vi "squash2016_3.vi"() -> ()   [LabVIEW 2014]
uses:
  <vilib>/vision/Image Controls.llb/IMAQ Image.ctl
  <vilib>/Utility/file.llb/Read From Spreadsheet File (string).vi
  <vilib>/Utility/file.llb/Read From Spreadsheet File (I64).vi
panel:
  in  "Forehand disp 2":bool
  in  "Backhand disp 2":bool
  in  "Cross disp 2":bool
  in  "Bounce disp 2":bool
  in  "Straight disp 2":bool
  in  "volley disp 2":bool
  in  "halfvolley disp 2":bool
  in  "halfvolley disp 1":bool
  in  "volley disp 1":bool
  in  "Straight disp 1":bool
  in  "Bounce disp 1":bool
  in  "Cross disp 1":bool
  in  "Backhand disp 1":bool
  in  "Forehand disp 1":bool
  in  "Let disp 2":bool
  in  "Nolet2 disp":bool
  in  "Stroke2 disp":bool
  in  "Unforced Error2 disp":bool
  in  "Forced Error2 disp":bool
  in  "Unexpected Winner2 disp":bool
  in  "Expected Winner2 disp":bool
  in  "Let disp":bool
  in  "Nolet1 disp":bool
  in  "Stroke1 disp":bool
  in  "Unforced Error1 disp":bool
  in  "Forced Error1 disp":bool
  in  "Unexpected Winner1 disp":bool
  in  "Expected Winner1 disp":bool
  in  "Adrive disp 2":bool
  in  "Smash disp 2":bool
  in  "DSWdrive disp 2":bool
  in  "Lob disp 2":bool
  in  "ASWdrive disp 2":bool
  in  "Ddrive disp 2":bool
  in  "Chop disp 2":bool
  in  "Drop disp 2":bool
  in  "Boast2 disp 2":bool
  in  "Boast3 disp 2":bool
  in  "Stringdisp 2":string
  in  "Adrive disp":bool
  in  "Smash disp":bool
  in  "DSWdrive disp":bool
  in  "Lob disp":bool
  in  "ASWdrive disp":bool
  in  "Ddrive disp":bool
  in  "Chop disp":bool
  in  "Drop disp":bool
  in  "Boast2 disp":bool
  in  "Boast3 disp":bool
  in  "Stringdisp":string
  out "last saved data":i64[](array[numeric])
  out "Btn 10":string
  out "Btn 9":string
  out "Btn 8":string
  out "Btn 7":string
  out "Btn 6":string
  out "subarray":i64[](array[numeric])
  out "output array":i64[][](array[numeric])
  out "appended array":i64[](array[numeric])
  out "0, 1":i16[](array[numeric])
  in  "REPORT":bool
  out "Player 2 data":i64[](array[numeric])
  out "player 1 data":i64[](array[numeric])
  out "both player data":i64[](array[numeric])
  out "Edited data":i64[][](array[numeric])
  out "Event After":i64[][](array[numeric])
  out "Event before":i64[][](array[numeric])
  out "result":i32[](array[numeric])
  out "EVENTS\nTO PLAY":i32[](array[numeric])
  out "Combined data":i64[][](array[numeric])
  out "Extra":i16
  out "Score change":bool[](array[boolean])
  out "last row":i32[](array[numeric])
  out "Player 1/2":i16
  out "Service":i16
  out "Cross":i16
  out "Straight":i16
  out "position":i16
  out "Main tab 2":T1(ring)
  in  "fast rewind":bool
  out "refnum of data save file":refnum<file>
  in  "START":bool
  out "frames to write":i64[][](array[numeric])
  in  "Data file":path=path "C:/Users/KoKuM/Desktop/Current work/ISN/SQUASH/testdata/test2.xls" caption="Data"
  in  "playback speed":dbl(slide)=1.0 min=0.25 max=1.5 step=0.25 scale=0.25..1.5
  in  "Main tab":enum32{"Coding", "Display"}(tab)
  in  "Boast 10":bool
  in  "Boast 12":bool
  in  "Boast 9":bool
  in  "Boast 11":bool
  in  "Smash 12":bool
  in  "Smash 11":bool
  in  "Smash 10":bool
  in  "Smash 9":bool
  in  "lob 12":bool
  in  "Drop 12":bool
  in  "lob 11":bool
  in  "Drop 11":bool
  in  "lob 10":bool
  in  "Drop 10":bool
  in  "lob 9":bool
  in  "Drop 9":bool
  in  "Chop 12":bool
  in  "Chop 11":bool
  in  "Chop 10":bool
  in  "Chop 9":bool
  in  "Smash 8":bool
  in  "Smash 7":bool
  in  "Smash 6":bool
  in  "Smash 5":bool
  in  "Smash":bool
  in  "Smash 2":bool
  in  "Smash 3":bool
  in  "Smash 4":bool
  in  "Chop 8":bool
  in  "Chop 7":bool
  in  "Chop 6":bool
  in  "Chop 5":bool
  in  "Chop":bool
  in  "Chop 2":bool
  in  "Chop 3":bool
  in  "Chop 4":bool
  in  "Boast 7":bool
  in  "Boast 5":bool
  in  "Boast 3":bool
  in  "Boast":bool
  in  "lob 8":bool
  in  "Drop 8":bool
  in  "Boast 6":bool
  in  "lob 7":bool
  in  "Drop 7":bool
  in  "lob 6":bool
  in  "Drop 6":bool
  in  "Boast 8":bool
  in  "lob 5":bool
  in  "Drop 5":bool
  in  "lob 13":bool
  in  "Drop":bool
  in  "Boast 2":bool
  in  "lob 2":bool
  in  "Drop 2":bool
  in  "lob 3":bool
  in  "Drop 3":bool
  in  "Boast 4":bool
  in  "lob 4":bool
  in  "Drop 4":bool
  in  "Let":bool
  in  "Nolet1":bool
  in  "Nolet2":bool
  in  "Stroke1":bool
  in  "Stroke2":bool
  in  "Expected Winner1":bool
  in  "Expected Winner2":bool
  in  "Unexpected Winner1":bool
  in  "Unexpected Winner2":bool
  in  "Forced Error1":bool
  in  "Unforced Error1":bool
  in  "Forced Error2":bool
  in  "Unforced Error2":bool
  in  "Pause lag(s)":dbl=1.0 min=0.0 max=2.0 step=0.5 format="%#.1g"
  in  "Code lag(s)":dbl=1.0 min=0.0 max=5.0 step=0.5 format="%#.1g"
  in  "Link Errors":bool
  in  "Btn 1":string
  in  "Btn 2":string
  in  "Btn 3":string
  in  "Btn 4":string
  in  "Btn 5":string
  in  "Button 1":bool
  in  "Button 2":bool
  in  "Button 3":bool
  in  "Button 4":bool
  in  "Button 5":bool
  out "P2":i32
  out "P1":i32
  out "Player1/Player2":bool[](array[boolean])
  in  "S6":bool
  in  "S5":bool
  in  "S4":bool
  in  "S3":bool
  in  "S2":bool
  in  "Service1":bool
  in  "Service2":bool
  in  "S1":bool
  in  "Player2":bool
  in  "Player1":bool
  in  "Auto switch":bool
  in  "5 4":bool
  in  "5 3":bool
  in  "5 2":bool
  in  "5 1":bool
  in  "6 4":bool
  in  "6 3":bool
  in  "6 2":bool
  in  "6 1":bool
  in  "4 4":bool
  in  "4 3":bool
  in  "4 2":bool
  in  "4 1":bool
  in  "3 4":bool
  in  "3 3":bool
  in  "3 2":bool
  in  "3 1":bool
  in  "2 4":bool
  in  "2 3":bool
  in  "2 2":bool
  in  "2 1":bool
  in  "1 4":bool
  in  "1 3":bool
  in  "1 2":bool
  in  "1 1":bool
  in  "after 2":u8(slide)=2 scale=0.0..5.0
  in  "before 2":u8(slide)=2
  in  "Pause lag on":bool
  in  "SWDrive hide":bool
  in  "SWADrive 12":bool
  in  "SWADrive 11":bool
  in  "SWADrive 10":bool
  in  "SWADrive 9":bool
  in  "SWDDrive 12":bool
  in  "SWDDrive 11":bool
  in  "SWDDrive 10":bool
  in  "SWDDrive 9":bool
  in  "ADrive 12":bool
  in  "ADrive 11":bool
  in  "ADrive 10":bool
  in  "ADrive 9":bool
  in  "DDrive 12":bool
  in  "DDrive 11":bool
  in  "DDrive 10":bool
  in  "DDrive 9":bool
  in  "DDrive 8":bool
  in  "DDrive 7":bool
  in  "DDrive 6":bool
  in  "DDrive 5":bool
  in  "DDrive":bool
  in  "DDrive 2":bool
  in  "DDrive 3":bool
  in  "DDrive 4":bool
  in  "ADrive 8":bool
  in  "ADrive 7":bool
  in  "ADrive 6":bool
  in  "ADrive 5":bool
  in  "ADrive":bool
  in  "ADrive 2":bool
  in  "ADrive 3":bool
  in  "ADrive 4":bool
  in  "SWDDrive 8":bool
  in  "SWDDrive 7":bool
  in  "SWDDrive 6":bool
  in  "SWDDrive 5":bool
  in  "SWDDrive":bool
  in  "SWDDrive 2":bool
  in  "SWDDrive 3":bool
  in  "SWDDrive 4":bool
  in  "SWADrive 8":bool
  in  "SWADrive 7":bool
  in  "SWADrive 6":bool
  in  "SWADrive 5":bool
  in  "SWADrive":bool
  in  "SWADrive 2":bool
  in  "SWADrive 3":bool
  in  "SWADrive 4":bool
  in  "Drive hide":bool
  in  "Undo":bool
  in  "Display tab":enum32{"Edit ", "Data Display"}(tab)
  in  "Extract data":bool
  in  "Upload edited video":bool
  in  "1 10":bool
  in  "1 7":bool
  in  "1 6":bool
  in  "1 5":bool
  in  "2 10":bool
  in  "2 7":bool
  in  "2 6":bool
  in  "2 5":bool
  in  "3 9":bool
  in  "3 7":bool
  in  "3 6":bool
  in  "3 5":bool
  in  "4 9":bool
  in  "4 7":bool
  in  "4 6":bool
  in  "4 5":bool
  in  "Boast3":bool
  in  "Boast2":bool
  in  "Drop 14":bool
  in  "Chop 13":bool
  in  "Ddrive":bool
  in  "Adrive":bool
  in  "ASWdrive":bool
  in  "Lob":bool
  in  "DSWdrive":bool
  in  "Smash 13":bool
  in  "FH":bool
  in  "BH":bool
  in  "ST":bool
  in  "CR":bool
  in  "Bounce":bool
  in  "Half Volley":bool
  in  "Volley":bool
  in  "before":u8(slide)=2
  in  "after":u8(slide)=2 scale=0.0..5.0
  in  "Combine":bool
  in  "Player2 2":bool
  in  "Player1 2":bool
  in  "S6 2":bool
  in  "S5 2":bool
  in  "S4 2":bool
  in  "S1 2":bool
  in  "Service2 2":bool
  in  "Service1 2":bool
  in  "S2 2":bool
  in  "S3 2":bool
  in  "Let 2":bool
  in  "Nolet2 2":bool
  in  "Nolet1 2":bool
  in  "Stroke2 2":bool
  in  "Stroke1 2":bool
  in  "Unforced Error2 2":bool
  in  "Forced Error2 2":bool
  in  "Unforced Error1 2":bool
  in  "Forced Error1 2":bool
  in  "Unexpected Winner2 2":bool
  in  "Unexpected Winner1 2":bool
  in  "Expected Winner2 2":bool
  in  "Expected Winner1 2":bool
  out "Video files to write":string[](array[string])
  in  "Video compress":bool=TRUE
  in  "Abort":bool
  in  "Write file":bool
  in  "Delete":bool[](array[boolean])
  out "Writing":u32(slide) scale=0.0..404.0
  in  "File name":string
  in  "Add to lib":bool
  in  "Video to write":path caption="Folder"
  in  "Examine code":bool
  in  "Update":bool
  in  "Reset":bool
  in  "Code number display":i32 min=1 max=1
  in  "Next":bool
  in  "Previous":bool
  in  "6 5":bool
  in  "6 6":bool
  in  "6 7":bool
  in  "6 8":bool
  in  "5 5":bool
  in  "5 6":bool
  in  "5 7":bool
  in  "5 8":bool
  in  "Button 7":bool
  in  "Button 8":bool
  in  "Button 9":bool
  in  "Button 10":bool
  in  "Button 6":bool
  in  "playback interval on":bool
  in  "Player 2 shots":string[](array[string])=["Att drive", "Def drive", "Att SW drive", "Def SW drive", "", "Drop", "Chop", "Lob", "Boast 2", "Boast 3", "Smash", "", "F-hand", "B-hand", "", "Straight", "Cross", "", "Bounce", "Volley", "H-volley"]
  out "FH 2":u8(slide) scale=0.0..2.0
  out "BH 2":u8(slide) scale=0.0..2.0
  out "Straight 2":u8(slide) scale=0.0..2.0
  out "Cross 2":u8(slide) scale=0.0..2.0
  out "Bounce 2":u8(slide) scale=0.0..2.0
  out "Volley 2":u8(slide) scale=0.0..2.0
  out "Drive 2":u8(slide) scale=0.0..2.0
  out "Lob 2":u8(slide) scale=0.0..2.0
  out "Drop 13":u8(slide) scale=0.0..2.0
  out "Boast 13":u8(slide) scale=0.0..2.0
  out "Player 2 shots numbers":string[](array[string])=["0", "0", "0", "0", "", " ", "0", "0", "", "0", "0", "", "0", "0"]
  in  "Fh 2":string="Forehand"
  in  "BH 4":string="Backhand"
  in  "Cross 6":string="Cross"
  in  "bounce 2":string="Bounce"
  in  "Straight 6":string="Straight"
  in  "volley 2":string="Volley"
  in  "H-volley 2":string="Half volley"
  out "F-hand 2":string="0"
  out "B-hand 2":string="0"
  out "Cross 3":string="0"
  out "Bounce 3":string="0"
  out "Straight 3":string="0"
  out "Volley 3":string="0"
  out "H-volley 3":string="0"
  in  "No let 2":string="No let"
  in  "Let  5":string="Let"
  in  "Stroke 2":string="Stroke"
  out "No Let 2":string="0"
  out "Let 4":string="0"
  out "Stroke 4":string="0"
  in  "ex win2":string="Expected \nwinner"
  in  "UNex win2":string="UNexpected \nwinner"
  in  "F err2":string="Forced \nerror"
  in  "UF err2":string="UNforced \nerror"
  out "ex win2 num":string="0"
  out "UNex win2 num":string="0"
  out "F err2 num":string="0"
  out "UF err2 num":string="0"
  out "4 42":dbl
  out "4 32":dbl
  out "4 22":dbl
  out "4 12":dbl
  out "3 42":dbl
  out "3 32":dbl
  out "3 22":dbl
  out "3 12":dbl
  out "2 42":dbl
  out "2 32":dbl
  out "2 22":dbl
  out "2 12":dbl
  out "1 42":dbl
  out "1 32":dbl
  out "1 22":dbl
  out "1 12":dbl
  in  "H-volley":string="Half volley"
  in  "volley":string="Volley"
  in  "Straight 5":string="Straight"
  in  "bounce":string="Bounce"
  in  "Cross 5":string="Cross"
  in  "BH 3":string="Backhand"
  in  "Fh":string="Forehand"
  in  "No let 1":string="No let"
  in  "Let 1":string="Let "
  in  "Stroke 1":string="Stroke"
  out "No Let 1":string="0"
  out "Let 3":string="0"
  out "Stroke 3":string="0"
  in  "ex win1":string="Expected \nwinner"
  in  "UNex win1":string="Unexpected \nwinner"
  in  "F err1":string="Forced \nerror"
  in  "UF err1":string="UNforced \nerror"
  out "ex win1 num":string="0"
  out "UNex win1 num":string="0"
  out "F err1 num":string="0"
  out "UF err1 num":string="0"
  out "1 14":dbl
  out "1 13":dbl
  out "1 11":dbl
  out "1 9":dbl
  out "2 14":dbl
  out "2 13":dbl
  out "2 11":dbl
  out "2 9":dbl
  out "3 13":dbl
  out "3 11":dbl
  out "3 10":dbl
  out "3 8":dbl
  out "4 13":dbl
  out "4 11":dbl
  out "4 10":dbl
  out "4 8":dbl
  out "H-volley 1":string="0"
  out "F-hand 1":string="0"
  out "B-hand 1":string="0"
  out "Cross 1":string="0"
  out "Bounce 1":string="0"
  out "Straight 1":string="0"
  out "Volley 1":string="0"
  in  "Player 1 shots":string[](array[string])=["Att drive", "Def drive", "Att SW drive", "Def SW drive", "", "Drop", "Chop", "Lob", "Boast 2", "Boast 3", "Smash", "", "F-hand", "B-hand", "", "Straight", "Cross", "", "Bounce", "Volley", "H-volley"]
  out "FH 1":u8(slide) scale=0.0..2.0
  out "BH 1":u8(slide) scale=0.0..2.0
  out "Straight 4":u8(slide) scale=0.0..2.0
  out "Cross 4":u8(slide) scale=0.0..2.0
  out "Bounce 4":u8(slide) scale=0.0..2.0
  out "Volley 4":u8(slide) scale=0.0..2.0
  out "Drive 1":u8(slide) scale=0.0..2.0
  out "Lob 1":u8(slide) scale=0.0..2.0
  out "Drop 1":u8(slide) scale=0.0..2.0
  out "Boast 1":u8(slide) scale=0.0..2.0
  out "Player 1 shots numbers":string[](array[string])=["0", "0", "0", "0", "", " ", "0", "0", "", "0", "0", "", "0", "0"]
  in  "display\nselection":string(combo)="1"
  out "5 14":dbl
  out "5 23":dbl
  out "5 33":dbl
  out "5 43":dbl
  out "6 15":dbl
  out "6 24":dbl
  out "6 34":dbl
  out "6 44":dbl
  out "5 18":dbl
  out "5 15":dbl
  out "5 16":dbl
  out "5 17":dbl
  out "6 18":dbl
  out "6 19":dbl
  out "6 20":dbl
  out "6 21":dbl
  in  "Load video":bool
  in  "Play":bool
  out "ful video frames":i64[](array[numeric])
  out "playback speed":dbl
  out "Number of Frames":u32
  out "framesPerSecond":u32
  out "Last Edit":bool[](array[boolean])
  out "frames 2 play":i64[](array[numeric])
  in  "stop":bool
  out "Video Frame":u32
  out "edited\nevents":i64[][](array[numeric])
  out "edited to play":i64[](array[numeric])
  out "frames edited":i64[](array[numeric])
  in  "fast forward":bool
  in  "Pause":bool
  out "coding":i64[][](array[numeric])
  in  "Progress...":u32(slide) min=400 max=47374 scale=-1.1..130372.0
  in  "Video file":path=path "C:/Users/KoKuM/Desktop/Current work/ISN/SQUASH/testdata/WWC16_FIN_w1.avi" caption="Video"
  out "task":i32(slide) scale=0.0..300.0
  out "Video":T2(plugin-control)
  # "Playback interval (s)"
  # "© 2016 National Sports Institute of Malaysia All Rights Reserved"
  # "Position"
  # "Drop"
  # "Chop"
  # "Lob"
  # "Boast"
  # "Smash"
  # "Att"
  # "Def"
  # "Att"
  # "Def"
  # "Half volley"
  # "Forehand"
  # "Backhand"
  # "St"
  # "Cr"
  # "St"
  # "Cr"
  # "Volley"
  # "Forehand"
  # "Backhand"
  # "St"
  # "Cr"
  # "St"
  # "Cr"
  # "Bounce"
  # "Forehand"
  # "Backhand"
  # "St"
  # "Cr"
  # "St"
  # "Cr"
  # "Lead and lag settings"
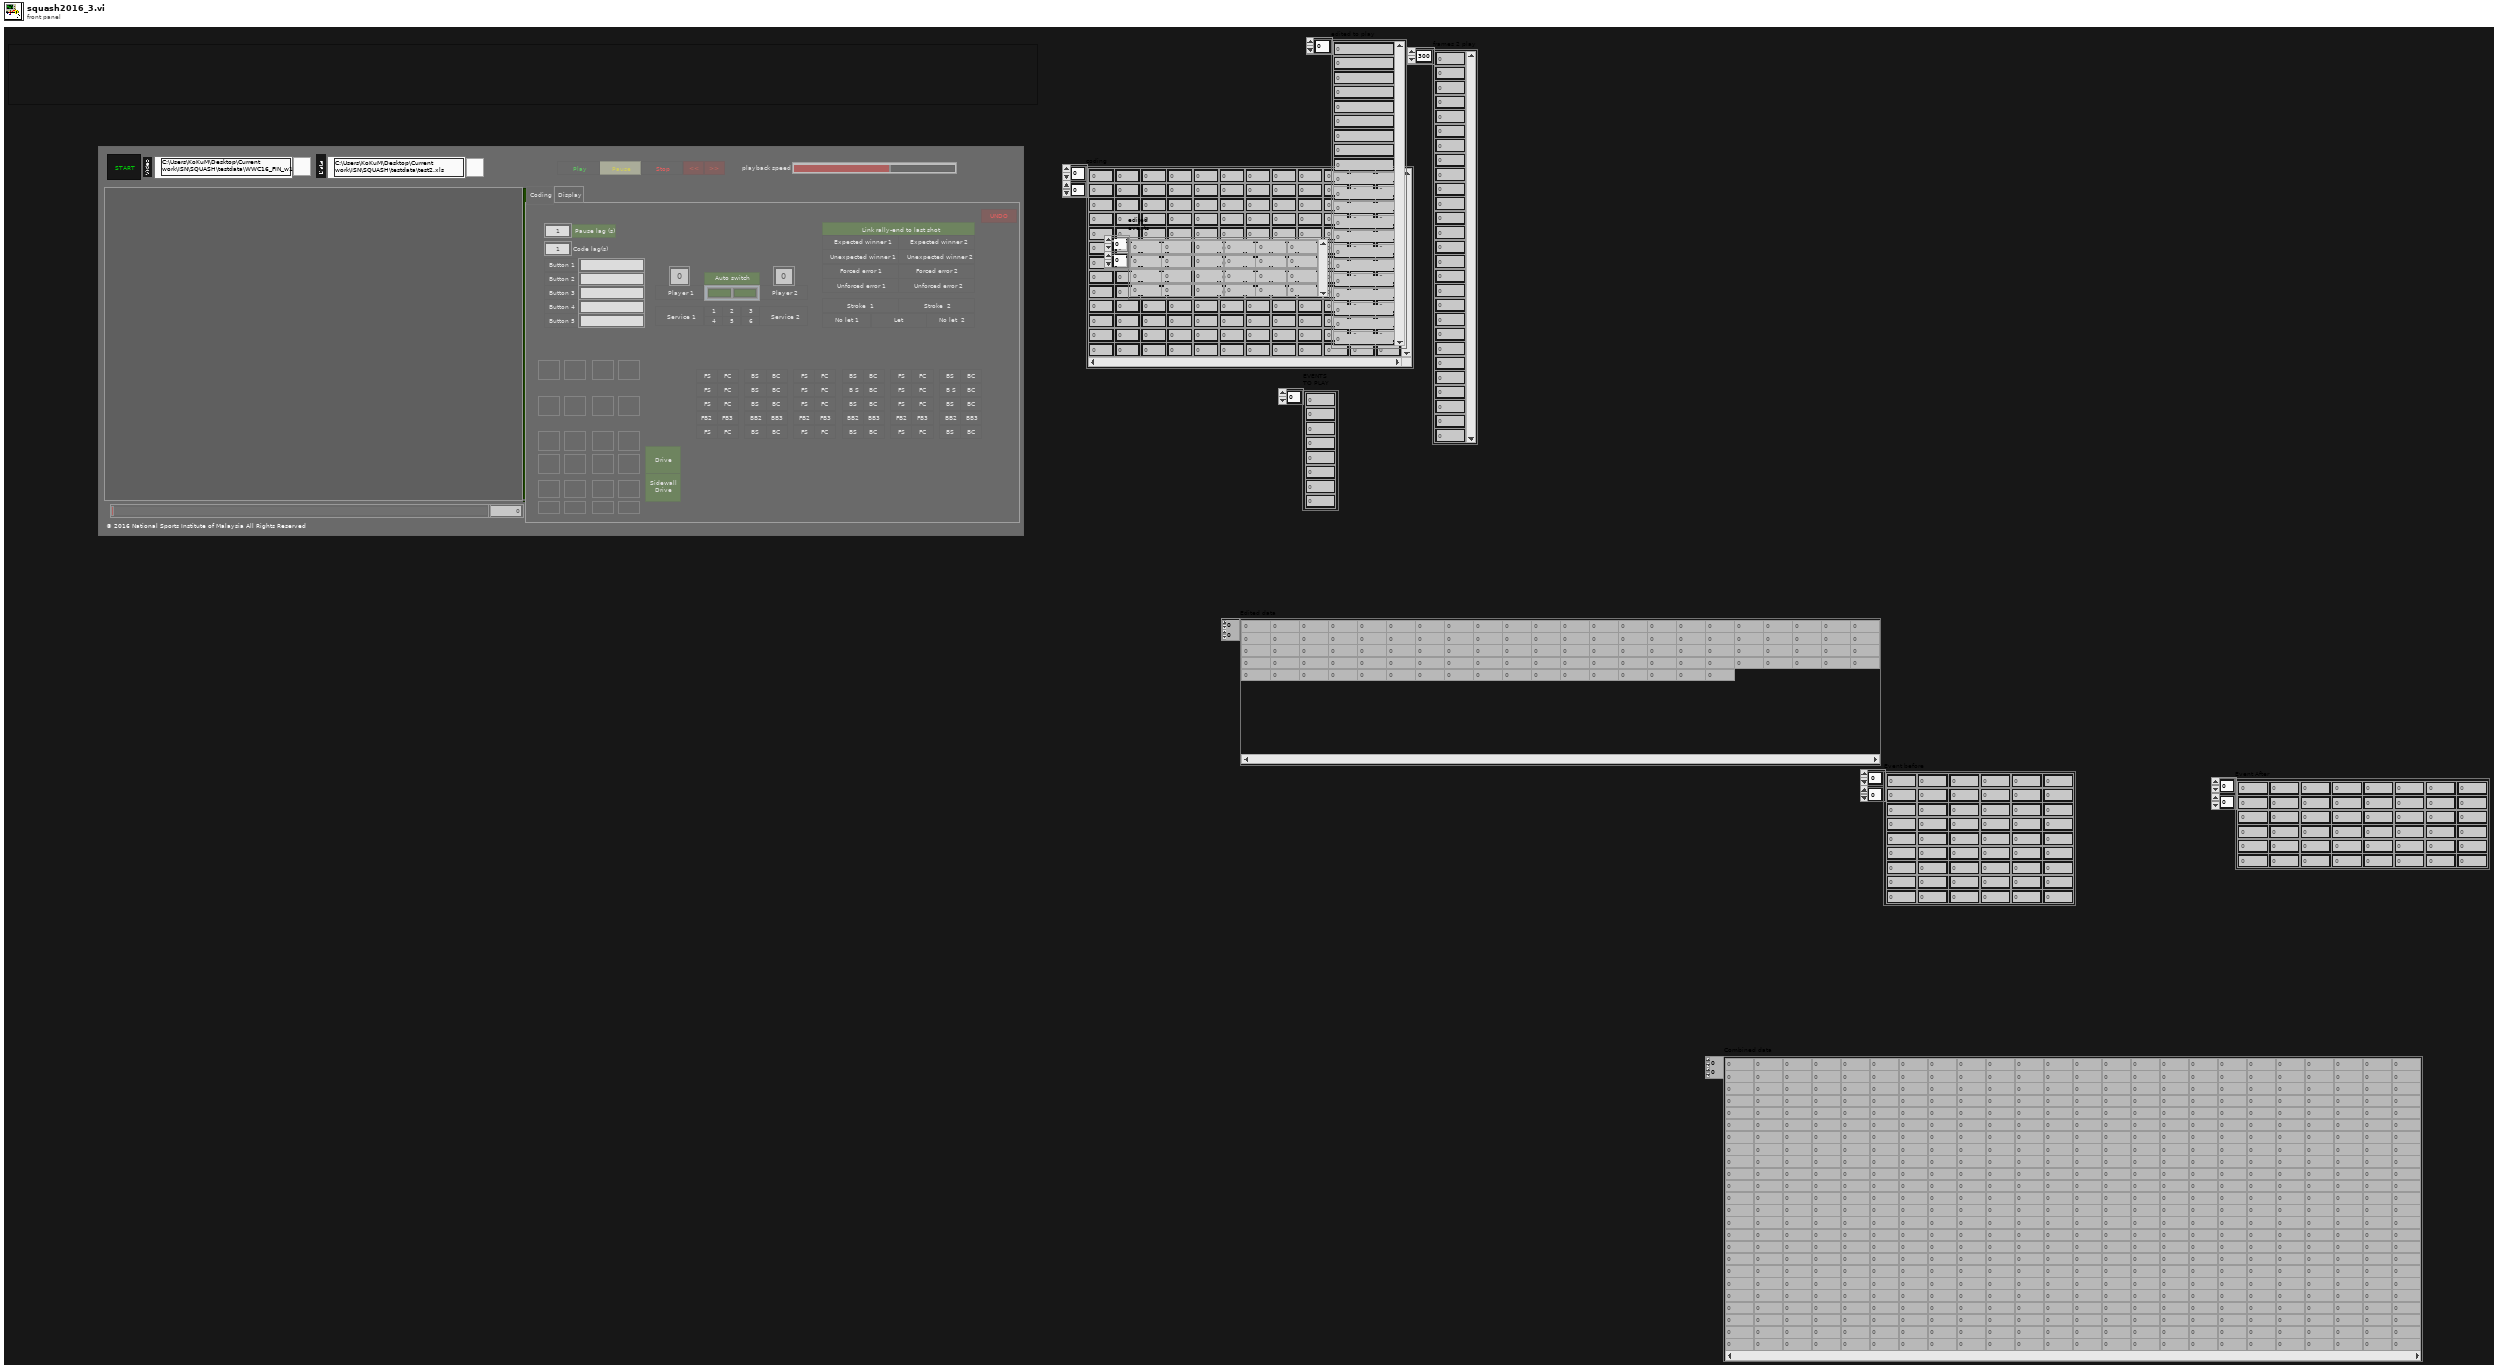
[diagram p1: front panel]
types:
  T1 = enum32{"Coding", "Edit video", "Examine coding", "Display", "Update coding", "Edit coding"}
  T2 = typedef "IMAQ Image.ctl" = refnum<image>
  T3 = enum16{"open", "replace", "create", "open or create", "replace or create", "replace or create with confirmation"}
  T4 = enum8{"Enabled", "Disabled", "Disabled and Grayed Out"}
  T5 = typedef "Image Type" = u32
  T6 = typedef "AviRefnum.ctl" = refnum<k1>
  T7 = cluster{"width":u32, "height":u32, "framesPerSecond":u32, "compressionFilter":string, "hasData":bool}
  T8 = typedef "eventvkey.ctl" = enum16{"ASCII", "Enter", "Return", "Shift", "Ctrl", "Alt", "Cmd", "Opt", "Caps", "NumLock", "Clear", "Break", "Up", "Down", "Left", "Right", "Insert", "Delete", "Home", "End", "PageUp", "PageDown", "Escape", "Help", "Pause", "ScrollLock", "F1", "F2", "F3", "F4", "F5", "F6", "F7", "F8", "F9", "F10", "F11", "F12", "F13", "F14", "F15", "F16", "F17", "F18", "F19", "F20", "F21", "F22", "F23", "F24", "Play", "VolumeUp", "VolumeDown", "Mute", "Two Byte Char"}
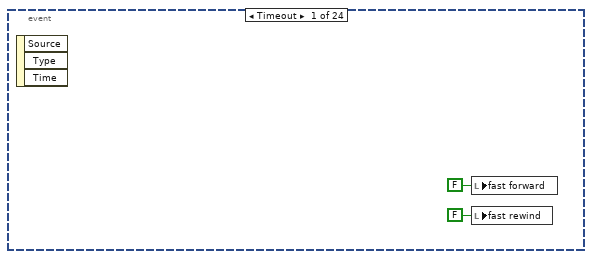
[diagram p3: hidden frame]
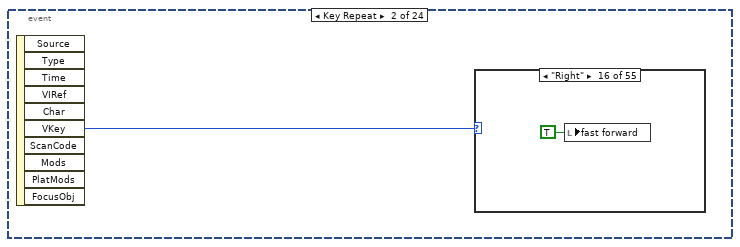
[diagram p4: hidden frame]
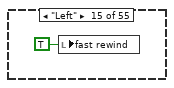
[diagram p19: hidden frame]
diagram:
  n1 = while {
    stop <- FALSE stop-if-true
    n2 = flat-sequence {
      tunnel: [w42] -> w15
      tunnel: [w43] -> w16
      tunnel: w16 -> [w136]
      tunnel: w15 -> [w135]
      tunnel: [w135] -> w14
      tunnel: [w136] -> w13
      tunnel: w14 -> [w176]
      tunnel: w13 -> [w159]
      tunnel: [w175] -> w11
      tunnel: [w158] -> w10
      tunnel: [w157] -> w9
      tunnel: [w156] -> w1
      tunnel: [w155] -> w8
      frame #0 {
        w37 = T4."Enabled" ("Disabled")
        w39 = u32 0 ("Progress...")
        w36 = FALSE ("START")
        w35 = T4."Disabled and Grayed Out" ("Disabled")
        n3 = property on="Play" class="Bool (strict)"("DisabledEnum"=w35, "Value"=w36) -> ()  [unwired: 2 in, 2 out]
        n4 = property on="stop" class="Bool (strict)"("DisabledEnum"=w35, "Value"=w36) -> ()  [unwired: 2 in, 2 out]
        n5 = property on="Pause" class="Bool (strict)"("DisabledEnum"=w35, "Value"=w36) -> ()  [unwired: 2 in, 2 out]
        n6 = property on="fast forward" class="Bool (strict)"("DisabledEnum"=w35, "Value"=w36) -> ()  [unwired: 2 in, 2 out]
        n7 = property on="playback speed" class="Slide (strict)"("DisabledEnum"=w35, "Value"=1.0 ("playback speed")) -> ()  [unwired: 2 in, 2 out]
        n8 = property on="Main tab" class="TabCtl (strict)"("DisabledEnum"=w35, "Value"=enum32{"Coding", "Display"}."Coding" ("Main tab")) -> ()  [unwired: 2 in, 2 out]
        n9 = property on="Progress..." class="Slide (strict)"("DisabledEnum"=w35, "Value"=w39) -> ()  [unwired: 2 in, 2 out]
        n10 = property on="Video Frame" class="DigNum (strict)"("DisabledEnum"=w35, "Value"=w39) -> ()  [unwired: 2 in, 2 out]
        n11 = property on="Video" class="ImageControl"("DisabledEnum"=w35, "Value"=T2 refnum ("Video")) -> ()  [unwired: 2 in, 2 out]
        n12 = property on="START" class="Bool (strict)"("DisabledEnum"=w37, "Value"=w36) -> ()  [unwired: 2 in, 2 out]
        n13 = property on="Video file" class="Path"("DisabledEnum"=w37) -> ()  [unwired: 2 in, 2 out]
        n14 = property on="Data file" class="Path"("DisabledEnum"=w37) -> ()  [unwired: 2 in, 2 out]
        n15 = property on="fast rewind" class="Bool (strict)"("DisabledEnum"=w35, "Value"=w36) -> ()  [unwired: 2 in, 2 out]
      }
      frame #1 {
        n16 = while {
          tunnel: [w45] -> w43
          tunnel: [w44] -> w42
          stop <- w46 stop-if-true
          n17 = case shown="True" "START" {
            tunnel: [FALSE w51] -> w46
            tunnel: [w48 w54] -> w45
            tunnel: [w48 w53] -> w44
            frame False {
              w48 = path "" ("dup path")
              n18 = Wait (ms)(milliseconds to wait=u32 200) -> ()  [unwired: 1 out]
            }
            frame True {
              n19 = Path To String(path="Data file") -> (string=w63:string)
              n20 = Wait (ms)(milliseconds to wait=u32 200) -> ()  [unwired: 1 out]
              n21 = Empty String/Path?(string/path=w63) -> (empty?=w62:bool)
              n22 = case shown="False" w62 {
                tunnel: "Data file" -> [w84 w109]
                tunnel: [w83 FALSE] -> w60
                tunnel: [w82 w109] -> w53
                frame False {
                  n23 = Strip Path(path=w84) -> (stripped path=w89:path)  [unwired: 1 out]
                  n24 = Path To String(path=w89) -> (string=w88:string)
                  n25 = call <vilib>:"Get File Extension.vi"("file"=w84) -> ("filename without extension"=w91:string)  [unwired: 7 in, 3 out]
                  n26 = Concatenate Strings(w88, "\\" ("string"), w91, ".xls" ("string")) -> (w90:string)
                  n27 = String To Path(string=w90) -> (path=w85:path)
                  n28 = call <vilib>:"Check if File or Folder Exists.vi"("path"=w85) -> ("file or folder exists?"=w86:bool)  [unwired: 8 in, 2 out]
                  n29 = case shown="True" w86 {
                    selector: w86 -> [_ w108]
                    tunnel: w85 -> [w95 w107]
                    tunnel: [w94 w108] -> w83
                    tunnel: [w93 w107] -> w82
                    frame False {
                      n30 = Two Button Dialog(message="This data file does not exist.\nDo you wish to start a new project?", 1:"No" ("F button name (\"Cancel\")"), 2:"Yes" ("T button name (\"OK\")")) -> (T button?=w96:bool)
                      n31 = case shown="False" w96 {
                        selector: w96 -> [w101 w103]
                        tunnel: w95 -> [_ w102]
                        tunnel: [w101 w103] -> w94
                        tunnel: [path "" ("dup path") w102] -> w93
                        frame False {
                        }
                        frame True {
                          n32 = Open/Create/Replace File(file path (use dialog)=w102, operation (0:open)=T3."create") -> (refnum out=w104:refnum<file>, error out=w106:errorcluster)  [unwired: 4 in, 1 out]
                          n33 = Close File(refnum=w104, error in=w106) -> ()  [unwired: 2 out]
                        }
                      }
                    }
                    frame True {
                    }
                  }
                }
                frame True {
                  n34 = One Button Dialog(message="Please enter data file") -> ()  [unwired: 1 in, 1 out]
                }
              }
              n35 = Path To String(path="Video file") -> (string=w58:string)
              n36 = Empty String/Path?(string/path=w58) -> (empty?=w57:bool)
              n37 = case shown="True" w57 {
                selector: w57 -> [_ w81]
                tunnel: "Video file" -> [w68 w79]
                tunnel: [w65 w79] -> w54
                tunnel: [w64 w81] -> w55
                frame False {
                  n38 = call <vilib>:"Check if File or Folder Exists.vi"("path"=w68) -> ("file or folder exists?"=w72:bool, "dup path"=w66:path)  [unwired: 8 in, 1 out]
                  n39 = call <vilib>:"Get File Extension.vi"("file"=w68) -> ("lowercase file extension"=w69:string)  [unwired: 7 in, 3 out]
                  n40 = Not(x=w72) -> (.not. x?=w73:bool)
                  n41 = Not Equal?(x=w69, y="avi" ("lowercase file extension")) -> (x != y?=w71:bool)
                  n42 = Or(x=w73, y=w71) -> (x .or. y?=w67:bool)
                  n43 = case shown="True" w67 {
                    selector: w67 -> [w74 w76]
                    tunnel: w66 -> [w75 _]
                    tunnel: [w75 path "" ("dup path")] -> w65
                    tunnel: [w74 w76] -> w64
                    frame False {
                    }
                    frame True {
                      n44 = One Button Dialog(message="You have chosen an invalid video file for coding\n\nPossible reasons\n1)\tChosen video file format was not AVI\n2)\tChosen video file does not exist") -> ()  [unwired: 1 in, 1 out]
                    }
                  }
                }
                frame True {
                  n45 = One Button Dialog(message="Please enter video file") -> ()  [unwired: 1 in, 1 out]
                }
              }
              n46 = Not(x=w55) -> (.not. x?=w59:bool)
              n47 = local write "Video file"(w54) -> ()
              n48 = And(x=w59, y=w60) -> (x .and. y?=w51:bool)
              n49 = local write "Data file"(w53) -> ()
              n50 = local write "START"(w51) -> ()
            }
          }
        }
      }
      frame #2 {
        w114 = FALSE ("Combine")
        w113 = i64[] [] ("to write")
        w131 = 0 ("P1")
        w116 = FALSE ("4 6")
        w115 = TRUE ("4 6")
        w151 = FALSE ("4 6")
        w149 = TRUE ("Extract data")
        w117 = u8 2 ("before")
        w134 = T4."Disabled and Grayed Out" ("Disabled")
        w154 = u32 0 ("Progress...")
        w137 = FALSE ("START")
        w138 = T4."Enabled" ("Disabled")
        n51 = property on="Play" class="Bool (strict)"("DisabledEnum"=w138, "Value"=w137) -> ()  [unwired: 2 in, 2 out]
        n52 = property on="stop" class="Bool (strict)"("DisabledEnum"=w138, "Value"=w137) -> ()  [unwired: 2 in, 2 out]
        n53 = property on="Pause" class="Bool (strict)"("DisabledEnum"=w138, "Value"=w137) -> ()  [unwired: 2 in, 2 out]
        n54 = property on="fast forward" class="Bool (strict)"("DisabledEnum"=w138, "Value"=w137) -> ()  [unwired: 2 in, 2 out]
        n55 = property on="fast rewind" class="Bool (strict)"("DisabledEnum"=w138, "Value"=w137) -> ()  [unwired: 2 in, 2 out]
        n56 = property on="playback speed" class="Slide (strict)"("DisabledEnum"=w138, "Value"=1.0 ("playback speed")) -> ()  [unwired: 2 in, 2 out]
        n57 = property on="Main tab" class="TabCtl (strict)"("DisabledEnum"=w138, "Value"=enum32{"Coding", "Display"}."Coding" ("Main tab")) -> ()  [unwired: 2 in, 2 out]
        n58 = property on="Progress..." class="Slide (strict)"("DisabledEnum"=w138, "Value"=w154) -> ()  [unwired: 2 in, 2 out]
        n59 = property on="Video Frame" class="DigNum (strict)"("DisabledEnum"=w138, "Value"=w154) -> ()  [unwired: 2 in, 2 out]
        n60 = property on="Video" class="ImageControl"("DisabledEnum"=w138) -> ()  [unwired: 2 in, 2 out]
        n61 = property on="Video file" class="Path"("DisabledEnum"=w134) -> ()  [unwired: 2 in, 2 out]
        n62 = property on="Data file" class="Path"("DisabledEnum"=w134) -> ()  [unwired: 2 in, 2 out]
        n63 = property on="Code number display" class="DigNum (strict)"("DisabledEnum"=w134) -> ()  [unwired: 2 in, 2 out]
        n64 = property on="Next" class="Bool (strict)"("DisabledEnum"=w134) -> ()  [unwired: 2 in, 2 out]
        n65 = property on="Reset" class="Bool (strict)"("DisabledEnum"=w134) -> ()  [unwired: 2 in, 2 out]
        n66 = property on="Update" class="Bool (strict)"("DisabledEnum"=w134) -> ()  [unwired: 2 in, 2 out]
        n67 = property on="Previous" class="Bool (strict)"("DisabledEnum"=w134) -> ()  [unwired: 2 in, 2 out]
        n68 = local write "Pause lag(s)"(1.0 ("Pause lag(s)")) -> ()
        n69 = local write "Code lag(s)"(0.5 ("Code lag(s)")) -> ()
        n70 = local write "Link Errors"(TRUE ("Link Errors")) -> ()
        n71 = local write "SWDrive hide"(w115) -> ()
        n72 = local write "Drive hide"(w115) -> ()
        n73 = local write "Pause lag on"(w115) -> ()
        n74 = local write "playback interval on"(w115) -> ()
        n75 = local write "Auto switch"(w115) -> ()
        n76 = local write "Combine"(w114) -> ()
        n77 = local write "Button 10"(w114) -> ()
        n78 = local write "Undo"(w114) -> ()
        n79 = local write "Button 8"(w114) -> ()
        n80 = local write "Button 9"(w114) -> ()
        n81 = local write "Button 6"(w114) -> ()
        n82 = local write "Button 7"(w114) -> ()
        n83 = local write "Last Edit"(bool[] [FALSE, FALSE, FALSE, FALSE, FALSE, FALSE, FALSE, FALSE, FALSE, FALSE, FALSE, FALSE, FALSE, FALSE, FALSE, FALSE, FALSE, FALSE, FALSE, FALSE, FALSE, FALSE, FALSE, FALSE, FALSE, FALSE, FALSE, FALSE, FALSE, FALSE, FALSE, FALSE, FALSE, FALSE, FALSE, FALSE] ("Last Edit")) -> ()
        n84 = local write "File name"("" ("File name")) -> ()
        n85 = local write "Code number display"(1 ("Code number display")) -> ()
        n86 = local write "Delete"(bool[] [TRUE, TRUE, TRUE, TRUE, TRUE] ("Array 2")) -> ()
        n87 = local write "Video compress"(w149) -> ()
        n88 = local write "Extract data"(w149) -> ()
        n89 = local write "Upload edited video"(w151) -> ()
        n90 = local write "Add to lib"(w151) -> ()
        n91 = local write "Abort"(w151) -> ()
        n92 = local write "Write file"(w151) -> ()
        n93 = local write "REPORT"(w151) -> ()
        n94 = local write "Examine code"(w151) -> ()
        n95 = local write "Update"(w151) -> ()
        n96 = local write "Reset"(w151) -> ()
        n97 = local write "Previous"(w151) -> ()
        n98 = local write "Next"(w151) -> ()
        n99 = local write "before"(w117) -> ()
        n100 = local write "after"(w117) -> ()
        n101 = local write "before 2"(w117) -> ()
        n102 = local write "after 2"(w117) -> ()
        n103 = call-poly <vilib>:"Read From Spreadsheet File.vi"("file path (dialog if empty)"=w135) -> ("all rows"=w123:string[][])  [unwired: 6 in, 4 out]
        n104 = Index Array(array=w123, index (row)=3) -> (element=w125:string[])  [unwired: 1 in]
        n105 = Index Array(array=w125, index #1=71 ("index"), index #2=72 ("index"), index #3=73 ("index"), index #4=74 ("index"), index #5=75 ("index")) -> (element #1=w120:string, element #2=w121:string, element #3=w122:string, element #4=w119:string, element #5=w118:string)
        n106 = local write "display\nselection"("1" ("display\nselection")) -> ()
        n107 = local write "task"(300 ("task")) -> ()
        n108 = local write "Load video"(FALSE ("Pause")) -> ()
        n109 = local write "Video files to write"(string[] [] ("Video files to write")) -> ()
        n110 = local write "frames to write"(i64[][] [] ("to write")) -> ()
        n111 = local write "player 1 data"(w113) -> ()
        n112 = local write "both player data"(w113) -> ()
        n113 = local write "Player 2 data"(w113) -> ()
        n114 = local write "last saved data"(w113) -> ()
        n115 = local write "Btn 1"(w120) -> ()
        n116 = local write "Btn 2"(w121) -> ()
        n117 = local write "Btn 3"(w122) -> ()
        n118 = local write "Btn 4"(w119) -> ()
        n119 = local write "Btn 5"(w118) -> ()
        n120 = local write "P1"(w131) -> ()
        n121 = local write "P2"(w131) -> ()
        n122 = local write "Drop"(w116) -> ()
        n123 = local write "Drop 2"(w116) -> ()
        n124 = local write "Drop 3"(w116) -> ()
        n125 = local write "Drop 4"(w116) -> ()
        n126 = local write "Drop 5"(w116) -> ()
        n127 = local write "Drop 6"(w116) -> ()
        n128 = local write "Drop 7"(w116) -> ()
        n129 = local write "Drop 8"(w116) -> ()
        n130 = local write "Drop 9"(w116) -> ()
        n131 = local write "Drop 10"(w116) -> ()
        n132 = local write "Drop 11"(w116) -> ()
        n133 = local write "Drop 12"(w116) -> ()
        n134 = local write "Chop"(w116) -> ()
        n135 = local write "Chop 2"(w116) -> ()
        n136 = local write "Chop 3"(w116) -> ()
        n137 = local write "Chop 4"(w116) -> ()
        n138 = local write "Chop 5"(w116) -> ()
        n139 = local write "Chop 6"(w116) -> ()
        n140 = local write "Chop 7"(w116) -> ()
        n141 = local write "Chop 8"(w116) -> ()
        n142 = local write "Chop 9"(w116) -> ()
        n143 = local write "Chop 10"(w116) -> ()
        n144 = local write "Chop 11"(w116) -> ()
        n145 = local write "Chop 12"(w116) -> ()
        n146 = local write "Player2 2"(w116) -> ()
        n147 = local write "Player1 2"(w116) -> ()
        n148 = local write "Button 7"(w116) -> ()
        n149 = local write "Button 8"(w116) -> ()
        n150 = local write "Button 9"(w116) -> ()
        n151 = local write "Button 10"(w116) -> ()
        n152 = local write "Button 6"(w116) -> ()
        n153 = local write "S6 2"(w116) -> ()
        n154 = local write "S5 2"(w116) -> ()
        n155 = local write "S4 2"(w116) -> ()
        n156 = local write "S1 2"(w116) -> ()
        n157 = local write "Service2 2"(w116) -> ()
        n158 = local write "Service1 2"(w116) -> ()
        n159 = local write "S2 2"(w116) -> ()
        n160 = local write "S3 2"(w116) -> ()
        n161 = local write "lob 13"(w116) -> ()
        n162 = local write "lob 2"(w116) -> ()
        n163 = local write "lob 3"(w116) -> ()
        n164 = local write "lob 4"(w116) -> ()
        n165 = local write "lob 5"(w116) -> ()
        n166 = local write "lob 6"(w116) -> ()
        n167 = local write "lob 7"(w116) -> ()
        n168 = local write "lob 8"(w116) -> ()
        n169 = local write "lob 9"(w116) -> ()
        n170 = local write "lob 10"(w116) -> ()
        n171 = local write "lob 11"(w116) -> ()
        n172 = local write "lob 12"(w116) -> ()
        n173 = local write "Smash"(w116) -> ()
        n174 = local write "Smash 2"(w116) -> ()
        n175 = local write "Smash 3"(w116) -> ()
        n176 = local write "Smash 4"(w116) -> ()
        n177 = local write "Smash 5"(w116) -> ()
        n178 = local write "Smash 6"(w116) -> ()
        n179 = local write "Smash 7"(w116) -> ()
        n180 = local write "Smash 8"(w116) -> ()
        n181 = local write "Smash 9"(w116) -> ()
        n182 = local write "Smash 10"(w116) -> ()
        n183 = local write "Smash 11"(w116) -> ()
        n184 = local write "Smash 12"(w116) -> ()
        n185 = local write "4 5"(w116) -> ()
        n186 = local write "4 6"(w116) -> ()
        n187 = local write "4 7"(w116) -> ()
        n188 = local write "4 9"(w116) -> ()
        n189 = local write "3 5"(w116) -> ()
        n190 = local write "3 6"(w116) -> ()
        n191 = local write "3 7"(w116) -> ()
        n192 = local write "3 9"(w116) -> ()
        n193 = local write "2 5"(w116) -> ()
        n194 = local write "2 6"(w116) -> ()
        n195 = local write "2 7"(w116) -> ()
        n196 = local write "2 10"(w116) -> ()
        n197 = local write "1 5"(w116) -> ()
        n198 = local write "1 6"(w116) -> ()
        n199 = local write "1 7"(w116) -> ()
        n200 = local write "1 10"(w116) -> ()
        n201 = local write "6 5"(w116) -> ()
        n202 = local write "6 6"(w116) -> ()
        n203 = local write "6 7"(w116) -> ()
        n204 = local write "6 8"(w116) -> ()
        n205 = local write "5 5"(w116) -> ()
        n206 = local write "5 6"(w116) -> ()
        n207 = local write "5 7"(w116) -> ()
        n208 = local write "5 8"(w116) -> ()
        n209 = local write "Half Volley"(w116) -> ()
        n210 = local write "ADrive"(w116) -> ()
        n211 = local write "ADrive 2"(w116) -> ()
        n212 = local write "ADrive 3"(w116) -> ()
        n213 = local write "ADrive 4"(w116) -> ()
        n214 = local write "ADrive 5"(w116) -> ()
        n215 = local write "ADrive 6"(w116) -> ()
        n216 = local write "ADrive 7"(w116) -> ()
        n217 = local write "ADrive 8"(w116) -> ()
        n218 = local write "ADrive 9"(w116) -> ()
        n219 = local write "ADrive 10"(w116) -> ()
        n220 = local write "ADrive 11"(w116) -> ()
        n221 = local write "ADrive 12"(w116) -> ()
        n222 = local write "DDrive"(w116) -> ()
        n223 = local write "DDrive 2"(w116) -> ()
        n224 = local write "DDrive 3"(w116) -> ()
        n225 = local write "DDrive 4"(w116) -> ()
        n226 = local write "DDrive 5"(w116) -> ()
        n227 = local write "DDrive 6"(w116) -> ()
        n228 = local write "DDrive 7"(w116) -> ()
        n229 = local write "DDrive 8"(w116) -> ()
        n230 = local write "DDrive 9"(w116) -> ()
        n231 = local write "DDrive 10"(w116) -> ()
        n232 = local write "DDrive 11"(w116) -> ()
        n233 = local write "DDrive 12"(w116) -> ()
        n234 = local write "Smash 13"(w116) -> ()
        n235 = local write "Boast3"(w116) -> ()
        n236 = local write "DSWdrive"(w116) -> ()
        n237 = local write "Lob"(w116) -> ()
        n238 = local write "ASWdrive"(w116) -> ()
        n239 = local write "Adrive"(w116) -> ()
        n240 = local write "Ddrive"(w116) -> ()
        n241 = local write "Chop 13"(w116) -> ()
        n242 = local write "Drop 14"(w116) -> ()
        n243 = local write "Boast2"(w116) -> ()
        n244 = local write "FH"(w116) -> ()
        n245 = local write "BH"(w116) -> ()
        n246 = local write "ST"(w116) -> ()
        n247 = local write "CR"(w116) -> ()
        n248 = local write "Bounce"(w116) -> ()
        n249 = local write "Volley"(w116) -> ()
        n250 = local write "SWADrive"(w116) -> ()
        n251 = local write "SWADrive 2"(w116) -> ()
        n252 = local write "SWADrive 3"(w116) -> ()
        n253 = local write "SWADrive 4"(w116) -> ()
        n254 = local write "SWADrive 5"(w116) -> ()
        n255 = local write "SWADrive 6"(w116) -> ()
        n256 = local write "SWADrive 7"(w116) -> ()
        n257 = local write "SWADrive 8"(w116) -> ()
        n258 = local write "SWADrive 9"(w116) -> ()
        n259 = local write "SWADrive 10"(w116) -> ()
        n260 = local write "SWADrive 11"(w116) -> ()
        n261 = local write "SWADrive 12"(w116) -> ()
        n262 = local write "SWDDrive"(w116) -> ()
        n263 = local write "SWDDrive 2"(w116) -> ()
        n264 = local write "SWDDrive 3"(w116) -> ()
        n265 = local write "SWDDrive 4"(w116) -> ()
        n266 = local write "SWDDrive 5"(w116) -> ()
        n267 = local write "SWDDrive 6"(w116) -> ()
        n268 = local write "SWDDrive 7"(w116) -> ()
        n269 = local write "SWDDrive 8"(w116) -> ()
        n270 = local write "SWDDrive 9"(w116) -> ()
        n271 = local write "SWDDrive 10"(w116) -> ()
        n272 = local write "SWDDrive 11"(w116) -> ()
        n273 = local write "SWDDrive 12"(w116) -> ()
        n274 = local write "Let 2"(w116) -> ()
        n275 = local write "Nolet2 2"(w116) -> ()
        n276 = local write "Nolet1 2"(w116) -> ()
        n277 = local write "Stroke2 2"(w116) -> ()
        n278 = local write "Stroke1 2"(w116) -> ()
        n279 = local write "Unforced Error2 2"(w116) -> ()
        n280 = local write "Forced Error2 2"(w116) -> ()
        n281 = local write "Unforced Error1 2"(w116) -> ()
        n282 = local write "Forced Error1 2"(w116) -> ()
        n283 = local write "Unexpected Winner2 2"(w116) -> ()
        n284 = local write "Unexpected Winner1 2"(w116) -> ()
        n285 = local write "Expected Winner2 2"(w116) -> ()
        n286 = local write "Expected Winner1 2"(w116) -> ()
        n287 = local write "Boast"(w116) -> ()
        n288 = local write "Boast 2"(w116) -> ()
        n289 = local write "Boast 3"(w116) -> ()
        n290 = local write "Boast 4"(w116) -> ()
        n291 = local write "Boast 5"(w116) -> ()
        n292 = local write "Boast 6"(w116) -> ()
        n293 = local write "Boast 7"(w116) -> ()
        n294 = local write "Boast 8"(w116) -> ()
        n295 = local write "Boast 9"(w116) -> ()
        n296 = local write "Boast 10"(w116) -> ()
        n297 = local write "Boast 11"(w116) -> ()
        n298 = local write "Boast 12"(w116) -> ()
        n299 = local write "4 4"(w116) -> ()
        n300 = local write "4 3"(w116) -> ()
        n301 = local write "4 2"(w116) -> ()
        n302 = local write "4 1"(w116) -> ()
        n303 = local write "3 4"(w116) -> ()
        n304 = local write "3 3"(w116) -> ()
        n305 = local write "3 2"(w116) -> ()
        n306 = local write "3 1"(w116) -> ()
        n307 = local write "2 4"(w116) -> ()
        n308 = local write "2 3"(w116) -> ()
        n309 = local write "2 2"(w116) -> ()
        n310 = local write "2 1"(w116) -> ()
        n311 = local write "1 4"(w116) -> ()
        n312 = local write "1 3"(w116) -> ()
        n313 = local write "1 2"(w116) -> ()
        n314 = local write "1 1"(w116) -> ()
        n315 = local write "5 4"(w116) -> ()
        n316 = local write "5 3"(w116) -> ()
        n317 = local write "5 2"(w116) -> ()
        n318 = local write "5 1"(w116) -> ()
        n319 = local write "6 4"(w116) -> ()
        n320 = local write "6 3"(w116) -> ()
        n321 = local write "6 2"(w116) -> ()
        n322 = local write "6 1"(w116) -> ()
        n323 = local write "S6"(w116) -> ()
        n324 = local write "S5"(w116) -> ()
        n325 = local write "S4"(w116) -> ()
        n326 = local write "S1"(w116) -> ()
        n327 = local write "S2"(w116) -> ()
        n328 = local write "S3"(w116) -> ()
        n329 = local write "Let"(w116) -> ()
        n330 = local write "Unexpected Winner2"(w116) -> ()
        n331 = local write "Unexpected Winner1"(w116) -> ()
        n332 = local write "Expected Winner2"(w116) -> ()
        n333 = local write "Expected Winner1"(w116) -> ()
        n334 = local write "Forced Error2"(w116) -> ()
        n335 = local write "Forced Error1"(w116) -> ()
        n336 = local write "Service2"(w116) -> ()
        n337 = local write "Service1"(w116) -> ()
        n338 = local write "Nolet2"(w116) -> ()
        n339 = local write "Nolet1"(w116) -> ()
        n340 = local write "Stroke2"(w116) -> ()
        n341 = local write "Stroke1"(w116) -> ()
        n342 = local write "Unforced Error2"(w116) -> ()
        n343 = local write "Unforced Error1"(w116) -> ()
        n344 = local write "Button 5"(w116) -> ()
        n345 = local write "Button 4"(w116) -> ()
        n346 = local write "Button 3"(w116) -> ()
        n347 = local write "Button 2"(w116) -> ()
        n348 = local write "Button 1"(w116) -> ()
        "Score change" <- bool[] [FALSE, FALSE] ("Score change")
        "Player1/Player2" <- bool[] [TRUE, FALSE] ("Score change")
      }
      frame #3 {
        w161 = T5 4 items=["Grayscale (U8)", "Grayscale (I16)", "Grayscale (SGL)", "Complex (CSG)", "RGB (U32)", "HSL (U32)", "RGB (U64)"] ("Image Type")
        n349 = Path to Array of Strings(0:w159) -> (2:w172:string[])  [unwired: 1 out]
        n350 = call "IMAQ AVI Open"("AVI Path"=w159) -> ("error out"=w163:errorcluster, "Avi Refnum"=w162:T6)  [unwired: 9 in]
        n351 = Delete From Array(array=w172) -> (array with subset deleted=w173:string[])  [unwired: 2 in, 1 out]
        n352 = call "IMAQ AVI Get Info"("error in (no error)"=w163, "Avi Refnum"=w162) -> ("error out"=w165:errorcluster, "Number of Frames"=w168:u32, "Avi Refnum (duplicate)"=w158:T6, "Frame Data"=w164:T7)  [unwired: 5 in, 1 out]
        "Number of Frames" <- w168
        n353 = Array of Strings to Path(0:w173) -> (2:w174:path)  [unwired: 1 in]
        n354 = call-poly <vilib>:"Read From Spreadsheet File.vi"("file path (dialog if empty)"=w176) -> ("all rows"=w179:i64[][])  [unwired: 6 in, 4 out]
        n355 = Decrement(x=w168) -> (x-1=w171:u32)
        n356 = local write "Video to write"(w174) -> ()
        n357 = Subtract(x=w171, y=200.0) -> (x-y=w169:dbl)
        n358 = Unbundle By Name(w164) -> ("framesPerSecond"=→"framesPerSecond":u32)
        n359 = property on="Progress..." class="Slide (strict)"(error in=w165, "Scale.Maximum"=w171) -> (error out=w166:errorcluster)  [unwired: 1 in, 1 out]
        n360 = Delete From Array(array=w179, length=4, index (row)=0) -> (array with subset deleted=w175:i64[][])  [unwired: 1 in, 1 out]
        n361 = for {
          N: w169 -> [_]
          tunnel: [w183] -> w155 mode=indexing
          i -> [w183]
        }
        "ful video frames" <- w155
        n362 = Index Array(array=w175, index (col)=0 ("disabled index (col)")) -> (element=w181:i64[])  [unwired: 1 in]
        n363 = Array Max & Min(array=w181) -> (max value=w180:i64)  [unwired: 3 out]
        n364 = call "IMAQ Create"("Image Name"="Video", "Image Type"=w161, "error in (no error)"=w166) -> ("New Image"=w157:T2, "error out"=w156:errorcluster)  [unwired: 2 in]
        n365 = local write "Progress..."(w180) -> ()
      }
    }
    n366 = while {
      tunnel: w10 -> [w355]
      tunnel: w9 -> [w354]
      tunnel: w1 -> [w353]
      shift-right: [w347] -> _
      shift-left: w8 -> [w346]
      tunnel: [w330] -> w4
      stop <- w331 continue-if-true
      # "This loop is the video play loop"
      # "1000/playback speed    / frames per sec"
      n367 = while {
        stop <- w371 continue-if-true
        n368 = local read "START"() -> (w370:bool)
        n369 = And(x=w370, y="Pause") -> (x .and. y?=w371:bool)
      }
      n370 = Index Array(array=w346, index="Progress...") -> (element=w333:i64)
      n371 = Array Max & Min(array=w346) -> (max value=w351:i64, max index (indices)=w352:i32)  [unwired: 2 out]
      n372 = while {
        stop <- w360 stop-if-true
        n373 = local read "START"() -> (w357:bool)
        n374 = Not(x=w357) -> (.not. x?=w356:bool)
        n375 = Compound Arithmetic op=OR(w356, "Play", "Load video", "stop") -> (w360:bool)
        n376 = case shown="True" "stop" {
          frame False {
          }
          frame True {
            w362 = FALSE ("Play")
            n377 = local write "stop"(w362) -> ()
            n378 = local write "Play"(w362) -> ()
          }
        }
      }
      n379 = property on="Progress..." class="Slide (strict)"("Scale.Maximum"=w352) -> ()  [unwired: 2 in, 2 out]
      n380 = Increment(x=w333) -> (x+1=w334:i64)
      n381 = Greater Or Equal?(x=w334, y=w351) -> (x >= y?=w337:bool)
      n382 = Select(t=w351, s=w337, f=w333) -> (s? t:f=w348:i64)
      "Video Frame" <- w348
      n383 = call "IMAQ AVI Read Frame"("error in (no error)"=w353, "Frame Number"=w348, "Image"=w354, "Avi Refnum"=w355) -> ("Image Out"=→"Video":T2, "Avi Refnum (duplicate)"=w330:T6)  [unwired: 4 in, 2 out]
      n384 = Search 1D Array(1D array=w346, element=w348) -> ()  [unwired: 1 in, 1 out]
      n385 = Or(x="fast forward", y="fast rewind") -> (x .or. y?=w328:bool)
      n386 = Increment(x="Progress...") -> (x+1=w329:u32)
      n387 = Select(t=1.0, s=w328, f="playback speed") -> (s? t:f=w340:dbl)
      n388 = Increment(x=w329) -> (x+1=w332:u32)
      n389 = local read "framesPerSecond"() -> (w345:u32)
      n390 = Select(t=w332, s="fast forward", f=w329) -> (s? t:f=w324:u32)
      n391 = Subtract(x="Progress...", y=2) -> (x-y=w325:u32)
      n392 = Divide(x=1000.0, y=w340) -> (x/y=w344:dbl)
      n393 = Divide(x=w344, y=w345) -> (x/y=w342:dbl)
      n394 = Select(t=w325, s="fast rewind", f=w324) -> (s? t:f=w323:u32)
      n395 = Round Toward -Infinity(1:w342) -> (0:w341:dbl)
      "playback speed" <- w341
      n396 = Wait (ms)(milliseconds to wait=w341) -> ()  [unwired: 1 out]
      n397 = local read "Load video"() -> (w335:bool)
      n398 = Select(t="Progress...", s=w337, f=w323) -> (s? t:f=w336:u32)
      n399 = case shown="True" w335 {
        tunnel: w346 -> [w363 _]
        tunnel: w336 -> [w364 _]
        tunnel: [w364 w365] -> w350
        tunnel: [w363 w368] -> w347
        frame False {
        }
        frame True {
          n400 = local read "frames 2 play"() -> (w368:i64[])
          n401 = Array Max & Min(array=w368) -> (max index (indices)=w367:i32)  [unwired: 3 out]
          n402 = property on="Progress..." class="Slide (strict)"("Scale.Maximum"=w367) -> ()  [unwired: 2 in, 2 out]
          n403 = local write "Load video"(FALSE ("Play")) -> ()
          n404 = local read "Progress..."() -> (w365:u32)
        }
      }
      n405 = local write "Progress..."(w350) -> ()
      n406 = local read "START"() -> (w331:bool)
    }
    n407 = while {
      shift-right: [w372] -> _
      shift-left: T1."Display" ("Main tab") -> [w373]
      tunnel: w10 -> [w386]
      shift-right: [w376] -> _
      shift-left: w11 -> [w389]
      tunnel: w8 -> [_]
      tunnel: w1 -> [_]
      tunnel: [w374] -> w7
      stop <- w375 continue-if-true
      w379 = T1."Coding" ("Main tab")
      # "Moving to display tab"
      n408 = case shown="\"Edit coding\"" w373 {
        tunnel: w389 -> [w576 w1482 w1740 w2105 w2142 w2277]
        tunnel: [w420 w1482 w1740 w2105 w2142 w2259] -> w376
        tunnel: [T1."Edit video" ("Main tab") w1494 T1."Display" ("Main tab") T1."Edit coding" ("Main tab") w2143 T1."Edit video" ("Main tab")] -> w381
        tunnel: w386 -> [w574 _ _ _ _ _]
        tunnel: [w416 w1487 w1754 w2103 w2140 w2265] -> w374
        frame "Coding", Default {
          n409 = local read "Drop"() -> (w572:bool)
          n410 = local read "Drop 2"() -> (w571:bool)
          n411 = local read "Drop 3"() -> (w570:bool)
          n412 = local read "Drop 4"() -> (w569:bool)
          n413 = local read "Drop 5"() -> (w568:bool)
          n414 = local read "Drop 6"() -> (w567:bool)
          n415 = local read "Drop 7"() -> (w566:bool)
          n416 = local read "Drop 8"() -> (w565:bool)
          n417 = local read "Drop 9"() -> (w564:bool)
          n418 = local read "Drop 10"() -> (w563:bool)
          n419 = local read "Drop 11"() -> (w562:bool)
          n420 = local read "Drop 12"() -> (w561:bool)
          n421 = local read "Chop"() -> (w560:bool)
          n422 = local read "Chop 2"() -> (w559:bool)
          n423 = local read "Chop 3"() -> (w558:bool)
          n424 = local read "Chop 4"() -> (w557:bool)
          n425 = local read "Chop 5"() -> (w556:bool)
          n426 = local read "Chop 6"() -> (w555:bool)
          n427 = local read "Chop 7"() -> (w554:bool)
          n428 = local read "Chop 8"() -> (w553:bool)
          n429 = local read "Chop 9"() -> (w552:bool)
          n430 = local read "Chop 10"() -> (w551:bool)
          n431 = local read "Chop 11"() -> (w550:bool)
          n432 = local read "Chop 12"() -> (w549:bool)
          n433 = local read "Let"() -> (w548:bool)
          n434 = local read "Unexpected Winner2"() -> (w539:bool)
          n435 = local read "Unexpected Winner1"() -> (w538:bool)
          n436 = local read "Expected Winner2"() -> (w537:bool)
          n437 = local read "Expected Winner1"() -> (w536:bool)
          n438 = local read "Forced Error2"() -> (w542:bool)
          n439 = local read "Forced Error1"() -> (w540:bool)
          n440 = local read "Nolet2"() -> (w547:bool)
          n441 = local read "Nolet1"() -> (w546:bool)
          n442 = local read "Stroke2"() -> (w545:bool)
          n443 = local read "Stroke1"() -> (w544:bool)
          n444 = local read "Unforced Error2"() -> (w543:bool)
          n445 = local read "Unforced Error1"() -> (w541:bool)
          n446 = Build Array(w572, w571, w570, w569, w568, w567, w566, w565, w564, w563, w562, w561, w560, w559, w558, w557, w556, w555, w554, w553, w552, w551, w550, w549, w548, w547, w546, w545, w544, w543, w542, w541, w540, w539, w538, w537, w536) -> (w426:bool[])
          n447 = local read "lob 13"() -> (w535:bool)
          n448 = local read "lob 2"() -> (w534:bool)
          n449 = local read "lob 3"() -> (w533:bool)
          n450 = local read "lob 4"() -> (w532:bool)
          n451 = local read "lob 5"() -> (w531:bool)
          n452 = local read "lob 6"() -> (w530:bool)
          n453 = local read "lob 7"() -> (w529:bool)
          n454 = local read "lob 8"() -> (w528:bool)
          n455 = local read "lob 9"() -> (w527:bool)
          n456 = local read "lob 10"() -> (w526:bool)
          n457 = local read "lob 11"() -> (w525:bool)
          n458 = local read "lob 12"() -> (w524:bool)
          n459 = local read "Smash"() -> (w523:bool)
          n460 = local read "Smash 2"() -> (w522:bool)
          n461 = local read "Smash 3"() -> (w521:bool)
          n462 = local read "Smash 4"() -> (w520:bool)
          n463 = local read "Smash 5"() -> (w519:bool)
          n464 = local read "Smash 6"() -> (w518:bool)
          n465 = local read "Smash 7"() -> (w517:bool)
          n466 = local read "Smash 8"() -> (w516:bool)
          n467 = local read "Smash 9"() -> (w515:bool)
          n468 = local read "Smash 10"() -> (w514:bool)
          n469 = local read "Smash 11"() -> (w513:bool)
          n470 = local read "Smash 12"() -> (w512:bool)
          n471 = local read "Boast"() -> (w511:bool)
          n472 = local read "Boast 2"() -> (w510:bool)
          n473 = local read "Boast 3"() -> (w509:bool)
          n474 = local read "Boast 4"() -> (w508:bool)
          n475 = local read "Boast 5"() -> (w507:bool)
          n476 = local read "Boast 6"() -> (w506:bool)
          n477 = local read "Boast 7"() -> (w505:bool)
          n478 = local read "Boast 8"() -> (w504:bool)
          n479 = local read "Boast 9"() -> (w503:bool)
          n480 = local read "Boast 10"() -> (w502:bool)
          n481 = local read "Boast 11"() -> (w501:bool)
          n482 = local read "Boast 12"() -> (w500:bool)
          n483 = Build Array(w535, w534, w533, w532, w531, w530, w529, w528, w527, w526, w525, w524, w523, w522, w521, w520, w519, w518, w517, w516, w515, w514, w513, w512, w511, w510, w509, w508, w507, w506, w505, w504, w503, w502, w501, w500) -> (w425:bool[])
          n484 = local read "Player2"() -> (w417:bool)
          n485 = local read "Player1"() -> (w418:bool)
          n486 = local read "Pause"() -> (w419:bool)
          n487 = local read "ADrive"() -> (w499:bool)
          n488 = local read "ADrive 2"() -> (w498:bool)
          n489 = local read "ADrive 3"() -> (w497:bool)
          n490 = local read "ADrive 4"() -> (w496:bool)
          n491 = local read "ADrive 5"() -> (w495:bool)
          n492 = local read "ADrive 6"() -> (w494:bool)
          n493 = local read "ADrive 7"() -> (w493:bool)
          n494 = local read "ADrive 8"() -> (w492:bool)
          n495 = local read "ADrive 9"() -> (w491:bool)
          n496 = local read "ADrive 10"() -> (w490:bool)
          n497 = local read "ADrive 11"() -> (w489:bool)
          n498 = local read "ADrive 12"() -> (w488:bool)
          n499 = local read "SWADrive"() -> (w487:bool)
          n500 = local read "SWADrive 2"() -> (w486:bool)
          n501 = local read "SWADrive 3"() -> (w485:bool)
          n502 = local read "SWADrive 4"() -> (w484:bool)
          n503 = local read "SWADrive 5"() -> (w483:bool)
          n504 = local read "SWADrive 6"() -> (w482:bool)
          n505 = local read "SWADrive 7"() -> (w481:bool)
          n506 = local read "SWADrive 8"() -> (w480:bool)
          n507 = local read "SWADrive 9"() -> (w479:bool)
          n508 = local read "SWADrive 10"() -> (w478:bool)
          n509 = local read "SWADrive 11"() -> (w477:bool)
          n510 = local read "SWADrive 12"() -> (w476:bool)
          n511 = local read "S6"() -> (w473:bool)
          n512 = local read "S5"() -> (w472:bool)
          n513 = local read "S4"() -> (w471:bool)
          n514 = local read "S1"() -> (w470:bool)
          n515 = local read "S2"() -> (w469:bool)
          n516 = local read "S3"() -> (w468:bool)
          n517 = local read "Service2"() -> (w475:bool)
          n518 = local read "Service1"() -> (w474:bool)
          n519 = Build Array(w499, w498, w497, w496, w495, w494, w493, w492, w491, w490, w489, w488, w487, w486, w485, w484, w483, w482, w481, w480, w479, w478, w477, w476, w475, w474, w473, w472, w471, w470, w469, w468, w419, w418, w417) -> (w424:bool[])
          n520 = local read "DDrive"() -> (w467:bool)
          n521 = local read "DDrive 2"() -> (w466:bool)
          n522 = local read "DDrive 3"() -> (w465:bool)
          n523 = local read "DDrive 4"() -> (w464:bool)
          n524 = local read "DDrive 5"() -> (w463:bool)
          n525 = local read "DDrive 6"() -> (w462:bool)
          n526 = local read "DDrive 7"() -> (w461:bool)
          n527 = local read "DDrive 8"() -> (w460:bool)
          n528 = local read "DDrive 9"() -> (w459:bool)
          n529 = local read "DDrive 10"() -> (w458:bool)
          n530 = local read "DDrive 11"() -> (w457:bool)
          n531 = local read "DDrive 12"() -> (w456:bool)
          n532 = local read "SWDDrive"() -> (w455:bool)
          n533 = local read "SWDDrive 2"() -> (w454:bool)
          n534 = local read "SWDDrive 3"() -> (w453:bool)
          n535 = local read "SWDDrive 4"() -> (w452:bool)
          n536 = local read "SWDDrive 5"() -> (w451:bool)
          n537 = local read "SWDDrive 6"() -> (w450:bool)
          n538 = local read "SWDDrive 7"() -> (w449:bool)
          n539 = local read "SWDDrive 8"() -> (w448:bool)
          n540 = local read "SWDDrive 9"() -> (w447:bool)
          n541 = local read "SWDDrive 10"() -> (w446:bool)
          n542 = local read "SWDDrive 11"() -> (w445:bool)
          n543 = local read "SWDDrive 12"() -> (w444:bool)
          n544 = local read "Button 5"() -> (w415:bool)
          n545 = local read "Button 4"() -> (w414:bool)
          n546 = local read "Button 3"() -> (w413:bool)
          n547 = local read "Button 2"() -> (w412:bool)
          n548 = local read "Button 1"() -> (w411:bool)
          n549 = Build Array(w467, w466, w465, w464, w463, w462, w461, w460, w459, w458, w457, w456, w455, w454, w453, w452, w451, w450, w449, w448, w447, w446, w445, w444) -> (w422:bool[])
          n550 = local read "4 4"() -> (w436:bool)
          n551 = local read "4 3"() -> (w437:bool)
          n552 = local read "4 2"() -> (w438:bool)
          n553 = local read "4 1"() -> (w439:bool)
          n554 = local read "3 4"() -> (w440:bool)
          n555 = local read "3 3"() -> (w441:bool)
          n556 = local read "3 2"() -> (w442:bool)
          n557 = local read "3 1"() -> (w443:bool)
          n558 = local read "2 4"() -> (w435:bool)
          n559 = local read "2 3"() -> (w434:bool)
          n560 = local read "2 2"() -> (w433:bool)
          n561 = local read "2 1"() -> (w432:bool)
          n562 = local read "1 4"() -> (w431:bool)
          n563 = local read "1 3"() -> (w430:bool)
          n564 = local read "1 2"() -> (w429:bool)
          n565 = local read "1 1"() -> (w428:bool)
          n566 = local read "5 4"() -> (w409:bool)
          n567 = local read "5 3"() -> (w408:bool)
          n568 = local read "5 2"() -> (w407:bool)
          n569 = local read "5 1"() -> (w406:bool)
          n570 = local read "6 4"() -> (w405:bool)
          n571 = local read "6 3"() -> (w404:bool)
          n572 = local read "6 2"() -> (w403:bool)
          n573 = local read "6 1"() -> (w402:bool)
          n574 = local read "Undo"() -> (w401:bool)
          n575 = Build Array(w415, w414, w413, w412, w411, w401) -> (w410:bool[])
          n576 = Build Array(w436, w437, w438, w439, w440, w441, w442, w443, w435, w434, w433, w432, w431, w430, w429, w428, w409, w408, w407, w406, w405, w404, w403, w402) -> (w423:bool[])
          n577 = local read "Video Frame"() -> (w573:u32)
          n578 = Build Array(w410, w422, w423, w424, w425, w426) -> (w427:bool[][])
          n579 = Or Array Elements(Boolean array=w427) -> (logical OR=w421:bool)
          n580 = case shown="True" w421 {
            tunnel: w573 -> [_ w739]
            tunnel: w576 -> [w580 w740]
            tunnel: [w580 w603] -> w420
            tunnel: w574 -> [_ w736]
            tunnel: [w577 w632] -> w416
            frame False {
              n581 = local read "Data file"() -> (w578:path)
              n582 = Open/Create/Replace File(file path (use dialog)=w578, operation (0:open)=T3."open") -> (refnum out=w577:refnum<file>)  [unwired: 4 in, 2 out]
            }
            frame True {
              w597 = 0 ("index")
              w607 = "\t"
              w643 = "\r"
              # "extra code buttons\n\nundo button / error button\n\nlink all (extra buttons) to linkshots logic"
              n583 = stacked-sequence {
                tunnel: w740 -> [w764 _ _ _ _ _ _ _ _ _ _ _ _ _ w1430 _]
                tunnel: [w764 _ _ _ _ _ _ _ _ _ _ _ _ _ _ _] -> w601
                tunnel: w739 -> [w770 _ _ _ _ _ _ _ _ _ _ _ _ _ _ _]
                tunnel: [w770 _ _ _ _ _ _ _ _ _ _ _ _ _ _ _] -> w605
                tunnel: w736 -> [w769 _ _ _ _ _ _ _ _ _ _ _ _ _ _ _]
                tunnel: [w766 _ _ _ _ _ _ _ _ _ _ _ _ _ _ _] -> w735
                tunnel: [_ _ "before 2" _ _ _ _ _ _ _ _ _ _ _ _ _] -> w734
                tunnel: [_ _ "after 2" _ _ _ _ _ _ _ _ _ _ _ _ _] -> w733
                tunnel: [_ _ w851 _ _ _ _ _ _ _ _ _ _ _ _ _] -> w732
                tunnel: [_ _ w850 _ _ _ _ _ _ _ _ _ _ _ _ _] -> w731
                tunnel: [_ _ w849 _ _ _ _ _ _ _ _ _ _ _ _ _] -> w730
                tunnel: [_ _ w848 _ _ _ _ _ _ _ _ _ _ _ _ _] -> w729
                tunnel: [_ _ w847 _ _ _ _ _ _ _ _ _ _ _ _ _] -> w728
                tunnel: [_ _ w846 _ _ _ _ _ _ _ _ _ _ _ _ _] -> w727
                tunnel: [_ _ w845 _ _ _ _ _ _ _ _ _ _ _ _ _] -> w726
                tunnel: [_ _ w844 _ _ _ _ _ _ _ _ _ _ _ _ _] -> w725
                tunnel: [_ _ w843 _ _ _ _ _ _ _ _ _ _ _ _ _] -> w724
                tunnel: [_ _ w842 _ _ _ _ _ _ _ _ _ _ _ _ _] -> w723
                tunnel: [_ _ w841 _ _ _ _ _ _ _ _ _ _ _ _ _] -> w722
                tunnel: [_ _ w840 _ _ _ _ _ _ _ _ _ _ _ _ _] -> w721
                tunnel: [_ _ w839 _ _ _ _ _ _ _ _ _ _ _ _ _] -> w720
                tunnel: [_ _ w838 _ _ _ _ _ _ _ _ _ _ _ _ _] -> w719
                tunnel: [_ _ w837 _ _ _ _ _ _ _ _ _ _ _ _ _] -> w718
                tunnel: [_ _ w836 _ _ _ _ _ _ _ _ _ _ _ _ _] -> w717
                tunnel: [_ _ w835 _ _ _ _ _ _ _ _ _ _ _ _ _] -> w716
                tunnel: [_ _ w834 _ _ _ _ _ _ _ _ _ _ _ _ _] -> w715
                tunnel: [_ _ w833 _ _ _ _ _ _ _ _ _ _ _ _ _] -> w714
                tunnel: [_ _ w832 _ _ _ _ _ _ _ _ _ _ _ _ _] -> w713
                tunnel: [_ _ w831 _ _ _ _ _ _ _ _ _ _ _ _ _] -> w712
                tunnel: [_ _ w830 _ _ _ _ _ _ _ _ _ _ _ _ _] -> w711
                tunnel: [_ _ w829 _ _ _ _ _ _ _ _ _ _ _ _ _] -> w710
                tunnel: [_ _ w828 _ _ _ _ _ _ _ _ _ _ _ _ _] -> w709
                tunnel: [_ _ _ w893 _ _ _ _ _ _ _ _ _ _ _ _] -> w708
                tunnel: [_ _ _ w892 _ _ _ _ _ _ _ _ _ _ _ _] -> w707
                tunnel: [_ _ _ w891 _ _ _ _ _ _ _ _ _ _ _ _] -> w706
                tunnel: [_ _ _ w890 _ _ _ _ _ _ _ _ _ _ _ _] -> w705
                tunnel: [_ _ _ _ w948 _ _ _ _ _ _ _ _ _ _ _] -> w704
                tunnel: [_ _ _ _ w947 _ _ _ _ _ _ _ _ _ _ _] -> w703
                tunnel: [_ _ _ _ w946 _ _ _ _ _ _ _ _ _ _ _] -> w702
                tunnel: [_ _ _ _ _ w990 _ _ _ _ _ _ _ _ _ _] -> w701
                tunnel: [_ _ _ _ _ w989 _ _ _ _ _ _ _ _ _ _] -> w700
                tunnel: [_ _ _ _ _ w988 _ _ _ _ _ _ _ _ _ _] -> w699
                tunnel: [_ _ _ _ _ _ w1018 _ _ _ _ _ _ _ _ _] -> w698
                tunnel: [_ _ _ _ _ _ _ w1076 _ _ _ _ _ _ _ _] -> w697
                tunnel: [_ _ _ _ _ _ _ _ w1134 _ _ _ _ _ _ _] -> w696
                tunnel: [_ _ _ _ _ _ _ _ _ w1186 _ _ _ _ _ _] -> w695
                tunnel: [_ _ _ _ _ _ _ _ _ _ w1250 _ _ _ _ _] -> w694
                tunnel: [_ _ _ _ _ _ _ _ _ _ _ w1290 _ _ _ _] -> w693
                tunnel: [_ _ _ _ _ _ _ _ _ _ _ _ w1330 _ _ _] -> w692
                tunnel: [_ _ _ _ _ _ _ _ _ _ _ _ _ _ w1393 _] -> w691
                tunnel: [_ _ _ _ _ _ _ _ _ _ _ _ _ _ w1394 _] -> w690
                tunnel: [_ _ _ _ _ _ _ _ _ _ _ _ _ _ w1395 _] -> w689
                tunnel: [_ _ _ _ _ _ _ _ _ _ _ _ _ _ w1400 _] -> w688
                tunnel: [_ _ _ _ _ _ _ _ _ _ _ _ _ _ w1401 _] -> w687
                tunnel: [_ _ _ _ _ _ _ _ _ _ _ _ _ _ w1402 _] -> w686
                tunnel: [_ _ _ _ _ _ _ _ _ _ _ _ _ _ w1403 _] -> w685
                tunnel: [_ _ _ _ _ _ _ _ _ _ _ _ _ _ w1404 _] -> w684
                tunnel: [_ _ _ _ _ _ _ _ _ _ _ _ _ _ w1405 _] -> w683
                tunnel: [_ _ _ _ _ _ _ _ _ _ _ _ _ _ w1406 _] -> w682
                tunnel: [_ _ _ _ _ _ _ _ _ _ _ _ _ _ w1407 _] -> w681
                tunnel: [_ _ _ _ _ _ _ _ _ _ _ _ _ _ w1408 _] -> w680
                tunnel: [_ _ _ _ _ _ _ _ _ _ _ _ _ _ w1408 _] -> w679
                tunnel: [_ _ _ _ _ _ _ _ _ _ _ _ _ _ w1396 _] -> w678
                tunnel: [_ _ _ _ _ _ _ _ _ _ _ _ _ _ w1397 _] -> w677
                tunnel: [_ _ _ _ _ _ _ _ _ _ _ _ _ _ w1398 _] -> w676
                tunnel: [_ _ _ _ _ _ _ _ _ _ _ _ _ _ w1399 _] -> w675
                tunnel: [_ _ _ _ _ _ _ _ _ _ _ _ _ _ _ w1449] -> w646
                tunnel: [_ _ _ _ _ _ _ _ _ _ _ _ _ w1379 _ _] -> w631
                tunnel: [_ _ _ _ _ _ _ _ _ _ _ _ _ w1378 _ _] -> w630
                tunnel: [_ _ _ _ _ _ _ _ _ _ _ _ _ w1377 _ _] -> w629
                tunnel: [_ _ _ _ _ _ _ _ _ _ _ _ _ w1376 _ _] -> w628
                tunnel: [_ _ _ _ _ _ _ _ _ _ _ _ _ w1375 _ _] -> w627
                tunnel: [_ _ w815 _ _ _ _ _ _ _ _ _ _ _ _ _] -> w619
                tunnel: [_ _ _ _ _ _ _ _ _ _ _ _ _ w1374 _ _] -> w618
                tunnel: [_ _ _ _ _ _ _ _ _ _ _ _ _ w1373 _ _] -> w617
                tunnel: [_ _ _ _ _ _ _ _ _ _ _ _ _ w1372 _ _] -> w616
                tunnel: [_ _ _ _ _ _ _ _ _ _ _ _ _ w1371 _ _] -> w615
                tunnel: [_ _ _ _ _ _ _ _ _ _ _ _ _ w1370 _ _] -> w614
                tunnel: [_ _ w819 _ _ _ _ _ _ _ _ _ _ _ _ _] -> w613
                tunnel: [_ _ w818 _ _ _ _ _ _ _ _ _ _ _ _ _] -> w612
                tunnel: [_ _ w817 _ _ _ _ _ _ _ _ _ _ _ _ _] -> w611
                tunnel: [_ _ w816 _ _ _ _ _ _ _ _ _ _ _ _ _] -> w610
                frame #0 {
                  n584 = local read "Pause"() -> (w765:bool)
                  n585 = And(x=w765, y="Pause lag on") -> (x .and. y?=w768:bool)
                  n586 = case shown="False" w765 {
                    frame False {
                      n587 = Tick Count (ms)() -> (millisecond timer value=w771:u32)
                      n588 = while {
                        tunnel: w771 -> [w783]
                        i -> [w774]
                        stop <- w781 stop-if-true
                        w777 = u32 25 ("milliseconds to wait")
                        n589 = Tick Count (ms)() -> (millisecond timer value=w784:u32)
                        n590 = Subtract(x=w784, y=w783) -> (x-y=w782:u32)
                        n591 = Multiply(x="Code lag(s)", y=1000) -> (x*y=w778:dbl)
                        n592 = Greater Or Equal?(x=w782, y=w778) -> (x >= y?=w781:bool)
                        n593 = Divide(x=w778, y=w777) -> (x/y=w776:dbl)
                        n594 = Divide(x=300.0, y=w776) -> (x/y=w773:dbl)
                        n595 = Multiply(x=w774, y=w773) -> (x*y=→"task":dbl)
                        n596 = Wait (ms)(milliseconds to wait=w777) -> ()  [unwired: 1 out]
                      }
                    }
                    frame True {
                    }
                  }
                  n597 = case shown="True" w768 {
                    tunnel: w770 -> [_ w788]
                    tunnel: w769 -> [_ w790]
                    tunnel: ["pauselag" ("Image Name") w786] -> w766
                    frame False {
                    }
                    frame True {
                      w791 = T5 4 items=["Grayscale (U8)", "Grayscale (I16)", "Grayscale (SGL)", "Complex (CSG)", "RGB (U32)", "HSL (U32)", "RGB (U64)"] ("Image Type")
                      n598 = local read "framesPerSecond"() -> (w797:u32)
                      n599 = local read "Number of Frames"() -> (w787:u32)
                      n600 = Increment(x=w788) -> (x+1=w789:u32)
                      n601 = Multiply(x="Pause lag(s)", y=w797) -> (x*y=w795:dbl)
                      n602 = call "IMAQ Create"("Image Name"="pauselag", "Image Type"=w791) -> ("New Image"=w786:T2, "error out"=w792:errorcluster)  [unwired: 3 in]
                      n603 = Round Toward +Infinity(x=w795) -> (ceil(x): smallest int >= x=w794:dbl)
                      n604 = for {
                        N: w794 -> [_]
                        tunnel: w789 -> [w804]
                        tunnel: w792 -> [w807]
                        tunnel: w786 -> [w806]
                        tunnel: w790 -> [w803]
                        tunnel: w787 -> [w801]
                        i -> [w805]
                        n605 = Add(x=w805, y=w804) -> (x+y=w800:u32)
                        n606 = local read "playback speed"() -> (w798:dbl)
                        n607 = Less Or Equal?(x=w801, y=w800) -> (x <= y?=w802:bool)
                        n608 = Select(t=w801, s=w802, f=w800) -> (s? t:f=w799:u32)
                        n609 = call "IMAQ AVI Read Frame"("error in (no error)"=w807, "Frame Number"=w799, "Image"=w806, "Avi Refnum"=w803) -> ("Image Out"=w808:T2)  [unwired: 4 in, 3 out]
                        n610 = local write "Video"(w808) -> ()
                        n611 = Wait (ms)(milliseconds to wait=w798) -> ()  [unwired: 1 out]
                      }
                    }
                  }
                }
                frame #1 {
                  w809 = i16 0 ("Service")
                  n612 = while {
                    stop <- w810 continue-if-true
                    n613 = local read "START"() -> (w811:bool)
                    n614 = local read "Pause"() -> (w812:bool)
                    n615 = And(x=w811, y=w812) -> (x .and. y?=w810:bool)
                  }
                  n616 = local write "Service"(w809) -> ()
                  n617 = local write "Cross"(w809) -> ()
                  n618 = local write "Straight"(w809) -> ()
                  n619 = local write "position"(w809) -> ()
                  n620 = local write "Player 1/2"(w809) -> ()
                  n621 = local write "Extra"(w809) -> ()
                }
                frame #2 {
                  n622 = local read "Service1"() -> (w859:bool)
                  n623 = local read "Service2"() -> (w861:bool)
                  n624 = Compound Arithmetic op=OR(w859, "Player1", w861, "Player2") -> (w858:bool)
                  n625 = Or(x="Player1", y="Player2") -> (x .or. y?=w864:bool)
                  n626 = case shown="True" w858 {
                    tunnel: w859 -> [_ w887]
                    tunnel: w861 -> [_ w886]
                    tunnel: "Player1" -> [_ w885]
                    tunnel: "Player2" -> [_ w884]
                    frame False {
                    }
                    frame True {
                      n627 = Or(x=w887, y=w885) -> (x .or. y?=w889:bool)
                      n628 = Or(x=w886, y=w884) -> (x .or. y?=w888:bool)
                      n629 = Build Array(w889, w888) -> (w883:bool[])
                      n630 = local write "Player1/Player2"(w883) -> ()
                    }
                  }
                  n631 = Boolean To (0,1)(Boolean=w864) -> (0, 1=→"Player 1/2":i16)
                  n632 = Boolean To (0,1)(Boolean="1 1") -> (0, 1=w851:i16)
                  n633 = Boolean To (0,1)(Boolean="1 2") -> (0, 1=w850:i16)
                  n634 = Boolean To (0,1)(Boolean="1 3") -> (0, 1=w849:i16)
                  n635 = Boolean To (0,1)(Boolean="1 4") -> (0, 1=w848:i16)
                  n636 = Boolean To (0,1)(Boolean="2 1") -> (0, 1=w847:i16)
                  n637 = Boolean To (0,1)(Boolean="2 2") -> (0, 1=w846:i16)
                  n638 = Boolean To (0,1)(Boolean="2 3") -> (0, 1=w845:i16)
                  n639 = Boolean To (0,1)(Boolean="2 4") -> (0, 1=w844:i16)
                  n640 = Boolean To (0,1)(Boolean="3 1") -> (0, 1=w843:i16)
                  n641 = Boolean To (0,1)(Boolean="3 2") -> (0, 1=w842:i16)
                  n642 = Boolean To (0,1)(Boolean="3 3") -> (0, 1=w841:i16)
                  n643 = Boolean To (0,1)(Boolean="3 4") -> (0, 1=w840:i16)
                  n644 = Boolean To (0,1)(Boolean="4 1") -> (0, 1=w839:i16)
                  n645 = Boolean To (0,1)(Boolean="4 2") -> (0, 1=w838:i16)
                  n646 = Boolean To (0,1)(Boolean="4 3") -> (0, 1=w837:i16)
                  n647 = Boolean To (0,1)(Boolean="4 4") -> (0, 1=w836:i16)
                  n648 = Boolean To (0,1)(Boolean="5 1") -> (0, 1=w835:i16)
                  n649 = Boolean To (0,1)(Boolean="5 2") -> (0, 1=w834:i16)
                  n650 = Boolean To (0,1)(Boolean="5 3") -> (0, 1=w833:i16)
                  n651 = Boolean To (0,1)(Boolean="5 4") -> (0, 1=w832:i16)
                  n652 = Boolean To (0,1)(Boolean="6 1") -> (0, 1=w831:i16)
                  n653 = Boolean To (0,1)(Boolean="6 2") -> (0, 1=w830:i16)
                  n654 = Boolean To (0,1)(Boolean="6 3") -> (0, 1=w829:i16)
                  n655 = Boolean To (0,1)(Boolean="6 4") -> (0, 1=w828:i16)
                  n656 = Compound Arithmetic op=OR("1 1", "1 2", "1 3", "1 4", "2 1", "2 2", "2 3", "2 4", "3 1", "3 2", "3 3", "3 4", "4 1", "4 2", "4 3", "4 4", "5 1", "5 2", "5 3", "5 4", "6 1", "6 2", "6 3", "6 4") -> (w882:bool)
                  n657 = Boolean To (0,1)(Boolean=w882) -> (0, 1=→"position":i16)
                  n658 = Boolean To (0,1)(Boolean="Button 1") -> (0, 1=w819:i16)
                  n659 = Boolean To (0,1)(Boolean="Button 2") -> (0, 1=w818:i16)
                  n660 = Boolean To (0,1)(Boolean="Button 3") -> (0, 1=w817:i16)
                  n661 = Boolean To (0,1)(Boolean="Button 4") -> (0, 1=w816:i16)
                  n662 = Boolean To (0,1)(Boolean="Button 5") -> (0, 1=w815:i16)
                  n663 = Compound Arithmetic op=OR(w819, w818, w817, w816, w815) -> (→"Extra":i16)
                }
                frame #3 {
                  n664 = Compound Arithmetic op=OR("ADrive", "ADrive 2", "ADrive 3", "ADrive 4", "ADrive 5", "ADrive 6", "ADrive 7", "ADrive 8", "ADrive 9", "ADrive 10", "ADrive 11", "ADrive 12") -> (w945:bool)
                  n665 = Compound Arithmetic op=OR("SWADrive", "SWADrive 2", "SWADrive 3", "SWADrive 4", "SWADrive 5", "SWADrive 6", "SWADrive 7", "SWADrive 8", "SWADrive 9", "SWADrive 10", "SWADrive 11", "SWADrive 12") -> (w906:bool)
                  n666 = Boolean To (0,1)(Boolean=w945) -> (0, 1=w893:i16)
                  n667 = Boolean To (0,1)(Boolean=w906) -> (0, 1=w891:i16)
                  n668 = Compound Arithmetic op=OR("DDrive", "DDrive 2", "DDrive 3", "DDrive 4", "DDrive 5", "DDrive 6", "DDrive 7", "DDrive 8", "DDrive 9", "DDrive 10", "DDrive 11", "DDrive 12") -> (w932:bool)
                  n669 = Compound Arithmetic op=OR("SWDDrive", "SWDDrive 2", "SWDDrive 3", "SWDDrive 4", "SWDDrive 5", "SWDDrive 6", "SWDDrive 7", "SWDDrive 8", "SWDDrive 9", "SWDDrive 10", "SWDDrive 11", "SWDDrive 12") -> (w919:bool)
                  n670 = Boolean To (0,1)(Boolean=w932) -> (0, 1=w892:i16)
                  n671 = Boolean To (0,1)(Boolean=w919) -> (0, 1=w890:i16)
                }
                frame #4 {
                  n672 = Compound Arithmetic op=OR("Chop", "Chop 2", "Chop 3", "Chop 4", "Chop 5", "Chop 6", "Chop 7", "Chop 8", "Chop 9", "Chop 10", "Chop 11", "Chop 12") -> (w985:bool)
                  n673 = Boolean To (0,1)(Boolean=w985) -> (0, 1=w947:i16)
                  n674 = Compound Arithmetic op=OR("lob 13", "lob 2", "lob 3", "lob 4", "lob 5", "lob 6", "lob 7", "lob 8", "lob 9", "lob 10", "lob 11", "lob 12") -> (w986:bool)
                  n675 = Compound Arithmetic op=OR("Drop", "Drop 2", "Drop 3", "Drop 4", "Drop 5", "Drop 6", "Drop 7", "Drop 8", "Drop 9", "Drop 10", "Drop 11", "Drop 12") -> (w987:bool)
                  n676 = Boolean To (0,1)(Boolean=w987) -> (0, 1=w948:i16)
                  n677 = Boolean To (0,1)(Boolean=w986) -> (0, 1=w946:i16)
                }
                frame #5 {
                  n678 = Compound Arithmetic op=OR("Boast 2", "Boast 4", "Boast 6", "Boast 8", "Boast 10", "Boast 12") -> (w1009:bool)
                  n679 = Boolean To (0,1)(Boolean=w1009) -> (0, 1=w989:i16)
                  n680 = Compound Arithmetic op=OR("Smash", "Smash 2", "Smash 3", "Smash 4", "Smash 5", "Smash 6", "Smash 7", "Smash 8", "Smash 9", "Smash 10", "Smash 11", "Smash 12") -> (w1016:bool)
                  n681 = Compound Arithmetic op=OR("Boast", "Boast 3", "Boast 5", "Boast 7", "Boast 9", "Boast 11") -> (w1017:bool)
                  n682 = Boolean To (0,1)(Boolean=w1017) -> (0, 1=w990:i16)
                  n683 = Boolean To (0,1)(Boolean=w1016) -> (0, 1=w988:i16)
                }
                frame #6 {
                  # "forehand"
                  n684 = local read "Smash 10"() -> (w1052:bool)
                  n685 = local read "Chop 10"() -> (w1064:bool)
                  n686 = local read "Smash 2"() -> (w1056:bool)
                  n687 = local read "Smash 5"() -> (w1055:bool)
                  n688 = local read "Smash 6"() -> (w1054:bool)
                  n689 = local read "Smash 9"() -> (w1053:bool)
                  n690 = local read "Boast 10"() -> (w1046:bool)
                  n691 = local read "Drop 10"() -> (w1070:bool)
                  n692 = local read "Chop 2"() -> (w1068:bool)
                  n693 = local read "Chop 5"() -> (w1067:bool)
                  n694 = local read "Chop 6"() -> (w1066:bool)
                  n695 = local read "Chop 9"() -> (w1065:bool)
                  n696 = local read "Boast 2"() -> (w1050:bool)
                  n697 = local read "Boast 5"() -> (w1049:bool)
                  n698 = local read "Boast 6"() -> (w1048:bool)
                  n699 = local read "Boast 9"() -> (w1047:bool)
                  n700 = local read "Drop 2"() -> (w1074:bool)
                  n701 = local read "Drop 5"() -> (w1073:bool)
                  n702 = local read "Drop 6"() -> (w1072:bool)
                  n703 = local read "Drop 9"() -> (w1071:bool)
                  n704 = local read "Smash"() -> (w1057:bool)
                  n705 = local read "lob 10"() -> (w1058:bool)
                  n706 = local read "Chop"() -> (w1069:bool)
                  n707 = local read "Boast"() -> (w1051:bool)
                  n708 = local read "Drop"() -> (w1075:bool)
                  n709 = local read "lob 2"() -> (w1062:bool)
                  n710 = local read "lob 5"() -> (w1061:bool)
                  n711 = local read "lob 6"() -> (w1060:bool)
                  n712 = local read "lob 9"() -> (w1059:bool)
                  n713 = local read "lob 13"() -> (w1063:bool)
                  n714 = Compound Arithmetic op=OR(w1075, w1074, w1073, w1072, w1071, w1070, w1069, w1068, w1067, w1066, w1065, w1064, w1063, w1062, w1061, w1060, w1059, w1058, w1057, w1056, w1055, w1054, w1053, w1052, w1051, w1050, w1049, w1048, w1047, w1046) -> (w1019:bool)
                  n715 = local read "SWADrive 10"() -> (w1039:bool)
                  n716 = local read "SWDDrive 10"() -> (w1045:bool)
                  n717 = local read "SWADrive 2"() -> (w1035:bool)
                  n718 = local read "SWADrive 5"() -> (w1036:bool)
                  n719 = local read "SWADrive 6"() -> (w1037:bool)
                  n720 = local read "SWADrive 9"() -> (w1038:bool)
                  n721 = local read "SWDDrive 2"() -> (w1041:bool)
                  n722 = local read "SWDDrive 5"() -> (w1042:bool)
                  n723 = local read "SWDDrive 6"() -> (w1043:bool)
                  n724 = local read "SWDDrive 9"() -> (w1044:bool)
                  n725 = local read "SWADrive"() -> (w1034:bool)
                  n726 = local read "SWDDrive"() -> (w1040:bool)
                  n727 = local read "ADrive 10"() -> (w1027:bool)
                  n728 = local read "DDrive 10"() -> (w1033:bool)
                  n729 = local read "ADrive 2"() -> (w1023:bool)
                  n730 = local read "ADrive 5"() -> (w1024:bool)
                  n731 = local read "ADrive 6"() -> (w1025:bool)
                  n732 = local read "ADrive 9"() -> (w1026:bool)
                  n733 = local read "DDrive 2"() -> (w1029:bool)
                  n734 = local read "DDrive 5"() -> (w1030:bool)
                  n735 = local read "DDrive 6"() -> (w1031:bool)
                  n736 = local read "DDrive 9"() -> (w1032:bool)
                  n737 = local read "ADrive"() -> (w1022:bool)
                  n738 = local read "DDrive"() -> (w1028:bool)
                  n739 = Compound Arithmetic op=OR(w1022, w1023, w1024, w1025, w1026, w1027, w1028, w1029, w1030, w1031, w1032, w1033, w1034, w1035, w1036, w1037, w1038, w1039, w1040, w1041, w1042, w1043, w1044, w1045) -> (w1020:bool)
                  n740 = Or(x=w1019, y=w1020) -> (x .or. y?=w1021:bool)
                  n741 = Boolean To (0,1)(Boolean=w1021) -> (0, 1=w1018:i16)
                }
                frame #7 {
                  # "backhand"
                  n742 = local read "Smash 11"() -> (w1108:bool)
                  n743 = local read "Smash 12"() -> (w1107:bool)
                  n744 = local read "Chop 11"() -> (w1120:bool)
                  n745 = local read "Chop 12"() -> (w1119:bool)
                  n746 = local read "Smash 3"() -> (w1112:bool)
                  n747 = local read "Smash 4"() -> (w1111:bool)
                  n748 = local read "Smash 7"() -> (w1110:bool)
                  n749 = local read "Smash 8"() -> (w1109:bool)
                  n750 = local read "Boast 11"() -> (w1102:bool)
                  n751 = local read "Boast 12"() -> (w1101:bool)
                  n752 = local read "Drop 11"() -> (w1126:bool)
                  n753 = local read "Drop 12"() -> (w1125:bool)
                  n754 = local read "Chop 3"() -> (w1124:bool)
                  n755 = local read "Chop 4"() -> (w1123:bool)
                  n756 = local read "Chop 7"() -> (w1122:bool)
                  n757 = local read "Chop 8"() -> (w1121:bool)
                  n758 = local read "Boast 3"() -> (w1106:bool)
                  n759 = local read "Boast 4"() -> (w1105:bool)
                  n760 = local read "Boast 7"() -> (w1104:bool)
                  n761 = local read "Boast 8"() -> (w1103:bool)
                  n762 = local read "Drop 3"() -> (w1130:bool)
                  n763 = local read "Drop 4"() -> (w1129:bool)
                  n764 = local read "Drop 7"() -> (w1128:bool)
                  n765 = local read "Drop 8"() -> (w1127:bool)
                  n766 = local read "lob 11"() -> (w1114:bool)
                  n767 = local read "lob 12"() -> (w1113:bool)
                  n768 = local read "lob 3"() -> (w1118:bool)
                  n769 = local read "lob 4"() -> (w1117:bool)
                  n770 = local read "lob 7"() -> (w1116:bool)
                  n771 = local read "lob 8"() -> (w1115:bool)
                  n772 = Compound Arithmetic op=OR(w1130, w1129, w1128, w1127, w1126, w1125, w1124, w1123, w1122, w1121, w1120, w1119, w1118, w1117, w1116, w1115, w1114, w1113, w1112, w1111, w1110, w1109, w1108, w1107, w1106, w1105, w1104, w1103, w1102, w1101) -> (w1131:bool)
                  n773 = local read "SWADrive 11"() -> (w1084:bool)
                  n774 = local read "SWADrive 12"() -> (w1083:bool)
                  n775 = local read "SWDDrive 11"() -> (w1078:bool)
                  n776 = local read "SWDDrive 12"() -> (w1077:bool)
                  n777 = local read "SWADrive 3"() -> (w1088:bool)
                  n778 = local read "SWADrive 4"() -> (w1087:bool)
                  n779 = local read "SWADrive 7"() -> (w1086:bool)
                  n780 = local read "SWADrive 8"() -> (w1085:bool)
                  n781 = local read "SWDDrive 3"() -> (w1082:bool)
                  n782 = local read "SWDDrive 4"() -> (w1081:bool)
                  n783 = local read "SWDDrive 7"() -> (w1080:bool)
                  n784 = local read "SWDDrive 8"() -> (w1079:bool)
                  n785 = local read "ADrive 11"() -> (w1096:bool)
                  n786 = local read "ADrive 12"() -> (w1095:bool)
                  n787 = local read "DDrive 11"() -> (w1090:bool)
                  n788 = local read "DDrive 12"() -> (w1089:bool)
                  n789 = local read "ADrive 3"() -> (w1100:bool)
                  n790 = local read "ADrive 4"() -> (w1099:bool)
                  n791 = local read "ADrive 7"() -> (w1098:bool)
                  n792 = local read "ADrive 8"() -> (w1097:bool)
                  n793 = local read "DDrive 3"() -> (w1094:bool)
                  n794 = local read "DDrive 4"() -> (w1093:bool)
                  n795 = local read "DDrive 7"() -> (w1092:bool)
                  n796 = local read "DDrive 8"() -> (w1091:bool)
                  n797 = Compound Arithmetic op=OR(w1100, w1099, w1098, w1097, w1096, w1095, w1094, w1093, w1092, w1091, w1090, w1089, w1088, w1087, w1086, w1085, w1084, w1083, w1082, w1081, w1080, w1079, w1078, w1077) -> (w1132:bool)
                  n798 = Or(x=w1131, y=w1132) -> (x .or. y?=w1133:bool)
                  n799 = Boolean To (0,1)(Boolean=w1133) -> (0, 1=w1076:i16)
                }
                frame #8 {
                  # "straight"
                  n800 = local read "Smash 11"() -> (w1159:bool)
                  n801 = local read "Chop 11"() -> (w1171:bool)
                  n802 = local read "Smash 3"() -> (w1163:bool)
                  n803 = local read "Smash 5"() -> (w1162:bool)
                  n804 = local read "Smash 7"() -> (w1161:bool)
                  n805 = local read "Smash 9"() -> (w1160:bool)
                  n806 = local read "Drop 11"() -> (w1177:bool)
                  n807 = local read "Chop 3"() -> (w1175:bool)
                  n808 = local read "Chop 5"() -> (w1174:bool)
                  n809 = local read "Chop 7"() -> (w1173:bool)
                  n810 = local read "Chop 9"() -> (w1172:bool)
                  n811 = local read "Drop 3"() -> (w1181:bool)
                  n812 = local read "Drop 5"() -> (w1180:bool)
                  n813 = local read "Drop 7"() -> (w1179:bool)
                  n814 = local read "Drop 9"() -> (w1178:bool)
                  n815 = local read "Smash"() -> (w1164:bool)
                  n816 = local read "lob 11"() -> (w1165:bool)
                  n817 = local read "Chop"() -> (w1176:bool)
                  n818 = local read "Drop"() -> (w1182:bool)
                  n819 = local read "lob 3"() -> (w1169:bool)
                  n820 = local read "lob 5"() -> (w1168:bool)
                  n821 = local read "lob 7"() -> (w1167:bool)
                  n822 = local read "lob 9"() -> (w1166:bool)
                  n823 = local read "lob 13"() -> (w1170:bool)
                  n824 = Compound Arithmetic op=OR(w1182, w1181, w1180, w1179, w1178, w1177, w1176, w1175, w1174, w1173, w1172, w1171, w1170, w1169, w1168, w1167, w1166, w1165, w1164, w1163, w1162, w1161, w1160, w1159) -> (w1183:bool)
                  n825 = local read "SWADrive 11"() -> (w1141:bool)
                  n826 = local read "SWDDrive 11"() -> (w1135:bool)
                  n827 = local read "SWADrive 3"() -> (w1145:bool)
                  n828 = local read "SWADrive 5"() -> (w1144:bool)
                  n829 = local read "SWADrive 7"() -> (w1143:bool)
                  n830 = local read "SWADrive 9"() -> (w1142:bool)
                  n831 = local read "SWDDrive 3"() -> (w1139:bool)
                  n832 = local read "SWDDrive 5"() -> (w1138:bool)
                  n833 = local read "SWDDrive 7"() -> (w1137:bool)
                  n834 = local read "SWDDrive 9"() -> (w1136:bool)
                  n835 = local read "SWADrive"() -> (w1146:bool)
                  n836 = local read "SWDDrive"() -> (w1140:bool)
                  n837 = local read "ADrive 11"() -> (w1153:bool)
                  n838 = local read "DDrive 11"() -> (w1147:bool)
                  n839 = local read "ADrive 3"() -> (w1157:bool)
                  n840 = local read "ADrive 5"() -> (w1156:bool)
                  n841 = local read "ADrive 7"() -> (w1155:bool)
                  n842 = local read "ADrive 9"() -> (w1154:bool)
                  n843 = local read "DDrive 3"() -> (w1151:bool)
                  n844 = local read "DDrive 5"() -> (w1150:bool)
                  n845 = local read "DDrive 7"() -> (w1149:bool)
                  n846 = local read "DDrive 9"() -> (w1148:bool)
                  n847 = local read "ADrive"() -> (w1158:bool)
                  n848 = local read "DDrive"() -> (w1152:bool)
                  n849 = Compound Arithmetic op=OR(w1158, w1157, w1156, w1155, w1154, w1153, w1152, w1151, w1150, w1149, w1148, w1147, w1146, w1145, w1144, w1143, w1142, w1141, w1140, w1139, w1138, w1137, w1136, w1135) -> (w1184:bool)
                  n850 = Or(x=w1183, y=w1184) -> (x .or. y?=w1185:bool)
                  n851 = Boolean To (0,1)(Boolean=w1185) -> (0, 1=w1134:i16)
                  "Straight" <- w1134
                }
                frame #9 {
                  # "cross"
                  n852 = local read "Smash 10"() -> (w1225:bool)
                  n853 = local read "Smash 12"() -> (w1224:bool)
                  n854 = local read "Chop 10"() -> (w1237:bool)
                  n855 = local read "Chop 12"() -> (w1236:bool)
                  n856 = local read "Smash 2"() -> (w1229:bool)
                  n857 = local read "Smash 4"() -> (w1228:bool)
                  n858 = local read "Smash 6"() -> (w1227:bool)
                  n859 = local read "Smash 8"() -> (w1226:bool)
                  n860 = local read "Boast 10"() -> (w1214:bool)
                  n861 = local read "Boast 11"() -> (w1213:bool)
                  n862 = local read "Boast 12"() -> (w1212:bool)
                  n863 = local read "Drop 10"() -> (w1243:bool)
                  n864 = local read "Drop 12"() -> (w1242:bool)
                  n865 = local read "Chop 2"() -> (w1241:bool)
                  n866 = local read "Chop 4"() -> (w1240:bool)
                  n867 = local read "Chop 6"() -> (w1239:bool)
                  n868 = local read "Chop 8"() -> (w1238:bool)
                  n869 = local read "Boast 2"() -> (w1222:bool)
                  n870 = local read "Boast 3"() -> (w1221:bool)
                  n871 = local read "Boast 4"() -> (w1220:bool)
                  n872 = local read "Boast 5"() -> (w1219:bool)
                  n873 = local read "Boast 6"() -> (w1218:bool)
                  n874 = local read "Boast 7"() -> (w1217:bool)
                  n875 = local read "Boast 8"() -> (w1216:bool)
                  n876 = local read "Boast 9"() -> (w1215:bool)
                  n877 = local read "Drop 2"() -> (w1247:bool)
                  n878 = local read "Drop 4"() -> (w1246:bool)
                  n879 = local read "Drop 6"() -> (w1245:bool)
                  n880 = local read "Drop 8"() -> (w1244:bool)
                  n881 = local read "lob 10"() -> (w1231:bool)
                  n882 = local read "lob 12"() -> (w1230:bool)
                  n883 = local read "Boast"() -> (w1223:bool)
                  n884 = local read "lob 2"() -> (w1235:bool)
                  n885 = local read "lob 4"() -> (w1234:bool)
                  n886 = local read "lob 6"() -> (w1233:bool)
                  n887 = local read "lob 8"() -> (w1232:bool)
                  n888 = Compound Arithmetic op=OR(w1247, w1246, w1245, w1244, w1243, w1242, w1241, w1240, w1239, w1238, w1237, w1236, w1235, w1234, w1233, w1232, w1231, w1230, w1229, w1228, w1227, w1226, w1225, w1224, w1223, w1222, w1221, w1220, w1219, w1218, w1217, w1216, w1215, w1214, w1213, w1212) -> (w1187:bool)
                  n889 = local read "SWADrive 10"() -> (w1195:bool)
                  n890 = local read "SWADrive 12"() -> (w1194:bool)
                  n891 = local read "SWDDrive 10"() -> (w1189:bool)
                  n892 = local read "SWDDrive 12"() -> (w1188:bool)
                  n893 = local read "SWADrive 2"() -> (w1199:bool)
                  n894 = local read "SWADrive 4"() -> (w1198:bool)
                  n895 = local read "SWADrive 6"() -> (w1197:bool)
                  n896 = local read "SWADrive 8"() -> (w1196:bool)
                  n897 = local read "SWDDrive 2"() -> (w1193:bool)
                  n898 = local read "SWDDrive 4"() -> (w1192:bool)
                  n899 = local read "SWDDrive 6"() -> (w1191:bool)
                  n900 = local read "SWDDrive 8"() -> (w1190:bool)
                  n901 = local read "ADrive 10"() -> (w1207:bool)
                  n902 = local read "ADrive 12"() -> (w1206:bool)
                  n903 = local read "DDrive 10"() -> (w1201:bool)
                  n904 = local read "DDrive 12"() -> (w1200:bool)
                  n905 = local read "ADrive 2"() -> (w1211:bool)
                  n906 = local read "ADrive 4"() -> (w1210:bool)
                  n907 = local read "ADrive 6"() -> (w1209:bool)
                  n908 = local read "ADrive 8"() -> (w1208:bool)
                  n909 = local read "DDrive 2"() -> (w1205:bool)
                  n910 = local read "DDrive 4"() -> (w1204:bool)
                  n911 = local read "DDrive 6"() -> (w1203:bool)
                  n912 = local read "DDrive 8"() -> (w1202:bool)
                  n913 = Compound Arithmetic op=OR(w1211, w1210, w1209, w1208, w1207, w1206, w1205, w1204, w1203, w1202, w1201, w1200, w1199, w1198, w1197, w1196, w1195, w1194, w1193, w1192, w1191, w1190, w1189, w1188) -> (w1248:bool)
                  n914 = Or(x=w1187, y=w1248) -> (x .or. y?=w1249:bool)
                  n915 = Boolean To (0,1)(Boolean=w1249) -> (0, 1=w1186:i16)
                  "Cross" <- w1186
                }
                frame #10 {
                  # "bounce"
                  n916 = local read "Smash 2"() -> (w1257:bool)
                  n917 = local read "Smash 3"() -> (w1256:bool)
                  n918 = local read "Smash 4"() -> (w1255:bool)
                  n919 = local read "Chop 2"() -> (w1281:bool)
                  n920 = local read "Chop 3"() -> (w1280:bool)
                  n921 = local read "Chop 4"() -> (w1279:bool)
                  n922 = local read "Boast 2"() -> (w1253:bool)
                  n923 = local read "Boast 3"() -> (w1252:bool)
                  n924 = local read "Boast 4"() -> (w1251:bool)
                  n925 = local read "Drop 2"() -> (w1285:bool)
                  n926 = local read "Drop 3"() -> (w1284:bool)
                  n927 = local read "Drop 4"() -> (w1283:bool)
                  n928 = local read "Smash"() -> (w1258:bool)
                  n929 = local read "Chop"() -> (w1282:bool)
                  n930 = local read "Boast"() -> (w1254:bool)
                  n931 = local read "Drop"() -> (w1286:bool)
                  n932 = local read "lob 2"() -> (w1260:bool)
                  n933 = local read "lob 3"() -> (w1261:bool)
                  n934 = local read "lob 4"() -> (w1259:bool)
                  n935 = local read "lob 13"() -> (w1262:bool)
                  n936 = Compound Arithmetic op=OR(w1286, w1285, w1284, w1283, w1282, w1281, w1280, w1279, w1262, w1260, w1261, w1259, w1258, w1257, w1256, w1255, w1254, w1253, w1252, w1251) -> (w1287:bool)
                  n937 = local read "SWADrive 2"() -> (w1269:bool)
                  n938 = local read "SWADrive 3"() -> (w1268:bool)
                  n939 = local read "SWADrive 4"() -> (w1267:bool)
                  n940 = local read "SWDDrive 2"() -> (w1265:bool)
                  n941 = local read "SWDDrive 3"() -> (w1264:bool)
                  n942 = local read "SWDDrive 4"() -> (w1263:bool)
                  n943 = local read "SWADrive"() -> (w1270:bool)
                  n944 = local read "SWDDrive"() -> (w1266:bool)
                  n945 = local read "ADrive 2"() -> (w1277:bool)
                  n946 = local read "ADrive 3"() -> (w1276:bool)
                  n947 = local read "ADrive 4"() -> (w1275:bool)
                  n948 = local read "DDrive 2"() -> (w1273:bool)
                  n949 = local read "DDrive 3"() -> (w1272:bool)
                  n950 = local read "DDrive 4"() -> (w1271:bool)
                  n951 = local read "ADrive"() -> (w1278:bool)
                  n952 = local read "DDrive"() -> (w1274:bool)
                  n953 = Compound Arithmetic op=OR(w1278, w1277, w1276, w1275, w1274, w1273, w1272, w1271, w1270, w1269, w1268, w1267, w1266, w1265, w1264, w1263) -> (w1288:bool)
                  n954 = Or(x=w1287, y=w1288) -> (x .or. y?=w1289:bool)
                  n955 = Boolean To (0,1)(Boolean=w1289) -> (0, 1=w1250:i16)
                }
                frame #11 {
                  # "volley"
                  n956 = local read "Smash 5"() -> (w1314:bool)
                  n957 = local read "Smash 6"() -> (w1313:bool)
                  n958 = local read "Smash 7"() -> (w1312:bool)
                  n959 = local read "Smash 8"() -> (w1311:bool)
                  n960 = local read "Chop 5"() -> (w1322:bool)
                  n961 = local read "Chop 6"() -> (w1321:bool)
                  n962 = local read "Chop 7"() -> (w1320:bool)
                  n963 = local read "Chop 8"() -> (w1319:bool)
                  n964 = local read "Boast 5"() -> (w1310:bool)
                  n965 = local read "Boast 6"() -> (w1309:bool)
                  n966 = local read "Boast 7"() -> (w1308:bool)
                  n967 = local read "Boast 8"() -> (w1307:bool)
                  n968 = local read "Drop 5"() -> (w1326:bool)
                  n969 = local read "Drop 6"() -> (w1325:bool)
                  n970 = local read "Drop 7"() -> (w1324:bool)
                  n971 = local read "Drop 8"() -> (w1323:bool)
                  n972 = local read "lob 5"() -> (w1318:bool)
                  n973 = local read "lob 6"() -> (w1317:bool)
                  n974 = local read "lob 7"() -> (w1316:bool)
                  n975 = local read "lob 8"() -> (w1315:bool)
                  n976 = Compound Arithmetic op=OR(w1326, w1325, w1324, w1323, w1322, w1321, w1320, w1319, w1318, w1317, w1316, w1315, w1314, w1313, w1312, w1311, w1310, w1309, w1308, w1307) -> (w1327:bool)
                  n977 = local read "SWADrive 5"() -> (w1298:bool)
                  n978 = local read "SWADrive 6"() -> (w1297:bool)
                  n979 = local read "SWADrive 7"() -> (w1296:bool)
                  n980 = local read "SWADrive 8"() -> (w1295:bool)
                  n981 = local read "SWDDrive 5"() -> (w1294:bool)
                  n982 = local read "SWDDrive 6"() -> (w1293:bool)
                  n983 = local read "SWDDrive 7"() -> (w1292:bool)
                  n984 = local read "SWDDrive 8"() -> (w1291:bool)
                  n985 = local read "ADrive 5"() -> (w1306:bool)
                  n986 = local read "ADrive 6"() -> (w1305:bool)
                  n987 = local read "ADrive 7"() -> (w1304:bool)
                  n988 = local read "ADrive 8"() -> (w1303:bool)
                  n989 = local read "DDrive 5"() -> (w1302:bool)
                  n990 = local read "DDrive 6"() -> (w1301:bool)
                  n991 = local read "DDrive 7"() -> (w1300:bool)
                  n992 = local read "DDrive 8"() -> (w1299:bool)
                  n993 = Compound Arithmetic op=OR(w1306, w1305, w1304, w1303, w1302, w1301, w1300, w1299, w1298, w1297, w1296, w1295, w1294, w1293, w1292, w1291) -> (w1328:bool)
                  n994 = Or(x=w1327, y=w1328) -> (x .or. y?=w1329:bool)
                  n995 = Boolean To (0,1)(Boolean=w1329) -> (0, 1=w1290:i16)
                }
                frame #12 {
                  # "half volley"
                  n996 = local read "Smash 10"() -> (w1353:bool)
                  n997 = local read "Smash 11"() -> (w1352:bool)
                  n998 = local read "Smash 12"() -> (w1351:bool)
                  n999 = local read "Chop 10"() -> (w1361:bool)
                  n1000 = local read "Chop 11"() -> (w1360:bool)
                  n1001 = local read "Chop 12"() -> (w1359:bool)
                  n1002 = local read "Smash 9"() -> (w1354:bool)
                  n1003 = local read "Boast 10"() -> (w1349:bool)
                  n1004 = local read "Boast 11"() -> (w1348:bool)
                  n1005 = local read "Boast 12"() -> (w1347:bool)
                  n1006 = local read "Drop 10"() -> (w1365:bool)
                  n1007 = local read "Drop 11"() -> (w1364:bool)
                  n1008 = local read "Drop 12"() -> (w1363:bool)
                  n1009 = local read "Chop 9"() -> (w1362:bool)
                  n1010 = local read "Boast 9"() -> (w1350:bool)
                  n1011 = local read "Drop 9"() -> (w1366:bool)
                  n1012 = local read "lob 10"() -> (w1357:bool)
                  n1013 = local read "lob 11"() -> (w1356:bool)
                  n1014 = local read "lob 12"() -> (w1355:bool)
                  n1015 = local read "lob 9"() -> (w1358:bool)
                  n1016 = Compound Arithmetic op=OR(w1366, w1365, w1364, w1363, w1362, w1361, w1360, w1359, w1358, w1357, w1356, w1355, w1354, w1353, w1352, w1351, w1350, w1349, w1348, w1347) -> (w1367:bool)
                  n1017 = local read "SWADrive 10"() -> (w1337:bool)
                  n1018 = local read "SWADrive 11"() -> (w1336:bool)
                  n1019 = local read "SWADrive 12"() -> (w1335:bool)
                  n1020 = local read "SWDDrive 10"() -> (w1333:bool)
                  n1021 = local read "SWDDrive 11"() -> (w1332:bool)
                  n1022 = local read "SWDDrive 12"() -> (w1331:bool)
                  n1023 = local read "SWADrive 9"() -> (w1338:bool)
                  n1024 = local read "SWDDrive 9"() -> (w1334:bool)
                  n1025 = local read "ADrive 10"() -> (w1345:bool)
                  n1026 = local read "ADrive 11"() -> (w1344:bool)
                  n1027 = local read "ADrive 12"() -> (w1343:bool)
                  n1028 = local read "DDrive 10"() -> (w1341:bool)
                  n1029 = local read "DDrive 11"() -> (w1340:bool)
                  n1030 = local read "DDrive 12"() -> (w1339:bool)
                  n1031 = local read "ADrive 9"() -> (w1346:bool)
                  n1032 = local read "DDrive 9"() -> (w1342:bool)
                  n1033 = Compound Arithmetic op=OR(w1346, w1345, w1344, w1343, w1342, w1341, w1340, w1339, w1338, w1337, w1336, w1335, w1334, w1333, w1332, w1331) -> (w1368:bool)
                  n1034 = Or(x=w1367, y=w1368) -> (x .or. y?=w1369:bool)
                  n1035 = Boolean To (0,1)(Boolean=w1369) -> (0, 1=w1330:i16)
                }
                frame #13 {
                  n1036 = local read "Player1/Player2"() -> (w1380:bool[])
                  n1037 = Index Array(array=w1380) -> (element #1=w1381:bool, element #2=w1382:bool)  [unwired: 2 in]
                  n1038 = Boolean To (0,1)(Boolean=w1382) -> (0, 1=w1370:i16)
                  n1039 = Boolean To (0,1)(Boolean=w1381) -> (0, 1=w1371:i16)
                  n1040 = Compound Arithmetic op=OR("Service1", "Service2", "S1", "S2", "S3", "S4", "S5", "S6") -> (w1392:bool)
                  n1041 = Boolean To (0,1)(Boolean=w1392) -> (0, 1=→"Service":i16)
                  n1042 = Boolean To (0,1)(Boolean="Service1") -> (0, 1=w1379:i16)
                  n1043 = Boolean To (0,1)(Boolean="Service2") -> (0, 1=w1378:i16)
                  n1044 = Boolean To (0,1)(Boolean="S1") -> (0, 1=w1377:i16)
                  n1045 = Boolean To (0,1)(Boolean="S2") -> (0, 1=w1376:i16)
                  n1046 = Boolean To (0,1)(Boolean="S3") -> (0, 1=w1375:i16)
                  n1047 = Boolean To (0,1)(Boolean="S4") -> (0, 1=w1374:i16)
                  n1048 = Boolean To (0,1)(Boolean="S5") -> (0, 1=w1373:i16)
                  n1049 = Boolean To (0,1)(Boolean="S6") -> (0, 1=w1372:i16)
                }
                frame #14 {
                  w1408 = 0 ("disabled index (col)")
                  n1050 = Index Array(array=w1430, index (col) #1=51 ("disabled index (col)"), index (col) #2=52 ("index (col)"), index (col) #3=0 ("index (col)")) -> (element #1=w1419:i64[], element #2=w1418:i64[], element #3=w1421:i64[])  [unwired: 3 in]
                  n1051 = Or(x=w1419, y=w1418) -> (x .or. y?=w1426:i64[])
                  n1052 = Reverse 1D Array(array=w1426) -> (reversed array=w1425:i64[])
                  n1053 = Reverse 1D Array(array=w1421) -> (reversed array=w1423:i64[])
                  n1054 = Compound Arithmetic op=OR("Expected Winner1", "Unexpected Winner1", "Stroke1", "Forced Error2", "Unforced Error2", "Nolet2") -> (w1440:bool)
                  n1055 = Search 1D Array(1D array=w1425, element=i64 1) -> (index of element=w1422:i32)  [unwired: 1 in]
                  n1056 = Boolean To (0,1)(Boolean=w1440) -> (0, 1=w1406:i16)
                  n1057 = Compound Arithmetic op=OR("Expected Winner2", "Unexpected Winner2", "Stroke2", "Forced Error1", "Unforced Error1", "Nolet1") -> (w1439:bool)
                  n1058 = Boolean To (0,1)(Boolean="Expected Winner1") -> (0, 1=w1393:i16)
                  n1059 = Boolean To (0,1)(Boolean="Expected Winner2") -> (0, 1=w1394:i16)
                  n1060 = Boolean To (0,1)(Boolean="Unexpected Winner1") -> (0, 1=w1395:i16)
                  n1061 = Boolean To (0,1)(Boolean="Unexpected Winner2") -> (0, 1=w1396:i16)
                  n1062 = Boolean To (0,1)(Boolean="Stroke1") -> (0, 1=w1397:i16)
                  n1063 = Boolean To (0,1)(Boolean="Stroke2") -> (0, 1=w1398:i16)
                  n1064 = Boolean To (0,1)(Boolean="Forced Error1") -> (0, 1=w1399:i16)
                  n1065 = Boolean To (0,1)(Boolean="Forced Error2") -> (0, 1=w1400:i16)
                  n1066 = Boolean To (0,1)(Boolean="Unforced Error1") -> (0, 1=w1401:i16)
                  n1067 = Boolean To (0,1)(Boolean="Unforced Error2") -> (0, 1=w1402:i16)
                  n1068 = Boolean To (0,1)(Boolean="Nolet1") -> (0, 1=w1403:i16)
                  n1069 = Boolean To (0,1)(Boolean="Nolet2") -> (0, 1=w1404:i16)
                  n1070 = Boolean To (0,1)(Boolean="Let") -> (0, 1=w1405:i16)
                  n1071 = Index Array(array=w1423, index=w1422) -> (element=w1420:i64)
                  n1072 = Boolean To (0,1)(Boolean=w1439) -> (0, 1=w1407:i16)
                  n1073 = Search 1D Array(1D array=w1421, element=w1420) -> (index of element=w1417:i32)  [unwired: 1 in]
                  n1074 = Not Equal To 0?(x=w1406) -> (x != 0?=w1432:bool)
                  n1075 = Not Equal To 0?(x=w1407) -> (x != 0?=w1431:bool)
                  n1076 = Build Array(w1432, w1431) -> (w1409:bool[])
                  n1077 = Index Array(array=w1418, index=w1417) -> (element=w1413:i64)
                  n1078 = Index Array(array=w1419, index=w1417) -> (element=w1414:i64)
                  n1079 = Not Equal To 0?(x=w1414) -> (x != 0?=w1415:bool)
                  n1080 = Not Equal To 0?(x=w1413) -> (x != 0?=w1416:bool)
                  n1081 = Build Array(w1415, w1416) -> (w1410:bool[])
                  n1082 = Select(t=w1410, s="Let", f=w1409) -> (s? t:f=w1412:bool[])
                  n1083 = local write "Score change"(w1412) -> ()
                }
                frame #15 {
                  w1447 = FALSE ("4 6")
                  n1084 = local read "Service"() -> (w1456:i16)
                  n1085 = local read "Cross"() -> (w1455:i16)
                  n1086 = local read "Straight"() -> (w1454:i16)
                  n1087 = local read "position"() -> (w1453:i16)
                  n1088 = local read "Player 1/2"() -> (w1452:i16)
                  n1089 = local read "Extra"() -> (w1451:i16)
                  n1090 = local write "Drop"(w1447) -> ()
                  n1091 = local write "Drop 2"(w1447) -> ()
                  n1092 = local write "Drop 3"(w1447) -> ()
                  n1093 = local write "Drop 4"(w1447) -> ()
                  n1094 = local write "Drop 5"(w1447) -> ()
                  n1095 = local write "Drop 6"(w1447) -> ()
                  n1096 = local write "Drop 7"(w1447) -> ()
                  n1097 = local write "Drop 8"(w1447) -> ()
                  n1098 = local write "Drop 9"(w1447) -> ()
                  n1099 = local write "Drop 10"(w1447) -> ()
                  n1100 = local write "Drop 11"(w1447) -> ()
                  n1101 = local write "Drop 12"(w1447) -> ()
                  n1102 = local write "Chop"(w1447) -> ()
                  n1103 = local write "Chop 2"(w1447) -> ()
                  n1104 = local write "Chop 3"(w1447) -> ()
                  n1105 = local write "Chop 4"(w1447) -> ()
                  n1106 = local write "Chop 5"(w1447) -> ()
                  n1107 = local write "Chop 6"(w1447) -> ()
                  n1108 = local write "Chop 7"(w1447) -> ()
                  n1109 = local write "Chop 8"(w1447) -> ()
                  n1110 = local write "Chop 9"(w1447) -> ()
                  n1111 = local write "Chop 10"(w1447) -> ()
                  n1112 = local write "Chop 11"(w1447) -> ()
                  n1113 = local write "Chop 12"(w1447) -> ()
                  n1114 = Compound Arithmetic op=ADD(w1456, w1455, w1454, w1453, w1452, w1451) -> (w1450:i16)
                  n1115 = Equal To 0?(x=w1450) -> (x = 0?=w1449:bool)
                  n1116 = local write "lob 13"(w1447) -> ()
                  n1117 = local write "lob 2"(w1447) -> ()
                  n1118 = local write "lob 3"(w1447) -> ()
                  n1119 = local write "lob 4"(w1447) -> ()
                  n1120 = local write "lob 5"(w1447) -> ()
                  n1121 = local write "lob 6"(w1447) -> ()
                  n1122 = local write "lob 7"(w1447) -> ()
                  n1123 = local write "lob 8"(w1447) -> ()
                  n1124 = local write "lob 9"(w1447) -> ()
                  n1125 = local write "lob 10"(w1447) -> ()
                  n1126 = local write "lob 11"(w1447) -> ()
                  n1127 = local write "lob 12"(w1447) -> ()
                  n1128 = local write "Smash"(w1447) -> ()
                  n1129 = local write "Smash 2"(w1447) -> ()
                  n1130 = local write "Smash 3"(w1447) -> ()
                  n1131 = local write "Smash 4"(w1447) -> ()
                  n1132 = local write "Smash 5"(w1447) -> ()
                  n1133 = local write "Smash 6"(w1447) -> ()
                  n1134 = local write "Smash 7"(w1447) -> ()
                  n1135 = local write "Smash 8"(w1447) -> ()
                  n1136 = local write "Smash 9"(w1447) -> ()
                  n1137 = local write "Smash 10"(w1447) -> ()
                  n1138 = local write "Smash 11"(w1447) -> ()
                  n1139 = local write "Smash 12"(w1447) -> ()
                  n1140 = case shown="True" "Auto switch" {
                    tunnel: w1449 -> [_ w1457]
                    frame False {
                    }
                    frame True {
                      n1141 = local read "Player1/Player2"() -> (w1463:bool[])
                      n1142 = local read "Player1/Player2"() -> (w1464:bool[])
                      n1143 = Reverse 1D Array(array=w1463) -> (reversed array=w1462:bool[])
                      n1144 = Select(t=w1464, s=w1457, f=w1462) -> (s? t:f=w1458:bool[])
                      n1145 = local read "Score change"() -> (w1460:bool[])
                      n1146 = Or Array Elements(Boolean array=w1460) -> (logical OR=w1461:bool)
                      n1147 = Select(t=w1460, s=w1461, f=w1458) -> (s? t:f=w1459:bool[])
                      n1148 = local write "Player1/Player2"(w1459) -> ()
                    }
                  }
                  n1149 = local write "ADrive"(w1447) -> ()
                  n1150 = local write "ADrive 2"(w1447) -> ()
                  n1151 = local write "ADrive 3"(w1447) -> ()
                  n1152 = local write "ADrive 4"(w1447) -> ()
                  n1153 = local write "ADrive 5"(w1447) -> ()
                  n1154 = local write "ADrive 6"(w1447) -> ()
                  n1155 = local write "ADrive 7"(w1447) -> ()
                  n1156 = local write "ADrive 8"(w1447) -> ()
                  n1157 = local write "ADrive 9"(w1447) -> ()
                  n1158 = local write "ADrive 10"(w1447) -> ()
                  n1159 = local write "ADrive 11"(w1447) -> ()
                  n1160 = local write "ADrive 12"(w1447) -> ()
                  n1161 = local write "DDrive"(w1447) -> ()
                  n1162 = local write "DDrive 2"(w1447) -> ()
                  n1163 = local write "DDrive 3"(w1447) -> ()
                  n1164 = local write "DDrive 4"(w1447) -> ()
                  n1165 = local write "DDrive 5"(w1447) -> ()
                  n1166 = local write "DDrive 6"(w1447) -> ()
                  n1167 = local write "DDrive 7"(w1447) -> ()
                  n1168 = local write "DDrive 8"(w1447) -> ()
                  n1169 = local write "DDrive 9"(w1447) -> ()
                  n1170 = local write "DDrive 10"(w1447) -> ()
                  n1171 = local write "DDrive 11"(w1447) -> ()
                  n1172 = local write "DDrive 12"(w1447) -> ()
                  n1173 = local write "SWADrive"(w1447) -> ()
                  n1174 = local write "SWADrive 2"(w1447) -> ()
                  n1175 = local write "SWADrive 3"(w1447) -> ()
                  n1176 = local write "SWADrive 4"(w1447) -> ()
                  n1177 = local write "SWADrive 5"(w1447) -> ()
                  n1178 = local write "SWADrive 6"(w1447) -> ()
                  n1179 = local write "SWADrive 7"(w1447) -> ()
                  n1180 = local write "SWADrive 8"(w1447) -> ()
                  n1181 = local write "SWADrive 9"(w1447) -> ()
                  n1182 = local write "SWADrive 10"(w1447) -> ()
                  n1183 = local write "SWADrive 11"(w1447) -> ()
                  n1184 = local write "SWADrive 12"(w1447) -> ()
                  n1185 = local write "SWDDrive"(w1447) -> ()
                  n1186 = local write "SWDDrive 2"(w1447) -> ()
                  n1187 = local write "SWDDrive 3"(w1447) -> ()
                  n1188 = local write "SWDDrive 4"(w1447) -> ()
                  n1189 = local write "SWDDrive 5"(w1447) -> ()
                  n1190 = local write "SWDDrive 6"(w1447) -> ()
                  n1191 = local write "SWDDrive 7"(w1447) -> ()
                  n1192 = local write "SWDDrive 8"(w1447) -> ()
                  n1193 = local write "SWDDrive 9"(w1447) -> ()
                  n1194 = local write "SWDDrive 10"(w1447) -> ()
                  n1195 = local write "SWDDrive 11"(w1447) -> ()
                  n1196 = local write "SWDDrive 12"(w1447) -> ()
                  n1197 = local write "Boast"(w1447) -> ()
                  n1198 = local write "Boast 2"(w1447) -> ()
                  n1199 = local write "Boast 3"(w1447) -> ()
                  n1200 = local write "Boast 4"(w1447) -> ()
                  n1201 = local write "Boast 5"(w1447) -> ()
                  n1202 = local write "Boast 6"(w1447) -> ()
                  n1203 = local write "Boast 7"(w1447) -> ()
                  n1204 = local write "Boast 8"(w1447) -> ()
                  n1205 = local write "Boast 9"(w1447) -> ()
                  n1206 = local write "Boast 10"(w1447) -> ()
                  n1207 = local write "Boast 11"(w1447) -> ()
                  n1208 = local write "Boast 12"(w1447) -> ()
                  n1209 = local write "4 4"(w1447) -> ()
                  n1210 = local write "4 3"(w1447) -> ()
                  n1211 = local write "4 2"(w1447) -> ()
                  n1212 = local write "4 1"(w1447) -> ()
                  n1213 = local write "3 4"(w1447) -> ()
                  n1214 = local write "3 3"(w1447) -> ()
                  n1215 = local write "3 2"(w1447) -> ()
                  n1216 = local write "3 1"(w1447) -> ()
                  n1217 = local write "2 4"(w1447) -> ()
                  n1218 = local write "2 3"(w1447) -> ()
                  n1219 = local write "2 2"(w1447) -> ()
                  n1220 = local write "2 1"(w1447) -> ()
                  n1221 = local write "1 4"(w1447) -> ()
                  n1222 = local write "1 3"(w1447) -> ()
                  n1223 = local write "1 2"(w1447) -> ()
                  n1224 = local write "1 1"(w1447) -> ()
                  n1225 = local write "5 4"(w1447) -> ()
                  n1226 = local write "5 3"(w1447) -> ()
                  n1227 = local write "5 2"(w1447) -> ()
                  n1228 = local write "5 1"(w1447) -> ()
                  n1229 = local write "6 4"(w1447) -> ()
                  n1230 = local write "6 3"(w1447) -> ()
                  n1231 = local write "6 2"(w1447) -> ()
                  n1232 = local write "6 1"(w1447) -> ()
                  n1233 = local write "S6"(w1447) -> ()
                  n1234 = local write "S5"(w1447) -> ()
                  n1235 = local write "S4"(w1447) -> ()
                  n1236 = local write "S1"(w1447) -> ()
                  n1237 = local write "S2"(w1447) -> ()
                  n1238 = local write "S3"(w1447) -> ()
                  n1239 = local write "Let"(w1447) -> ()
                  n1240 = local write "Unexpected Winner2"(w1447) -> ()
                  n1241 = local write "Unexpected Winner1"(w1447) -> ()
                  n1242 = local write "Expected Winner2"(w1447) -> ()
                  n1243 = local write "Expected Winner1"(w1447) -> ()
                  n1244 = local write "Forced Error2"(w1447) -> ()
                  n1245 = local write "Forced Error1"(w1447) -> ()
                  n1246 = local write "Service2"(w1447) -> ()
                  n1247 = local write "Service1"(w1447) -> ()
                  n1248 = local write "Nolet2"(w1447) -> ()
                  n1249 = local write "Nolet1"(w1447) -> ()
                  n1250 = local write "Stroke2"(w1447) -> ()
                  n1251 = local write "Stroke1"(w1447) -> ()
                  n1252 = local write "Unforced Error2"(w1447) -> ()
                  n1253 = local write "Unforced Error1"(w1447) -> ()
                  n1254 = local write "Player1"(w1447) -> ()
                  n1255 = local write "Player2"(w1447) -> ()
                  n1256 = local write "Button 5"(w1447) -> ()
                  n1257 = local write "Button 4"(w1447) -> ()
                  n1258 = local write "Button 3"(w1447) -> ()
                  n1259 = local write "Button 2"(w1447) -> ()
                  n1260 = local write "Button 1"(w1447) -> ()
                }
              }
              n1261 = Build Array(w605, w734, w733, w732, w731, w730, w729, w728, w727, w726, w725, w724, w723, w722, w721, w720, w719, w718, w717, w716, w715, w714, w713, w712, w711, w710, w709, w708, w707, w706, w705, w704, w703, w702, w701, w700, w699, w698, w697, w696, w695, w694, w693, w692, w691, w690, w689, w678, w677, w676, w675, w688, w687, w686, w685, w684, w683, w682, w681, w680, w679, w631, w630, w629, w628, w627, w618, w617, w616, w615, w614, w613, w612, w611, w610, w619) -> (w599:u32[])
              n1262 = call "IMAQ Dispose"("Image"=w735) -> ()  [unwired: 5 in, 1 out]
              n1263 = Index Array(array=w601, index (col)=0 ("disabled index (col)")) -> (element=w743:i64[])  [unwired: 1 in]
              n1264 = Delete From Array(array=w599, index=0) -> (array with subset deleted=w659:u32[])  [unwired: 1 in, 1 out]
              n1265 = for {
                tunnel: w743 -> [w761] mode=indexing
                tunnel: w605 -> [w762]
                tunnel: [w761] -> w741 mode=indexing if=w763
                stop <- w763 continue-if-true
                n1266 = Less Or Equal?(x=w761, y=w762) -> (x <= y?=w763:bool)
              }
              n1267 = Delete From Array(array=w659, length=2, index=68) -> (array with subset deleted=w587:u32[])  [unwired: 1 out]
              n1268 = Array Size(array=w741) -> (size(s)=w600:i32)
              n1269 = Delete From Array(array=w587, length=17, index=43) -> (deleted portion=w653:u32[], array with subset deleted=w657:u32[])
              n1270 = Delete From Array(array=w587, length=2, index=0) -> (array with subset deleted=w584:u32[])  [unwired: 1 out]
              n1271 = Decrement(x=w600) -> (x-1=w651:i32)
              n1272 = Array Max & Min(array=w657) -> (max value=w658:u32)  [unwired: 3 out]
              n1273 = Array Max & Min(array=w653) -> (max value=w660:u32)  [unwired: 3 out]
              n1274 = Equal To 0?(x=w658) -> ()  [unwired: 1 out]
              n1275 = Not Equal To 0?(x=w660) -> (x != 0?=w656:bool)
              n1276 = Index Array(array=w601, index (row)=w651) -> (element=w654:i64[])  [unwired: 1 in]
              n1277 = Array Max & Min(array=w584) -> (max value=w737:u32)  [unwired: 3 out]
              n1278 = Compound Arithmetic op=AND(w646, w656, "Link Errors") -> (w602:bool)
              n1279 = Decrement(x=w600) -> (x-1=w647:i32)
              n1280 = Replace Array Subset(array=w654, new element=w653, index=44) -> (w598:i64[])
              n1281 = Equal To 0?(x=w737) -> (x = 0?=w590:bool)
              n1282 = Index Array(array=w598, index=w597) -> (element=w596:i64)
              n1283 = Replace Array Subset(array=w601, new element=w598, index (row)=w647) -> (w650:i64[][])  [unwired: 1 in]
              n1284 = Insert Into Array(array=w601, index (row)=w600, new element=w599) -> (w649:i64[][])  [unwired: 1 in]
              n1285 = Index Array(array=w599, index=w597) -> (element=w595:u32)
              n1286 = Select(t=w650, s=w602, f=w649) -> (s? t:f=w648:i64[][])
              n1287 = Select(t=w596, s=w602, f=w595) -> (s? t:f=w588:i64)
              n1288 = local read "last saved data"() -> (w593:i64[])
              n1289 = Select(t=w601, s=w590, f=w648) -> (s? t:f=w604:i64[][])
              n1290 = Search 1D Array(1D array=w593, element=w588) -> (index of element=w592:i32)  [unwired: 1 in]
              n1291 = Greater Than 0?(x=w592) -> (x > 0?=w591:bool)
              n1292 = Insert Into Array(array=w593, new element=w588) -> (w594:i64[])  [unwired: 1 in]
              n1293 = Or(x=w591, y=w590) -> (x .or. y?=w589:bool)
              n1294 = Select(t=w593, s=w589, f=w594) -> (s? t:f=w582:i64[])
              n1295 = case shown="True" "Undo" {
                tunnel: w604 -> [w745 w747]
                tunnel: [w745 w746] -> w603
                tunnel: w582 -> [w744 w756]
                tunnel: [w744 w749] -> w583
                frame False {
                }
                frame True {
                  n1296 = Reverse 1D Array(array=w756) -> (reversed array=w755:i64[])
                  n1297 = Delete From Array(array=w755, index=0) -> (deleted portion=w751:i64, array with subset deleted=w750:i64[])  [unwired: 1 in]
                  n1298 = Reverse 1D Array(array=w750) -> (reversed array=w749:i64[])
                  n1299 = Index Array(array=w747, index (col)=0 ("disabled index (col)")) -> (element=w752:i64[])  [unwired: 1 in]
                  n1300 = Search 1D Array(1D array=w752, element=w751) -> (index of element=w748:i32)  [unwired: 1 in]
                  n1301 = local write "Undo"(FALSE ("Undo")) -> ()
                  n1302 = Delete From Array(array=w747, index (row)=w748) -> (array with subset deleted=w746:i64[][])  [unwired: 2 in, 1 out]
                }
              }
              "last saved data" <- w583
              n1303 = Concatenate Strings("Btn 1", w607, "Btn 2", w607, "Btn 3", w607, "Btn 4", w607, "Btn 5", w607, "Error" ("String")) -> (w621:string)
              n1304 = for {
                tunnel: string[] ["frame number", "Lead", "Lag", "position 1", "position 2", "position 3", "position 4", "position 5", "position 6", "position 7", "position 8", "position 9", "position 10", "position 11", "position 12", "position 13", "position 14", "position 15", "position 16", "position 17", "position 18", "position 19", "position 20", "position 21", "position 22", "position 23", "position 24", "Drive A", "Drive D", "SW Drive A", "SW Drive D", "drop", "chop", "lob", "boast 2", "boast 3", "smash", "Forehand", "Backhand", "Straight", "Cross", "Bounce", "Half Volley", "Volley", "Expected winner 1", "Expected winner 2", "Unexpected winner 1", "Unexpected winner 2", "Stroke 1", "Stroke 2", "Forced error 1", "Forced error 2", "Unforced error 1", "Unforced error 2", "No let 1", "No let 2", "Let", "point1", "point2", "score1", "score2", "service1", "service2", "s1", "s2", "s3", "s4", "s5", "s6", "player1", "player2"] ("all rows") -> [w760] mode=indexing
                tunnel: [w758] -> w608 mode=indexing
                n1305 = Concatenate Strings(w760, "\t") -> (w758:string)
              }
              n1306 = Index Array(array=w603, index (col)=0 ("disabled index (col)")) -> (element=w672:i64[])  [unwired: 1 in]
              n1307 = local read "Video file"() -> (w640:path)
              n1308 = Index Array(array=w603, index (col) #1=57 ("disabled index (col)"), index (col) #2=58 ("index (col)")) -> (element #1=w668:i64[], element #2=w665:i64[])  [unwired: 2 in]
              n1309 = local read "Data file"() -> (w634:path)
              n1310 = Array Max & Min(array=w672) -> (max index (indices)=w673:i32)  [unwired: 3 out]
              n1311 = Add Array Elements(numeric array=w668) -> (sum=→"P1":i64)
              n1312 = Add Array Elements(numeric array=w665) -> (sum=→"P2":i64)
              n1313 = call <vilib>:"Get File Extension.vi"("file"=w640) -> ("filename without extension"=w642:string)  [unwired: 7 in, 3 out]
              n1314 = Open/Create/Replace File(file path (use dialog)=w634, operation (0:open)=T3."replace") -> (refnum out=w636:refnum<file>, error out=w635:errorcluster)  [unwired: 4 in, 1 out]
              n1315 = Index Array(array=w603, index (row)=w673) -> (element=→"last row":i64[])  [unwired: 1 in]
              n1316 = Concatenate Strings(w608, w621, "\r") -> (w633:string)
              n1317 = Array To Spreadsheet String(delimiter (Tab)="\t" ("delimiter (\\t)"), array=w603, 3:"%.3f" ("format (%.3f)")) -> (spreadsheet string=w645:string)
              n1318 = Concatenate Strings("avi file" ("string"), w643, w642, w643, w643, w633, w645) -> (w644:string)
              n1319 = Write to Text File(file (use dialog)=w636, text=w644, error in=w635) -> (refnum out=w632:refnum<file>)  [unwired: 1 in, 2 out]
            }
          }
          "coding" <- w576
        }
        frame "Display" {
          n1320 = flat-sequence {
            tunnel: [w1520] -> w1485
            tunnel: w1482 -> [w1521]
            tunnel: w1485 -> [w1528]
            tunnel: [w1527] -> w1481
            tunnel: [w1526] -> w1479
            tunnel: [w1525] -> w1478
            tunnel: w1481 -> [w1587]
            tunnel: [w1587] -> w1480
            tunnel: w1479 -> [w1585]
            tunnel: w1478 -> [w1586]
            tunnel: [w1586] -> w1477
            tunnel: [w1585] -> w1476
            tunnel: [w1629] -> w1484
            tunnel: w1480 -> [w1630]
            tunnel: w1477 -> [w1629]
            tunnel: w1476 -> [w1628]
            tunnel: [w1628] -> w1475
            tunnel: [w1628] -> w1474
            tunnel: w1484 -> [w1690]
            tunnel: [w1690] -> w1483
            tunnel: w1475 -> [_]
            tunnel: w1474 -> [w1679]
            tunnel: [w1679] -> w1473
            tunnel: w1483 -> [w1703]
            tunnel: w1473 -> [w1700]
            frame #0 {
              n1321 = case shown="\"2\"" "display\nselection" {
                tunnel: [w1523 w1524] -> w1520
                tunnel: w1521 -> [w1523 _]
                frame "1", Default {
                }
                frame "2" {
                  n1322 = local read "Edited data"() -> (w1524:i64[][])
                }
              }
            }
            frame #1 {
              w1537 = 64
              # "disreagard player on display option to be set here"
              # "ADD elements on one column to get the data"
              # "extract seperate data sets for player 1 and player 2"
              n1323 = Index Array(array=w1528, index (col)=69 ("index")) -> (element=w1530:i64[])  [unwired: 1 in]
              n1324 = Index Array(array=w1528, index (col)=70 ("index")) -> (element=w1533:i64[])  [unwired: 1 in]
              n1325 = for {
                tunnel: w1528 -> [w1566]
                tunnel: w1530 -> [w1568] mode=indexing
                shift-right: [w1561] -> w1535
                shift-left: i64[][] [] ("Combined data") -> [w1562]
                i -> [w1565]
                n1326 = Index Array(array=w1566, index (row)=w1565) -> (element=w1564:i64[])  [unwired: 1 in]
                n1327 = Not Equal To 0?(x=w1568) -> (x != 0?=w1567:bool)
                n1328 = Insert Into Array(array=w1562, new element=w1564) -> (w1563:i64[][])  [unwired: 2 in]
                n1329 = Select(t=w1563, s=w1567, f=w1562) -> (s? t:f=w1561:i64[][])
              }
              n1330 = for {
                tunnel: w1528 -> [w1558]
                tunnel: w1533 -> [w1560] mode=indexing
                shift-right: [w1553] -> w1536
                shift-left: i64[][] [] ("Combined data") -> [w1554]
                i -> [w1557]
                n1331 = Index Array(array=w1558, index (row)=w1557) -> (element=w1556:i64[])  [unwired: 1 in]
                n1332 = Not Equal To 0?(x=w1560) -> (x != 0?=w1559:bool)
                n1333 = Insert Into Array(array=w1554, new element=w1556) -> (w1555:i64[][])  [unwired: 2 in]
                n1334 = Select(t=w1555, s=w1559, f=w1554) -> (s? t:f=w1553:i64[][])
              }
              n1335 = for {
                N: w1537 -> [_]
                tunnel: w1536 -> [w1546]
                tunnel: [w1543] -> w1526 mode=indexing
                i -> [w1547]
                n1336 = Increment(x=w1547) -> (x+1=w1545:i32)
                n1337 = Index Array(array=w1546, index (col)=w1545) -> (element=w1544:i64[])  [unwired: 1 in]
                n1338 = Add Array Elements(numeric array=w1544) -> (sum=w1543:i64)
              }
              "Player 2 data" <- w1526
              n1339 = for {
                N: w1537 -> [_]
                tunnel: w1535 -> [w1551]
                tunnel: [w1548] -> w1525 mode=indexing
                i -> [w1552]
                n1340 = Increment(x=w1552) -> (x+1=w1550:i32)
                n1341 = Index Array(array=w1551, index (col)=w1550) -> (element=w1549:i64[])  [unwired: 1 in]
                n1342 = Add Array Elements(numeric array=w1549) -> (sum=w1548:i64)
              }
              "player 1 data" <- w1525
              n1343 = for {
                N: w1537 -> [_]
                tunnel: w1528 -> [w1541]
                tunnel: [w1538] -> w1527 mode=indexing
                i -> [w1542]
                n1344 = Increment(x=w1542) -> (x+1=w1540:i32)
                n1345 = Index Array(array=w1541, index (col)=w1540) -> (element=w1539:i64[])  [unwired: 1 in]
                n1346 = Add Array Elements(numeric array=w1539) -> (sum=w1538:i64)
              }
              "both player data" <- w1527
            }
            frame #2 {
              # "Position numbers"
              n1347 = Array Subset(array=w1586, index=2, length=26) -> (w1623:i64[])
              n1348 = Index Array(array=w1623) -> (element #1=→"1 13":i64, element #2=→"1 14":i64, element #3=→"1 11":i64, element #4=→"1 9":i64, element #5=→"2 14":i64, element #6=→"2 13":i64, element #7=→"2 11":i64, element #8=→"2 9":i64, element #9=→"3 13":i64, element #10=→"3 11":i64, element #11=→"3 10":i64, element #12=→"3 8":i64, element #13=→"4 13":i64, element #14=→"4 11":i64, element #15=→"4 10":i64, element #16=→"4 8":i64, element #17=→"5 17":i64, element #18=→"5 16":i64, element #19=→"5 15":i64, element #20=→"5 18":i64, element #21=→"6 21":i64, element #22=→"6 20":i64, element #23=→"6 19":i64, element #24=→"6 18":i64)  [unwired: 24 in]
              n1349 = Array Subset(array=w1585, index=2, length=26) -> (w1606:i64[])
              n1350 = Index Array(array=w1606) -> (element #1=→"1 12":i64, element #2=→"1 22":i64, element #3=→"1 32":i64, element #4=→"1 42":i64, element #5=→"2 12":i64, element #6=→"2 22":i64, element #7=→"2 32":i64, element #8=→"2 42":i64, element #9=→"3 12":i64, element #10=→"3 22":i64, element #11=→"3 32":i64, element #12=→"3 42":i64, element #13=→"4 12":i64, element #14=→"4 22":i64, element #15=→"4 32":i64, element #16=→"4 42":i64, element #17=→"5 14":i64, element #18=→"5 23":i64, element #19=→"5 33":i64, element #20=→"5 43":i64, element #21=→"6 15":i64, element #22=→"6 24":i64, element #23=→"6 34":i64, element #24=→"6 44":i64)  [unwired: 24 in]
            }
            frame #3 {
              # "winner error numbers"
              # "Shot numbers"
              n1351 = Array Subset(array=w1628, index=26, length=10) -> (w1647:i64[])
              n1352 = Index Array(array=w1628, index=55) -> (element=w1637:i64)
              n1353 = Index Array(array=w1629, index=55) -> (element=w1634:i64)
              n1354 = Array Subset(array=w1629, index=26, length=10) -> (w1648:i64[])
              n1355 = Number To Fractional String(number=w1647, precision (6)=i16 0) -> (F-format string=w1662:string[])  [unwired: 2 in]
              n1356 = Array Subset(array=w1630, index=43, length=12) -> (w1654:i64[])
              n1357 = Number To Fractional String(number=w1637, precision (6)=i16 0) -> (F-format string=→"Let 4":string)  [unwired: 2 in]
              n1358 = Number To Fractional String(number=w1648, precision (6)=i16 0) -> (F-format string=w1663:string[])  [unwired: 2 in]
              n1359 = Number To Fractional String(number=w1634, precision (6)=i16 0) -> (F-format string=→"Let 3":string)  [unwired: 2 in]
              n1360 = Insert Into Array(array=w1662, index=4, new element="" ("new element/subarray")) -> (→"Player 2 shots numbers":string[])
              n1361 = Number To Fractional String(number=w1654, precision (6)=i16 0) -> (F-format string=w1653:string[])  [unwired: 2 in]
              n1362 = Insert Into Array(array=w1663, index=4, new element="" ("new element/subarray")) -> (→"Player 1 shots numbers":string[])
              n1363 = Index Array(array=w1653) -> (element #1=→"ex win1 num":string, element #2=→"ex win2 num":string, element #3=→"UNex win1 num":string, element #4=→"UNex win2 num":string, element #5=→"Stroke 3":string, element #6=→"Stroke 4":string, element #7=→"F err1 num":string, element #8=→"F err2 num":string, element #9=→"UF err1 num":string, element #10=→"UF err2 num":string, element #11=→"No Let 1":string, element #12=→"No Let 2":string)  [unwired: 12 in]
            }
            frame #4 {
              n1364 = Array Subset(array=w1690, index=36, length=7) -> (w1692:i64[])
              n1365 = Array Subset(array=w1679, index=36, length=7) -> (w1683:i64[])
              n1366 = Number To Fractional String(number=w1692, precision (6)=i16 0) -> (F-format string=w1691:string[])  [unwired: 2 in]
              n1367 = Number To Fractional String(number=w1683, precision (6)=i16 0) -> (F-format string=w1684:string[])  [unwired: 2 in]
              n1368 = Index Array(array=w1691) -> (element #1=→"F-hand 1":string, element #2=→"B-hand 1":string, element #3=→"Straight 1":string, element #4=→"Cross 1":string, element #5=→"Bounce 1":string, element #6=→"H-volley 1":string, element #7=→"Volley 1":string)  [unwired: 7 in]
              n1369 = Index Array(array=w1684) -> (element #1=→"F-hand 2":string, element #2=→"B-hand 2":string, element #3=→"Straight 3":string, element #4=→"Cross 3":string, element #5=→"Bounce 3":string, element #6=→"H-volley 3":string, element #7=→"Volley 3":string)  [unwired: 7 in]
            }
            frame #5 {
              # "slider sclaes for graphical display"
              n1370 = Array Subset(array=w1703, index=26, length=10) -> (w1699:i64[])
              "subarray" <- w1699
              n1371 = Array Subset(array=w1700, index=26, length=10) -> (w1698:i64[])
              n1372 = Insert Into Array(array=w1699, new element=w1698) -> (w1697:i64[])  [unwired: 1 in]
              n1373 = Array Max & Min(array=w1698) -> (max value=w1707:i64)  [unwired: 3 out]
              n1374 = Equal To 0?(x=w1707) -> (x = 0?=w1706:bool)
              n1375 = Array Max & Min(array=w1697) -> (max value=w1711:i64)  [unwired: 3 out]
              n1376 = Select(t=1.0, s=w1706, f=w1707) -> ()  [unwired: 1 out]
              n1377 = Equal To 0?(x=w1711) -> (x = 0?=w1710:bool)
              n1378 = Select(t=1.0, s=w1710, f=w1711) -> (s? t:f=w1696:dbl)
              n1379 = property on="FH 2" class="Slide (strict)"("Scale.Maximum"=w1696) -> ()  [unwired: 2 in, 2 out]
              n1380 = property on="BH 2" class="Slide (strict)"("Scale.Maximum"=w1696) -> ()  [unwired: 2 in, 2 out]
              n1381 = property on="Straight 2" class="Slide (strict)"("Scale.Maximum"=w1696) -> ()  [unwired: 2 in, 2 out]
              n1382 = property on="Cross 2" class="Slide (strict)"("Scale.Maximum"=w1696) -> ()  [unwired: 2 in, 2 out]
              n1383 = property on="Bounce 2" class="Slide (strict)"("Scale.Maximum"=w1696) -> ()  [unwired: 2 in, 2 out]
              n1384 = property on="Volley 2" class="Slide (strict)"("Scale.Maximum"=w1696) -> ()  [unwired: 2 in, 2 out]
              n1385 = property on="Drive 2" class="Slide (strict)"("Scale.Maximum"=w1696) -> ()  [unwired: 2 in, 2 out]
              n1386 = property on="Drop 13" class="Slide (strict)"("Scale.Maximum"=w1696) -> ()  [unwired: 2 in, 2 out]
              n1387 = property on="Lob 2" class="Slide (strict)"("Scale.Maximum"=w1696) -> ()  [unwired: 2 in, 2 out]
              n1388 = property on="Boast 13" class="Slide (strict)"("Scale.Maximum"=w1696) -> ()  [unwired: 2 in, 2 out]
              n1389 = property on="Drive 1" class="Slide (strict)"("Scale.Maximum"=w1696) -> ()  [unwired: 2 in, 2 out]
              n1390 = property on="Drop 1" class="Slide (strict)"("Scale.Maximum"=w1696) -> ()  [unwired: 2 in, 2 out]
              n1391 = property on="Lob 1" class="Slide (strict)"("Scale.Maximum"=w1696) -> ()  [unwired: 2 in, 2 out]
              n1392 = property on="Boast 1" class="Slide (strict)"("Scale.Maximum"=w1696) -> ()  [unwired: 2 in, 2 out]
              n1393 = property on="FH 1" class="Slide (strict)"("Scale.Maximum"=w1696) -> ()  [unwired: 2 in, 2 out]
              n1394 = property on="BH 1" class="Slide (strict)"("Scale.Maximum"=w1696) -> ()  [unwired: 2 in, 2 out]
              n1395 = property on="Straight 4" class="Slide (strict)"("Scale.Maximum"=w1696) -> ()  [unwired: 2 in, 2 out]
              n1396 = property on="Cross 4" class="Slide (strict)"("Scale.Maximum"=w1696) -> ()  [unwired: 2 in, 2 out]
              n1397 = property on="Bounce 4" class="Slide (strict)"("Scale.Maximum"=w1696) -> ()  [unwired: 2 in, 2 out]
              n1398 = property on="Volley 4" class="Slide (strict)"("Scale.Maximum"=w1696) -> ()  [unwired: 2 in, 2 out]
              n1399 = Index Array(array=w1698) -> (element #1=→"Drive 2":i64, element #2=→"Drop 13":i64, element #3=→"Lob 2":i64, element #4=→"Boast 13":i64, element #5=→"FH 2":i64, element #6=→"BH 2":i64, element #7=→"Straight 2":i64, element #8=→"Cross 2":i64, element #9=→"Bounce 2":i64, element #10=→"Volley 2":i64)  [unwired: 10 in]
              n1400 = Index Array(array=w1699) -> (element #1=→"Drive 1":i64, element #2=→"Drop 1":i64, element #3=→"Lob 1":i64, element #4=→"Boast 1":i64, element #5=→"FH 1":i64, element #6=→"BH 1":i64, element #7=→"Straight 4":i64, element #8=→"Cross 4":i64, element #9=→"Bounce 4":i64, element #10=→"Volley 4":i64)  [unwired: 10 in]
            }
          }
          n1401 = local read "Video files to write"() -> (w1469:string[])
          n1402 = property on="Video files to write" class="Arr (strict)"() -> ("Index Values"=w1468:u32[])  [unwired: 2 in, 2 out]
          n1403 = local read "frames to write"() -> (w1470:i64[][])
          n1404 = case shown="True" "Upload edited video" {
            frame False {
            }
            frame True {
              n1405 = flat-sequence {
                frame #0 {
                  n1406 = local read "frames edited"() -> (w1516:i64[])
                  n1407 = local write "Progress..."(u32 0 ("Progress...")) -> ()
                  n1408 = local write "frames 2 play"(w1516) -> ()
                }
                frame #1 {
                  w1518 = FALSE ("stop")
                  w1519 = TRUE ("Play")
                  n1409 = local write "Load video"(w1519) -> ()
                  n1410 = local write "Play"(w1519) -> ()
                  n1411 = local write "stop"(w1518) -> ()
                  n1412 = local write "Upload edited video"(w1518) -> ()
                  n1413 = local write "Pause"(w1518) -> ()
                }
              }
            }
          }
          n1414 = Index Array(array=w1468) -> (element=w1465:u32)  [unwired: 1 in]
          n1415 = And Array Elements(Boolean array="Delete") -> (logical AND=w1467:bool)
          n1416 = case shown="True" "Add to lib" {
            tunnel: w1470 -> [_ w1511]
            tunnel: w1469 -> [_ w1508]
            frame False {
            }
            frame True {
              n1417 = local read "frames edited"() -> (w1507:i64[])
              n1418 = local write "Add to lib"(FALSE ("Add to lib")) -> ()
              n1419 = Build Array("File name") -> (w1509:string[])
              n1420 = Build Array(w1507) -> (w1512:i64[][])
              n1421 = Insert Into Array(array=w1512, new element=w1511) -> (→"frames to write":i64[][])  [unwired: 2 in]
              n1422 = Insert Into Array(array=w1509, new element=w1508) -> (→"Video files to write":string[])  [unwired: 1 in]
            }
          }
          n1423 = case shown="False" w1467 {
            tunnel: "Delete" -> [w1503 _]
            tunnel: w1465 -> [w1501 _]
            frame False {
              n1424 = for {
                tunnel: w1503 -> [w1506] mode=indexing
                tunnel: [w1504] -> w1502
                i -> [w1504]
                stop <- w1505 stop-if-true
                n1425 = Not(x=w1506) -> (.not. x?=w1505:bool)
              }
              n1426 = local write "Delete"(bool[] [TRUE, TRUE, TRUE, TRUE, TRUE] ("Array 2")) -> ()
              n1427 = local read "Video files to write"() -> (w1498:string[])
              n1428 = local read "frames to write"() -> (w1496:i64[][])
              n1429 = Add(x=w1502, y=w1501) -> (x+y=w1495:u32)
              n1430 = Delete From Array(array=w1498, index=w1495) -> (array with subset deleted=w1500:string[])  [unwired: 1 in, 1 out]
              n1431 = Delete From Array(array=w1496, index (row)=w1495) -> (array with subset deleted=w1497:i64[][])  [unwired: 2 in, 1 out]
              n1432 = local write "frames to write"(w1497) -> ()
              n1433 = local write "Video files to write"(w1500) -> ()
            }
            frame True {
            }
          }
          n1434 = local read "refnum of data save file"() -> (w1487:refnum<file>)
          n1435 = local write "Code number display"(1 ("Code number")) -> ()
          n1436 = Select(t=T1."Edit video" ("Main tab"), s="Extract data", f=T1."Display" ("Main tab")) -> (s? t:f=w1493:T1)
          n1437 = Select(t=T1."Examine coding" ("Main tab"), s="Examine code", f=w1493) -> (s? t:f=w1494:T1)
        }
        frame "Edit video" {
          w1753 = T4."Disabled and Grayed Out" ("Disabled")
          n1438 = local read "Btn 5"() -> (w1736:string)
          "Btn 10" <- w1736
          n1439 = local read "Btn 4"() -> (w1735:string)
          "Btn 9" <- w1735
          n1440 = local read "Btn 3"() -> (w1734:string)
          "Btn 8" <- w1734
          n1441 = local read "Btn 2"() -> (w1733:string)
          "Btn 7" <- w1733
          n1442 = local read "Btn 1"() -> (w1732:string)
          "Btn 6" <- w1732
          n1443 = property on="Button 10" class="Bool (strict)"("BoolText.Text"=w1736) -> ()  [unwired: 2 in, 2 out]
          n1444 = property on="Button 9" class="Bool (strict)"("BoolText.Text"=w1735) -> ()  [unwired: 2 in, 2 out]
          n1445 = property on="Button 8" class="Bool (strict)"("BoolText.Text"=w1734) -> ()  [unwired: 2 in, 2 out]
          n1446 = property on="Button 7" class="Bool (strict)"("BoolText.Text"=w1733) -> ()  [unwired: 2 in, 2 out]
          n1447 = property on="Button 6" class="Bool (strict)"("BoolText.Text"=w1732) -> ()  [unwired: 2 in, 2 out]
          n1448 = Array Size(array=w1740) -> (size(s)=w1741:i32[])
          n1449 = Index Array(array=w1741) -> (element #2=w1739:i32)  [unwired: 2 in, 1 out]
          n1450 = Initialize Array(i64 0 ("element"), w1739) -> (w1738:i64[])
          n1451 = local write "Extract data"(FALSE ("edit video")) -> ()
          n1452 = Build Array(w1738) -> (w1737:i64[][])
          n1453 = property on="Code number display" class="DigNum (strict)"("DisabledEnum"=w1753) -> ()  [unwired: 2 in, 2 out]
          n1454 = property on="Next" class="Bool (strict)"("DisabledEnum"=w1753) -> ()  [unwired: 2 in, 2 out]
          n1455 = property on="Reset" class="Bool (strict)"("DisabledEnum"=w1753) -> ()  [unwired: 2 in, 2 out]
          n1456 = property on="Update" class="Bool (strict)"("DisabledEnum"=w1753) -> ()  [unwired: 2 in, 2 out]
          n1457 = property on="Previous" class="Bool (strict)"("DisabledEnum"=w1753) -> ()  [unwired: 2 in, 2 out]
          n1458 = flat-sequence {
            tunnel: [w1772] -> w1743
            tunnel: [w1771] -> w1744
            tunnel: [w1770] -> w1745
            tunnel: [w1769] -> w1746
            tunnel: [w1768] -> w1747
            tunnel: [w1767] -> w1748
            tunnel: [w1766] -> w1749
            tunnel: [w1765] -> w1750
            tunnel: [w1764] -> w1751
            tunnel: [w1760] -> w1752
            tunnel: w1740 -> [w1758]
            tunnel: w1737 -> [w1757]
            tunnel: w1752 -> [w1848]
            tunnel: w1751 -> [w1849]
            tunnel: w1750 -> [w1850]
            tunnel: w1749 -> [w1858]
            tunnel: w1748 -> [w1859]
            tunnel: w1747 -> [w1868]
            tunnel: w1746 -> [w1869]
            tunnel: w1745 -> [w1870]
            tunnel: w1744 -> [w1878]
            tunnel: w1743 -> [w1902]
            frame #0 {
              # "seperate sections of data"
              n1459 = Insert Into Array(array=w1757, new element=w1758) -> (w1759:i64[][])  [unwired: 2 in]
              "Combined data" <- w1759
              n1460 = Array Size(array=w1759) -> (size(s)=w1763:i32[])
              n1461 = Index Array(array=w1763) -> (element=w1762:i32)  [unwired: 1 in]
              n1462 = Initialize Array(i64 0 ("element"), w1762) -> (w1760:i64[])
              n1463 = Array Subset(array=w1759, index (col)=3 ("index"), length (col)=24 ("length")) -> (w1772:i64[][])  [unwired: 2 in]
              n1464 = Array Subset(array=w1759, index (col)=27 ("index"), length (col)=10 ("length")) -> (w1771:i64[][])  [unwired: 2 in]
              n1465 = Array Subset(array=w1759, index (col)=37 ("index"), length (col)=2 ("length")) -> (w1770:i64[][])  [unwired: 2 in]
              n1466 = Array Subset(array=w1759, index (col)=39 ("index"), length (col)=2 ("length")) -> (w1769:i64[][])  [unwired: 2 in]
              n1467 = Array Subset(array=w1759, index (col)=41 ("index"), length (col)=3 ("length")) -> (w1768:i64[][])  [unwired: 2 in]
              n1468 = Array Subset(array=w1759, index (col)=44 ("index"), length (col)=13 ("length")) -> (w1767:i64[][])  [unwired: 2 in]
              n1469 = Array Subset(array=w1759, index (col)=61 ("index"), length (col)=8 ("length")) -> (w1766:i64[][])  [unwired: 2 in]
              n1470 = Array Subset(array=w1759, index (col)=69 ("index"), length (col)=2 ("length")) -> (w1765:i64[][])  [unwired: 2 in]
              n1471 = Array Subset(array=w1759, index (col)=71 ("index"), length (col)=5 ("length")) -> (w1764:i64[][])  [unwired: 2 in]
            }
            frame #1 {
              w1932 = i64[][] [] ("Combined data")
              # "AND different sections of data"
              # "needs data to display for\n\nfull match (combined data)\nedited section\n1 shot b4\n1shot after"
              # "display which data selector needs to be set here"
              # "extract select events ONLY from full data"
              # "delete negative frames\nand frames past last frame of video"
              # "delete repeated frames"
              n1472 = Build Array("Adrive", "Ddrive", "ASWdrive", "DSWdrive", "Drop 14", "Chop 13", "Lob", "Boast2", "Boast3", "Smash 13") -> (w1828:bool[])
              n1473 = Build Array("1 10", "1 7", "1 6", "1 5", "2 10", "2 7", "2 6", "2 5", "3 9", "3 7", "3 6", "3 5", "4 9", "4 7", "4 6", "4 5", "5 8", "5 7", "5 6", "5 5", "6 8", "6 7", "6 6", "6 5") -> (w1829:bool[])
              n1474 = call "or multiple inputs.vi"("zero array in"=w1848, "input array in"=w1828, "file data in"=w1878) -> ("array out"=w1845:dbl[], "no input?"=w1830:bool)
              n1475 = call "or multiple inputs.vi"("zero array in"=w1848, "input array in"=w1829, "file data in"=w1902) -> ("array out"=w1843:dbl[], "no input?"=w1832:bool)
              n1476 = Build Array("Expected Winner1 2", "Expected Winner2 2", "Unexpected Winner1 2", "Unexpected Winner2 2", "Stroke1 2", "Stroke2 2", "Forced Error1 2", "Forced Error2 2", "Unforced Error1 2", "Unforced Error2 2", "Nolet1 2", "Nolet2 2", "Let 2") -> (w1824:bool[])
              n1477 = call "or multiple inputs.vi"("zero array in"=w1848, "input array in"=w1824, "file data in"=w1859) -> ("array out"=w1844:dbl[], "no input?"=w1831:bool)
              n1478 = Build Array("FH", "BH") -> (w1827:bool[])
              n1479 = Build Array("ST", "CR") -> (w1826:bool[])
              n1480 = Build Array("Bounce", "Half Volley", "Volley") -> (w1825:bool[])
              n1481 = Build Array("Player1 2", "Player2 2") -> (w1822:bool[])
              n1482 = Build Array("Button 6", "Button 7", "Button 8", "Button 9", "Button 10") -> (w1821:bool[])
              n1483 = Build Array("Service1 2", "Service2 2", "S1 2", "S2 2", "S3 2", "S4 2", "S5 2", "S6 2") -> (w1823:bool[])
              n1484 = call "or multiple inputs.vi"("zero array in"=w1848, "input array in"=w1827, "file data in"=w1870) -> ("array out"=w1847:dbl[], "no input?"=w1838:bool)
              n1485 = call "or multiple inputs.vi"("zero array in"=w1848, "input array in"=w1826, "file data in"=w1869) -> ("array out"=w1846:dbl[], "no input?"=w1837:bool)
              n1486 = call "or multiple inputs.vi"("zero array in"=w1848, "input array in"=w1825, "file data in"=w1868) -> ("array out"=w1839:dbl[], "no input?"=w1836:bool)
              n1487 = call "or multiple inputs.vi"("zero array in"=w1848, "input array in"=w1822, "file data in"=w1850) -> ("array out"=w1840:dbl[], "no input?"=w1835:bool)
              n1488 = call "or multiple inputs.vi"("zero array in"=w1848, "input array in"=w1821, "file data in"=w1849) -> ("array out"=w1841:dbl[], "no input?"=w1834:bool)
              n1489 = call "or multiple inputs.vi"("zero array in"=w1848, "input array in"=w1823, "file data in"=w1858) -> ("array out"=w1842:dbl[], "no input?"=w1833:bool)
              n1490 = Compound Arithmetic op=AND(w1847, w1846, w1839, w1840, w1841, w1842, w1843, w1844, w1845) -> (w1921:i32[])
              "result" <- w1921
              n1491 = Compound Arithmetic op=AND(w1838, w1837, w1836, w1835, w1834, w1833, w1832, w1831, w1830) -> (w1919:bool)
              n1492 = Select(t=i32[] [] ("result"), s=w1919, f=w1921) -> (s? t:f=w1934:i32[])
              "EVENTS\nTO PLAY" <- w1934
              n1493 = local read "Combined data"() -> (w1812:i64[][])
              n1494 = Insert Into Array(array=w1829, new element #1=w1828, new element #2=w1827, new element #3=w1826, new element #4=w1825, new element #5=w1824, new element #6=w1823, new element #7=w1822, new element #8=w1821) -> (w1820:bool[])  [unwired: 1 in]
              "Last Edit" <- w1820
              n1495 = for {
                tunnel: w1812 -> [w1963]
                tunnel: w1934 -> [w1972] mode=indexing
                shift-right: [w1973] -> w1931
                shift-left: w1932 -> [w1974]
                shift-right: [w1967] -> w1930
                shift-left: w1932 -> [w1968]
                shift-right: [w1960] -> w1929
                shift-left: w1932 -> [w1961]
                i -> [w1965]
                n1496 = Increment(x=w1965) -> (x+1=w1964:i32)
                n1497 = Decrement(x=w1965) -> (x-1=w1971:i32)
                n1498 = Index Array(array=w1963, index (row)=w1965) -> (element=w1976:i64[])  [unwired: 1 in]
                n1499 = Index Array(array=w1963, index (row)=w1964) -> (element=w1966:i64[])  [unwired: 1 in]
                n1500 = Not Equal To 0?(x=w1972) -> (x != 0?=w1959:bool)
                n1501 = Index Array(array=w1963, index (row)=w1971) -> (element=w1970:i64[])  [unwired: 1 in]
                n1502 = Insert Into Array(array=w1961, new element=w1966) -> (w1962:i64[][])  [unwired: 2 in]
                n1503 = Insert Into Array(array=w1974, new element=w1976) -> (w1975:i64[][])  [unwired: 2 in]
                n1504 = Insert Into Array(array=w1968, new element=w1970) -> (w1969:i64[][])  [unwired: 2 in]
                n1505 = Select(t=w1969, s=w1959, f=w1968) -> (s? t:f=w1967:i64[][])
                n1506 = Select(t=w1962, s=w1959, f=w1961) -> (s? t:f=w1960:i64[][])
                n1507 = Select(t=w1975, s=w1959, f=w1974) -> (s? t:f=w1973:i64[][])
              }
              "Edited data" <- w1931
              "Event After" <- w1929
              "Event before" <- w1930
              n1508 = Or Array Elements(Boolean array=w1820) -> (logical OR=w1811:bool)
              n1509 = Index Array(array=w1931, index (col) #1=0 ("disabled index (col)"), index (col) #2=1 ("disabled index (row)"), index (col) #3=2 ("disabled index (col)")) -> (element #1=w1940:i64[], element #2=w1796:i64[], element #3=w1795:i64[])  [unwired: 3 in]
              n1510 = Build Array(w1940) -> (w1928:i64[][])
              n1511 = Empty Array?(array=w1940) -> (empty?=w1818:bool)
              n1512 = Array Size(array=w1940) -> (size(s)=w1941:i32)
              n1513 = local read "framesPerSecond"() -> (w1794:u32)
              n1514 = Transpose 2D Array(2D array=w1928) -> (transposed array=→"edited\nevents":i64[][])
              n1515 = property on="Code number display" class="DigNum (strict)"("Maximum"=w1941, "Minimum"=1.0 ("Data Entry Limits:Minimum")) -> ()  [unwired: 2 in, 2 out]
              n1516 = And(x=w1818, y=w1811) -> (x .and. y?=w1819:bool)
              n1517 = case shown="True" w1819 {
                frame False {
                  n1518 = for {
                    N: 300 -> [_]
                    i -> [w2008]
                    n1519 = Increment(x=w2008) -> (x+1=w2007:i32)
                    n1520 = local write "task"(w2007) -> ()
                    n1521 = Wait (ms)(milliseconds to wait=u32 1) -> ()  [unwired: 1 out]
                  }
                }
                frame True {
                  n1522 = One Button Dialog(message="INVALID EVENTS\n\nSelected event(s) or combination of events does not exist") -> ()  [unwired: 1 in, 1 out]
                }
              }
              n1523 = for {
                tunnel: "after" -> [w1979]
                tunnel: w1940 -> [w1998] mode=indexing
                shift-right: [w1992] -> w1810
                shift-left: u32[] [] -> [w1994]
                tunnel: w1796 -> [w1982] mode=indexing
                tunnel: [w1978] -> _ mode=indexing
                tunnel: w1795 -> [w1978] mode=indexing
                tunnel: w1794 -> [w1984]
                tunnel: "before" -> [w1983]
                tunnel: "playback interval on" -> [w1977]
                n1524 = Select(t=w1983, s=w1977, f=w1982) -> (s? t:f=w1981:i64)
                n1525 = Select(t=w1979, s=w1977, f=w1978) -> (s? t:f=w1980:i64)
                n1526 = Multiply(x=w1984, y=w1981) -> (x*y=w1986:i64)
                n1527 = Multiply(x=w1984, y=w1980) -> (x*y=w1985:i64)
                n1528 = Array Max & Min(array=w1994) -> (max value=w1997:u32, max index (indices)=w1993:i32)  [unwired: 2 out]
                n1529 = Subtract(x=w1998, y=w1986) -> (x-y=w1996:i64)
                n1530 = Add(x=w1985, y=w1998) -> (x+y=w1995:i64)
                n1531 = Greater Or Equal?(x=w1997, y=w1996) -> (x >= y?=w1989:bool)
                n1532 = Build Array(w1996, w1995) -> (w1987:i64[])
                n1533 = Build Array(w1995) -> (w1991:i64[])
                n1534 = And(x="Combine", y=w1989) -> (x .and. y?=w1990:bool)
                n1535 = case shown="True" w1990 {
                  tunnel: w1994 -> [w2001 w2005]
                  tunnel: w1993 -> [_ w2004]
                  tunnel: w1991 -> [_ w2003]
                  tunnel: [w2000 w2002] -> w1992
                  tunnel: w1987 -> [w1999 _]
                  frame False {
                    n1536 = Insert Into Array(array=w2001, new element=w1999) -> (w2000:u32[])  [unwired: 1 in]
                  }
                  frame True {
                    n1537 = Replace Array Subset(array=w2005, new element=w2003, index=w2004) -> (w2002:u32[])
                  }
                }
              }
              n1538 = Delete From Array(array=w1812, length=1, index (col)=0 ("disabled index (col)")) -> (deleted portion=w1817:i64[][])  [unwired: 1 in, 1 out]
              n1539 = Array Max & Min(array=w1817) -> (max value=w1816:i64, min value=w1815:i64)  [unwired: 2 out]
              n1540 = Build Array(w1815, w1816) -> (w1808:i64[])
              n1541 = Select(t=w1810, s=w1811, f=w1808) -> (s? t:f=w1809:i64[])
              "edited to play" <- w1809
              n1542 = Array Size(array=w1809) -> (size(s)=w1923:i32)
              n1543 = Divide(x=w1923, y=2) -> (x/y=w1924:dbl)
              n1544 = for {
                N: w1924 -> [_]
                shift-right: [w1949] -> _
                shift-left: w1809 -> [w1951]
                shift-right: [w1944] -> w1922
                shift-left: i64[] [] ("edited\nto play 3") -> [w1945]
                n1545 = Split 1D Array(array=w1951, index=2) -> (first subarray=w1950:i64[], second subarray=w1949:i64[])
                n1546 = Index Array(array=w1950, index #1=1 ("index"), index #2=0 ("index")) -> (element #1=w1955:i64, element #2=w1948:i64)
                n1547 = Subtract(x=w1955, y=w1948) -> (x-y=w1947:i64)
                n1548 = Increment(x=w1947) -> (x+1=w1946:i64)
                n1549 = for {
                  N: w1946 -> [_]
                  tunnel: w1948 -> [w1958]
                  tunnel: [w1956] -> w1943 mode=indexing
                  tunnel: [w1956] -> _
                  i -> [w1957]
                  n1550 = Add(x=w1958, y=w1957) -> (x+y=w1956:i64)
                }
                n1551 = Insert Into Array(array=w1945, new element=w1943) -> (w1944:i64[])  [unwired: 1 in]
              }
              n1552 = local read "Number of Frames"() -> (w1937:u32)
              n1553 = Subtract(x=w1937, y=u32 2) -> (x-y=w1939:u32)
              n1554 = In Range and Coerce(upper limit=0, x=w1922, lower limit=w1939) -> (coerced(x)=w1807:i64[])  [unwired: 1 out]
              "frames edited" <- w1807
              "frames 2 play" <- w1807
              n1555 = for {
                tunnel: w1807 -> [_] mode=indexing
                shift-right: [w2015] -> _
                shift-left: w1807 -> [w2014]
                i -> [w2011]
                n1556 = Index Array(array=w2014, index=w2011) -> (element=w2013:i64)
                n1557 = Increment(x=w2011) -> (x+1=w2012:i32)
                n1558 = while {
                  shift-right: [w2020] -> w2015
                  shift-left: w2014 -> [w2021]
                  tunnel: w2013 -> [w2022]
                  tunnel: w2012 -> [w2016]
                  stop <- w2017 stop-if-true
                  n1559 = Search 1D Array(1D array=w2021, element=w2022, start index (0)=w2016) -> (index of element=w2019:i32)
                  n1560 = Equal?(x=w2019, y=-1) -> (x = y?=w2017:bool)
                  n1561 = Delete From Array(array=w2021, index=w2019) -> (array with subset deleted=w2020:i64[])  [unwired: 1 in, 1 out]
                }
              }
            }
          }
          n1562 = local read "refnum of data save file"() -> (w1754:refnum<file>)
        }
        frame "Examine coding" {
          w2100 = T4."Enabled" ("Disabled")
          n1563 = property on="Code number display" class="DigNum (strict)"("DisabledEnum"=w2100) -> ()  [unwired: 2 in, 2 out]
          n1564 = property on="Next" class="Bool (strict)"("DisabledEnum"=w2100) -> ()  [unwired: 2 in, 2 out]
          n1565 = property on="Reset" class="Bool (strict)"("DisabledEnum"=w2100) -> ()  [unwired: 2 in, 2 out]
          n1566 = property on="Update" class="Bool (strict)"("DisabledEnum"=w2100) -> ()  [unwired: 2 in, 2 out]
          n1567 = property on="Previous" class="Bool (strict)"("DisabledEnum"=w2100) -> ()  [unwired: 2 in, 2 out]
          n1568 = local read "edited\nevents"() -> (w2108:i64[][])
          n1569 = Decrement(x="Code number display") -> (x-1=w2101:i32)
          n1570 = flat-sequence {
            tunnel: "Code number display" -> [w2125]
            frame #0 {
              n1571 = local read "edited to play"() -> (w2124:i64[])
              n1572 = for {
                N: w2125 -> [_]
                shift-right: [w2130] -> _
                shift-left: w2124 -> [w2131]
                tunnel: [w2129] -> w2117
                n1573 = Split 1D Array(array=w2131, index=2) -> (first subarray=w2129:i64[], second subarray=w2130:i64[])
              }
              n1574 = Index Array(array=w2117, index #1=1 ("index"), index #2=0 ("index")) -> (element #1=w2123:i64, element #2=w2120:i64)
              n1575 = Subtract(x=w2123, y=w2120) -> (x-y=w2119:i64)
              n1576 = Increment(x=w2119) -> (x+1=w2118:i64)
              n1577 = for {
                N: w2118 -> [_]
                tunnel: w2120 -> [w2128]
                tunnel: [w2126] -> w2116 mode=indexing
                i -> [w2127]
                n1578 = Add(x=w2128, y=w2127) -> (x+y=w2126:i64)
              }
              n1579 = local write "Progress..."(u32 0 ("Progress...")) -> ()
              n1580 = local write "frames 2 play"(w2116) -> ()
            }
            frame #1 {
              w2133 = TRUE ("Play")
              w2134 = FALSE ("Next")
              n1581 = local write "Next"(w2134) -> ()
              n1582 = local write "Previous"(w2134) -> ()
              n1583 = local write "Reset"(w2134) -> ()
              n1584 = local write "stop"(w2134) -> ()
              n1585 = local write "Pause"(w2134) -> ()
              n1586 = local write "Load video"(w2133) -> ()
              n1587 = local write "Play"(w2133) -> ()
            }
          }
          n1588 = Index Array(array=w2108, index (row)=w2101, index (col)=0) -> (element=w2107:i64)
          n1589 = Index Array(array=w2105, index (col)=0 ("disabled index (col)")) -> (element=w2112:i64[])  [unwired: 1 in]
          n1590 = Search 1D Array(1D array=w2112, element=w2107) -> (index of element=w2111:i32)  [unwired: 1 in]
          n1591 = Index Array(array=w2105, index (row)=w2111) -> (element=w2110:i64[])  [unwired: 1 in]
          n1592 = Delete From Array(array=w2110, length=3, index=0) -> (array with subset deleted=w2109:i64[])  [unwired: 1 out]
          n1593 = for {
            tunnel: w2109 -> [w2139] mode=indexing
            tunnel: [w2135] -> w2023 mode=indexing
            n1594 = Equal To 0?(x=w2139) -> (x = 0?=w2138:bool)
            n1595 = Select(t=FALSE ("x = 0?"), s=w2138, f=TRUE) -> (s? t:f=w2135:bool)
          }
          n1596 = Split 1D Array(array=w2023, index=24) -> (first subarray=w2048:bool[], second subarray=w2049:bool[])
          n1597 = Index Array(array=w2048) -> (element #1=w2047:bool, element #2=w2046:bool, element #3=w2045:bool, element #4=w2044:bool, element #5=w2043:bool, element #6=w2042:bool, element #7=w2041:bool, element #8=w2040:bool, element #9=w2039:bool, element #10=w2038:bool, element #11=w2037:bool, element #12=w2036:bool, element #13=w2035:bool, element #14=w2034:bool, element #15=w2033:bool, element #16=w2032:bool, element #17=w2031:bool, element #18=w2030:bool, element #19=w2029:bool, element #20=w2028:bool, element #21=w2027:bool, element #22=w2026:bool, element #23=w2025:bool, element #24=w2024:bool)  [unwired: 30 in, 6 out]
          n1598 = Split 1D Array(array=w2049, index=34) -> (first subarray=w2050:bool[], second subarray=w2051:bool[])
          n1599 = local write "1 10"(w2047) -> ()
          n1600 = local write "1 7"(w2046) -> ()
          n1601 = local write "1 6"(w2045) -> ()
          n1602 = local write "1 5"(w2044) -> ()
          n1603 = local write "2 10"(w2043) -> ()
          n1604 = local write "2 7"(w2042) -> ()
          n1605 = local write "2 6"(w2041) -> ()
          n1606 = local write "2 5"(w2040) -> ()
          n1607 = local write "3 9"(w2039) -> ()
          n1608 = local write "3 7"(w2038) -> ()
          n1609 = local write "3 6"(w2037) -> ()
          n1610 = local write "3 5"(w2036) -> ()
          n1611 = local write "4 9"(w2035) -> ()
          n1612 = local write "4 7"(w2034) -> ()
          n1613 = local write "4 6"(w2033) -> ()
          n1614 = local write "4 5"(w2032) -> ()
          n1615 = local write "5 8"(w2031) -> ()
          n1616 = local write "5 7"(w2030) -> ()
          n1617 = local write "5 6"(w2029) -> ()
          n1618 = local write "5 5"(w2028) -> ()
          n1619 = local write "6 8"(w2027) -> ()
          n1620 = local write "6 7"(w2026) -> ()
          n1621 = local write "6 6"(w2025) -> ()
          n1622 = local write "6 5"(w2024) -> ()
          n1623 = Index Array(array=w2050) -> (element #1=w2097:bool, element #2=w2096:bool, element #3=w2095:bool, element #4=w2094:bool, element #5=w2093:bool, element #6=w2092:bool, element #7=w2091:bool, element #8=w2090:bool, element #9=w2089:bool, element #10=w2088:bool, element #11=w2087:bool, element #12=w2086:bool, element #13=w2085:bool, element #14=w2084:bool, element #15=w2083:bool, element #16=w2082:bool, element #17=w2081:bool, element #18=w2080:bool, element #19=w2079:bool, element #20=w2078:bool, element #21=w2077:bool, element #22=w2076:bool, element #23=w2075:bool, element #24=w2074:bool, element #25=w2073:bool, element #26=w2072:bool, element #27=w2071:bool, element #28=w2070:bool, element #29=w2069:bool, element #30=w2068:bool)  [unwired: 30 in]
          n1624 = local write "Adrive"(w2097) -> ()
          n1625 = local write "Ddrive"(w2096) -> ()
          n1626 = local write "ASWdrive"(w2095) -> ()
          n1627 = local write "DSWdrive"(w2094) -> ()
          n1628 = local write "Drop 14"(w2093) -> ()
          n1629 = local write "Chop 13"(w2092) -> ()
          n1630 = local write "Lob"(w2091) -> ()
          n1631 = local write "Boast2"(w2090) -> ()
          n1632 = local write "Boast3"(w2089) -> ()
          n1633 = local write "Smash 13"(w2088) -> ()
          n1634 = local write "FH"(w2087) -> ()
          n1635 = local write "BH"(w2086) -> ()
          n1636 = local write "ST"(w2085) -> ()
          n1637 = local write "CR"(w2084) -> ()
          n1638 = local write "Bounce"(w2083) -> ()
          n1639 = local write "Half Volley"(w2082) -> ()
          n1640 = local write "Volley"(w2081) -> ()
          n1641 = local write "Expected Winner1 2"(w2080) -> ()
          n1642 = local write "Expected Winner2 2"(w2079) -> ()
          n1643 = local write "Unexpected Winner1 2"(w2078) -> ()
          n1644 = local write "Unexpected Winner2 2"(w2077) -> ()
          n1645 = local write "Stroke1 2"(w2076) -> ()
          n1646 = local write "Stroke2 2"(w2075) -> ()
          n1647 = local write "Forced Error1 2"(w2074) -> ()
          n1648 = local write "Forced Error2 2"(w2073) -> ()
          n1649 = local write "Unforced Error1 2"(w2072) -> ()
          n1650 = local write "Unforced Error2 2"(w2071) -> ()
          n1651 = local write "Nolet1 2"(w2070) -> ()
          n1652 = local write "Nolet2 2"(w2069) -> ()
          n1653 = local write "Let 2"(w2068) -> ()
          n1654 = Index Array(array=w2051) -> (element #1=w2067:bool, element #2=w2066:bool, element #3=w2065:bool, element #4=w2064:bool, element #5=w2063:bool, element #6=w2062:bool, element #7=w2061:bool, element #8=w2060:bool, element #9=w2059:bool, element #10=w2058:bool, element #11=w2057:bool, element #12=w2056:bool, element #13=w2055:bool, element #14=w2054:bool, element #15=w2053:bool)  [unwired: 15 in]
          n1655 = local write "Service1 2"(w2067) -> ()
          n1656 = local write "Service2 2"(w2066) -> ()
          n1657 = local write "S1 2"(w2065) -> ()
          n1658 = local write "S2 2"(w2064) -> ()
          n1659 = local write "S3 2"(w2063) -> ()
          n1660 = local write "S4 2"(w2062) -> ()
          n1661 = local write "S5 2"(w2061) -> ()
          n1662 = local write "S6 2"(w2060) -> ()
          n1663 = local write "Player1 2"(w2059) -> ()
          n1664 = local write "Player2 2"(w2058) -> ()
          n1665 = local write "Button 6"(w2057) -> ()
          n1666 = local write "Button 7"(w2056) -> ()
          n1667 = local write "Button 8"(w2055) -> ()
          n1668 = local write "Button 9"(w2054) -> ()
          n1669 = local write "Button 10"(w2053) -> ()
          n1670 = local read "refnum of data save file"() -> (w2103:refnum<file>)
        }
        frame "Edit coding" {
          n1671 = local read "Examine code"() -> (w2141:bool)
          n1672 = case shown="False" w2141 {
            tunnel: [T1."Edit video" ("Main tab") w2224] -> w2143
            frame False {
              n1673 = local read "Last Edit"() -> (w2218:bool[])
              n1674 = Split 1D Array(array=w2218, index=24) -> (first subarray=w2168:bool[], second subarray=w2169:bool[])
              n1675 = Index Array(array=w2168) -> (element #1=w2167:bool, element #2=w2166:bool, element #3=w2165:bool, element #4=w2164:bool, element #5=w2163:bool, element #6=w2162:bool, element #7=w2161:bool, element #8=w2160:bool, element #9=w2159:bool, element #10=w2158:bool, element #11=w2157:bool, element #12=w2156:bool, element #13=w2155:bool, element #14=w2154:bool, element #15=w2153:bool, element #16=w2152:bool, element #17=w2151:bool, element #18=w2150:bool, element #19=w2149:bool, element #20=w2148:bool, element #21=w2147:bool, element #22=w2146:bool, element #23=w2145:bool, element #24=w2144:bool)  [unwired: 30 in, 6 out]
              n1676 = Split 1D Array(array=w2169, index=30) -> (first subarray=w2170:bool[], second subarray=w2171:bool[])
              n1677 = local write "1 10"(w2167) -> ()
              n1678 = local write "1 7"(w2166) -> ()
              n1679 = local write "1 6"(w2165) -> ()
              n1680 = local write "1 5"(w2164) -> ()
              n1681 = local write "2 10"(w2163) -> ()
              n1682 = local write "2 7"(w2162) -> ()
              n1683 = local write "2 6"(w2161) -> ()
              n1684 = local write "2 5"(w2160) -> ()
              n1685 = local write "3 9"(w2159) -> ()
              n1686 = local write "3 7"(w2158) -> ()
              n1687 = local write "3 6"(w2157) -> ()
              n1688 = local write "3 5"(w2156) -> ()
              n1689 = local write "4 9"(w2155) -> ()
              n1690 = local write "4 7"(w2154) -> ()
              n1691 = local write "4 6"(w2153) -> ()
              n1692 = local write "4 5"(w2152) -> ()
              n1693 = local write "5 8"(w2151) -> ()
              n1694 = local write "5 7"(w2150) -> ()
              n1695 = local write "5 6"(w2149) -> ()
              n1696 = local write "5 5"(w2148) -> ()
              n1697 = local write "6 8"(w2147) -> ()
              n1698 = local write "6 7"(w2146) -> ()
              n1699 = local write "6 6"(w2145) -> ()
              n1700 = local write "6 5"(w2144) -> ()
              n1701 = Index Array(array=w2170) -> (element #1=w2217:bool, element #2=w2216:bool, element #3=w2215:bool, element #4=w2214:bool, element #5=w2213:bool, element #6=w2212:bool, element #7=w2211:bool, element #8=w2210:bool, element #9=w2209:bool, element #10=w2208:bool, element #11=w2207:bool, element #12=w2206:bool, element #13=w2205:bool, element #14=w2204:bool, element #15=w2203:bool, element #16=w2202:bool, element #17=w2201:bool, element #18=w2200:bool, element #19=w2199:bool, element #20=w2198:bool, element #21=w2197:bool, element #22=w2196:bool, element #23=w2195:bool, element #24=w2194:bool, element #25=w2193:bool, element #26=w2192:bool, element #27=w2191:bool, element #28=w2190:bool, element #29=w2189:bool, element #30=w2188:bool)  [unwired: 30 in]
              n1702 = local write "Adrive"(w2217) -> ()
              n1703 = local write "Ddrive"(w2216) -> ()
              n1704 = local write "ASWdrive"(w2215) -> ()
              n1705 = local write "DSWdrive"(w2214) -> ()
              n1706 = local write "Drop 14"(w2213) -> ()
              n1707 = local write "Chop 13"(w2212) -> ()
              n1708 = local write "Lob"(w2211) -> ()
              n1709 = local write "Boast2"(w2210) -> ()
              n1710 = local write "Boast3"(w2209) -> ()
              n1711 = local write "Smash 13"(w2208) -> ()
              n1712 = local write "FH"(w2207) -> ()
              n1713 = local write "BH"(w2206) -> ()
              n1714 = local write "ST"(w2205) -> ()
              n1715 = local write "CR"(w2204) -> ()
              n1716 = local write "Bounce"(w2203) -> ()
              n1717 = local write "Half Volley"(w2202) -> ()
              n1718 = local write "Volley"(w2201) -> ()
              n1719 = local write "Expected Winner1 2"(w2200) -> ()
              n1720 = local write "Expected Winner2 2"(w2199) -> ()
              n1721 = local write "Unexpected Winner1 2"(w2198) -> ()
              n1722 = local write "Unexpected Winner2 2"(w2197) -> ()
              n1723 = local write "Stroke1 2"(w2196) -> ()
              n1724 = local write "Stroke2 2"(w2195) -> ()
              n1725 = local write "Forced Error1 2"(w2194) -> ()
              n1726 = local write "Forced Error2 2"(w2193) -> ()
              n1727 = local write "Unforced Error1 2"(w2192) -> ()
              n1728 = local write "Unforced Error2 2"(w2191) -> ()
              n1729 = local write "Nolet1 2"(w2190) -> ()
              n1730 = local write "Nolet2 2"(w2189) -> ()
              n1731 = local write "Let 2"(w2188) -> ()
              n1732 = Index Array(array=w2171) -> (element #1=w2187:bool, element #2=w2186:bool, element #3=w2185:bool, element #4=w2184:bool, element #5=w2183:bool, element #6=w2182:bool, element #7=w2181:bool, element #8=w2180:bool, element #9=w2179:bool, element #10=w2178:bool, element #11=w2177:bool, element #12=w2176:bool, element #13=w2175:bool, element #14=w2174:bool, element #15=w2173:bool)  [unwired: 15 in]
              n1733 = local write "Service1 2"(w2187) -> ()
              n1734 = local write "Service2 2"(w2186) -> ()
              n1735 = local write "S1 2"(w2185) -> ()
              n1736 = local write "S2 2"(w2184) -> ()
              n1737 = local write "S3 2"(w2183) -> ()
              n1738 = local write "S4 2"(w2182) -> ()
              n1739 = local write "S5 2"(w2181) -> ()
              n1740 = local write "S6 2"(w2180) -> ()
              n1741 = local write "Player1 2"(w2179) -> ()
              n1742 = local write "Player2 2"(w2178) -> ()
              n1743 = local write "Button 6"(w2177) -> ()
              n1744 = local write "Button 7"(w2176) -> ()
              n1745 = local write "Button 8"(w2175) -> ()
              n1746 = local write "Button 9"(w2174) -> ()
              n1747 = local write "Button 10"(w2173) -> ()
              n1748 = local write "Upload edited video"(TRUE ("Upload edited video")) -> ()
            }
            frame True {
              n1749 = event shown="[0] Timeout" {
                selector: _ -> [_ _]
                dyn-events: _ -> [_ _]
                timeout: 25 -> [_ _]
                tunnel: [FALSE TRUE] -> w2222
                event Timeout {
                  n1750 = event-data() -> ()  [unwired: 1 in, 3 out]
                }
                event "Code number display": Value Change {
                  n1751 = event-data() -> ()  [unwired: 1 in, 3 out]
                }
              }
              n1752 = case shown="True" "Next" {
                frame False {
                }
                frame True {
                  n1753 = local read "edited\nevents"() -> (w2241:i64[][])
                  n1754 = local read "Code number display"() -> (w2237:i32)
                  n1755 = Index Array(array=w2241, index (col)=0 ("disabled index (col)")) -> (element=w2243:i64[])  [unwired: 1 in]
                  n1756 = Array Size(array=w2243) -> (size(s)=w2236:i32)
                  n1757 = Increment(x=w2237) -> (x+1=w2239:i32)
                  n1758 = Less Or Equal?(x=w2239, y=w2236) -> (x <= y?=w2240:bool)
                  n1759 = Select(t=w2239, s=w2240, f=w2236) -> (s? t:f=w2238:i32)
                  n1760 = local write "Code number display"(w2238) -> ()
                }
              }
              n1761 = case shown="True" "Previous" {
                frame False {
                }
                frame True {
                  n1762 = local read "Code number display"() -> (w2244:i32)
                  n1763 = Decrement(x=w2244) -> (x-1=w2247:i32)
                  n1764 = Greater Than 0?(x=w2247) -> (x > 0?=w2248:bool)
                  n1765 = Select(t=w2247, s=w2248, f=1) -> (s? t:f=w2245:i32)
                  n1766 = local write "Code number display"(w2245) -> ()
                }
              }
              n1767 = Compound Arithmetic op=OR(w2222, "Reset", "Previous", "Next") -> (w2230:bool)
              n1768 = Select(t=T1."Examine coding" ("Main tab"), s=w2230, f=T1."Edit coding" ("Main tab")) -> (s? t:f=w2225:T1)
              n1769 = Select(t=T1."Update coding" ("Main tab"), s="Update", f=w2225) -> (s? t:f=w2224:T1)
            }
          }
          n1770 = local read "refnum of data save file"() -> (w2140:refnum<file>)
        }
        frame "Update coding" {
          w2249 = "\t"
          w2273 = "\r"
          n1771 = flat-sequence {
            tunnel: w2277 -> [w2370]
            tunnel: [w2367] -> w2276
            tunnel: w2276 -> [w2454]
            tunnel: [w2454] -> w2259
            frame #0 {
              w2316 = FALSE
              n1772 = local read "Service1 2"() -> (w2315:bool)
              n1773 = local read "Service2 2"() -> (w2314:bool)
              n1774 = local read "Button 10"() -> (w2301:bool)
              n1775 = local read "Player1 2"() -> (w2307:bool)
              n1776 = local read "Player2 2"() -> (w2306:bool)
              n1777 = local read "Button 6"() -> (w2305:bool)
              n1778 = local read "Button 7"() -> (w2304:bool)
              n1779 = local read "Button 8"() -> (w2303:bool)
              n1780 = local read "Button 9"() -> (w2302:bool)
              n1781 = local read "S1 2"() -> (w2313:bool)
              n1782 = local read "S2 2"() -> (w2312:bool)
              n1783 = local read "S3 2"() -> (w2311:bool)
              n1784 = local read "S4 2"() -> (w2310:bool)
              n1785 = local read "S5 2"() -> (w2309:bool)
              n1786 = local read "S6 2"() -> (w2308:bool)
              n1787 = local read "1 10"() -> (w2364:bool)
              n1788 = local read "2 10"() -> (w2360:bool)
              n1789 = local read "5 8"() -> (w2296:bool)
              n1790 = local read "5 7"() -> (w2295:bool)
              n1791 = local read "5 6"() -> (w2294:bool)
              n1792 = local read "5 5"() -> (w2293:bool)
              n1793 = local read "6 8"() -> (w2292:bool)
              n1794 = local read "6 7"() -> (w2291:bool)
              n1795 = local read "6 6"() -> (w2290:bool)
              n1796 = local read "6 5"() -> (w2289:bool)
              n1797 = local read "1 7"() -> (w2363:bool)
              n1798 = local read "1 6"() -> (w2362:bool)
              n1799 = local read "1 5"() -> (w2361:bool)
              n1800 = local read "2 7"() -> (w2359:bool)
              n1801 = local read "2 6"() -> (w2358:bool)
              n1802 = local read "2 5"() -> (w2357:bool)
              n1803 = local read "3 9"() -> (w2356:bool)
              n1804 = local read "3 7"() -> (w2355:bool)
              n1805 = local read "3 6"() -> (w2354:bool)
              n1806 = local read "3 5"() -> (w2353:bool)
              n1807 = local read "4 9"() -> (w2352:bool)
              n1808 = local read "4 7"() -> (w2351:bool)
              n1809 = local read "4 6"() -> (w2350:bool)
              n1810 = local read "4 5"() -> (w2349:bool)
              n1811 = Build Array(w2315, w2314, w2313, w2312, w2311, w2310, w2309, w2308, w2307, w2306, w2305, w2304, w2303, w2302, w2301) -> (w2298:bool[])
              n1812 = Build Array(w2364, w2363, w2362, w2361, w2360, w2359, w2358, w2357, w2356, w2355, w2354, w2353, w2352, w2351, w2350, w2349, w2296, w2295, w2294, w2293, w2292, w2291, w2290, w2289) -> (w2300:bool[])
              n1813 = local read "Unexpected Winner1 2"() -> (w2329:bool)
              n1814 = local read "Unexpected Winner2 2"() -> (w2322:bool)
              n1815 = local read "Expected Winner1 2"() -> (w2330:bool)
              n1816 = local read "Expected Winner2 2"() -> (w2323:bool)
              n1817 = local read "Unforced Error1 2"() -> (w2319:bool)
              n1818 = local read "Unforced Error2 2"() -> (w2326:bool)
              n1819 = local read "Forced Error1 2"() -> (w2320:bool)
              n1820 = local read "Forced Error2 2"() -> (w2327:bool)
              n1821 = local read "ASWdrive"() -> (w2346:bool)
              n1822 = local read "DSWdrive"() -> (w2345:bool)
              n1823 = local read "Smash 13"() -> (w2339:bool)
              n1824 = local read "Stroke1 2"() -> (w2328:bool)
              n1825 = local read "Stroke2 2"() -> (w2321:bool)
              n1826 = local read "Volley"() -> (w2332:bool)
              n1827 = local read "Chop 13"() -> (w2343:bool)
              n1828 = local read "Half Volley"() -> (w2333:bool)
              n1829 = local read "Nolet1 2"() -> (w2318:bool)
              n1830 = local read "Nolet2 2"() -> (w2325:bool)
              n1831 = local read "Drop 14"() -> (w2344:bool)
              n1832 = local read "Bounce"() -> (w2334:bool)
              n1833 = local read "Boast2"() -> (w2341:bool)
              n1834 = local read "Boast3"() -> (w2340:bool)
              n1835 = local read "Adrive"() -> (w2348:bool)
              n1836 = local read "Ddrive"() -> (w2347:bool)
              n1837 = local read "Let 2"() -> (w2331:bool)
              n1838 = local read "Lob"() -> (w2342:bool)
              n1839 = local read "BH"() -> (w2337:bool)
              n1840 = local read "FH"() -> (w2338:bool)
              n1841 = local read "CR"() -> (w2335:bool)
              n1842 = local read "ST"() -> (w2336:bool)
              n1843 = Compound Arithmetic op=OR(w2323, w2322, w2321, w2320, w2319, w2318) -> (w2317:bool)
              n1844 = Compound Arithmetic op=OR(w2330, w2329, w2328, w2327, w2326, w2325) -> (w2324:bool)
              n1845 = Build Array(w2348, w2347, w2346, w2345, w2344, w2343, w2342, w2341, w2340, w2339, w2338, w2337, w2336, w2335, w2334, w2333, w2332, w2330, w2323, w2329, w2322, w2328, w2321, w2320, w2327, w2319, w2326, w2318, w2325, w2331, w2324, w2317, w2316, w2316) -> (w2299:bool[])
              n1846 = Insert Into Array(array=w2300, new element #1=w2299, new element #2=w2298) -> (w2297:bool[])  [unwired: 1 in]
              n1847 = Boolean To (0,1)(Boolean=w2297) -> (0, 1=w2371:i16[])
              "0, 1" <- w2371
              n1848 = local read "Code number display"() -> (w2366:i32)
              n1849 = local read "edited\nevents"() -> (w2372:i64[][])
              n1850 = Decrement(x=w2366) -> (x-1=w2365:i32)
              n1851 = Index Array(array=w2370, index (col)=0 ("disabled index (col)")) -> (element=w2375:i64[])  [unwired: 1 in]
              n1852 = Index Array(array=w2372, index (row)=w2365, index (col)=0) -> (element=w2374:i64)
              n1853 = Search 1D Array(1D array=w2375, element=w2374) -> (index of element=w2368:i32)  [unwired: 1 in]
              n1854 = Index Array(array=w2370, index (row)=w2368) -> (element=w2288:i64[])  [unwired: 1 in]
              n1855 = Delete From Array(array=w2288, index=0) -> ()  [unwired: 1 in, 2 out]
              n1856 = Index Array(array=w2288, index #1=0 ("index"), index #2=1 ("index"), index #3=2 ("index")) -> (element #1=w2287:i64, element #2=w2286:i64, element #3=w2285:i64)
              n1857 = Build Array (concatenate)(w2287, w2286, w2285, w2371) -> (w2369:i64[])
              "appended array" <- w2369
              n1858 = Replace Array Subset(array=w2370, new element=w2369, index (row)=w2368) -> (w2367:i64[][])  [unwired: 1 in]
              "output array" <- w2367
            }
            frame #1 {
              n1859 = local read "Last Edit"() -> (w2452:bool[])
              n1860 = Split 1D Array(array=w2452, index=24) -> (first subarray=w2402:bool[], second subarray=w2403:bool[])
              n1861 = Index Array(array=w2402) -> (element #1=w2401:bool, element #2=w2400:bool, element #3=w2399:bool, element #4=w2398:bool, element #5=w2397:bool, element #6=w2396:bool, element #7=w2395:bool, element #8=w2394:bool, element #9=w2393:bool, element #10=w2392:bool, element #11=w2391:bool, element #12=w2390:bool, element #13=w2389:bool, element #14=w2388:bool, element #15=w2387:bool, element #16=w2386:bool, element #17=w2385:bool, element #18=w2384:bool, element #19=w2383:bool, element #20=w2382:bool, element #21=w2381:bool, element #22=w2380:bool, element #23=w2379:bool, element #24=w2378:bool)  [unwired: 30 in, 6 out]
              n1862 = Split 1D Array(array=w2403, index=30) -> (first subarray=w2404:bool[], second subarray=w2405:bool[])
              n1863 = local write "1 10"(w2401) -> ()
              n1864 = local write "1 7"(w2400) -> ()
              n1865 = local write "1 6"(w2399) -> ()
              n1866 = local write "1 5"(w2398) -> ()
              n1867 = local write "2 10"(w2397) -> ()
              n1868 = local write "2 7"(w2396) -> ()
              n1869 = local write "2 6"(w2395) -> ()
              n1870 = local write "2 5"(w2394) -> ()
              n1871 = local write "3 9"(w2393) -> ()
              n1872 = local write "3 7"(w2392) -> ()
              n1873 = local write "3 6"(w2391) -> ()
              n1874 = local write "3 5"(w2390) -> ()
              n1875 = local write "4 9"(w2389) -> ()
              n1876 = local write "4 7"(w2388) -> ()
              n1877 = local write "4 6"(w2387) -> ()
              n1878 = local write "4 5"(w2386) -> ()
              n1879 = local write "5 8"(w2385) -> ()
              n1880 = local write "5 7"(w2384) -> ()
              n1881 = local write "5 6"(w2383) -> ()
              n1882 = local write "5 5"(w2382) -> ()
              n1883 = local write "6 8"(w2381) -> ()
              n1884 = local write "6 7"(w2380) -> ()
              n1885 = local write "6 6"(w2379) -> ()
              n1886 = local write "6 5"(w2378) -> ()
              n1887 = Index Array(array=w2404) -> (element #1=w2451:bool, element #2=w2450:bool, element #3=w2449:bool, element #4=w2448:bool, element #5=w2447:bool, element #6=w2446:bool, element #7=w2445:bool, element #8=w2444:bool, element #9=w2443:bool, element #10=w2442:bool, element #11=w2441:bool, element #12=w2440:bool, element #13=w2439:bool, element #14=w2438:bool, element #15=w2437:bool, element #16=w2436:bool, element #17=w2435:bool, element #18=w2434:bool, element #19=w2433:bool, element #20=w2432:bool, element #21=w2431:bool, element #22=w2430:bool, element #23=w2429:bool, element #24=w2428:bool, element #25=w2427:bool, element #26=w2426:bool, element #27=w2425:bool, element #28=w2424:bool, element #29=w2423:bool, element #30=w2422:bool)  [unwired: 30 in]
              n1888 = local write "Adrive"(w2451) -> ()
              n1889 = local write "Ddrive"(w2450) -> ()
              n1890 = local write "ASWdrive"(w2449) -> ()
              n1891 = local write "DSWdrive"(w2448) -> ()
              n1892 = local write "Drop 14"(w2447) -> ()
              n1893 = local write "Chop 13"(w2446) -> ()
              n1894 = local write "Lob"(w2445) -> ()
              n1895 = local write "Boast2"(w2444) -> ()
              n1896 = local write "Boast3"(w2443) -> ()
              n1897 = local write "Smash 13"(w2442) -> ()
              n1898 = local write "FH"(w2441) -> ()
              n1899 = local write "BH"(w2440) -> ()
              n1900 = local write "ST"(w2439) -> ()
              n1901 = local write "CR"(w2438) -> ()
              n1902 = local write "Bounce"(w2437) -> ()
              n1903 = local write "Half Volley"(w2436) -> ()
              n1904 = local write "Volley"(w2435) -> ()
              n1905 = local write "Expected Winner1 2"(w2434) -> ()
              n1906 = local write "Expected Winner2 2"(w2433) -> ()
              n1907 = local write "Unexpected Winner1 2"(w2432) -> ()
              n1908 = local write "Unexpected Winner2 2"(w2431) -> ()
              n1909 = local write "Stroke1 2"(w2430) -> ()
              n1910 = local write "Stroke2 2"(w2429) -> ()
              n1911 = local write "Forced Error1 2"(w2428) -> ()
              n1912 = local write "Forced Error2 2"(w2427) -> ()
              n1913 = local write "Unforced Error1 2"(w2426) -> ()
              n1914 = local write "Unforced Error2 2"(w2425) -> ()
              n1915 = local write "Nolet1 2"(w2424) -> ()
              n1916 = local write "Nolet2 2"(w2423) -> ()
              n1917 = local write "Let 2"(w2422) -> ()
              n1918 = Index Array(array=w2405) -> (element #1=w2421:bool, element #2=w2420:bool, element #3=w2419:bool, element #4=w2418:bool, element #5=w2417:bool, element #6=w2416:bool, element #7=w2415:bool, element #8=w2414:bool, element #9=w2413:bool, element #10=w2412:bool, element #11=w2411:bool, element #12=w2410:bool, element #13=w2409:bool, element #14=w2408:bool, element #15=w2407:bool)  [unwired: 15 in]
              n1919 = local write "Service1 2"(w2421) -> ()
              n1920 = local write "Service2 2"(w2420) -> ()
              n1921 = local write "S1 2"(w2419) -> ()
              n1922 = local write "S2 2"(w2418) -> ()
              n1923 = local write "S3 2"(w2417) -> ()
              n1924 = local write "S4 2"(w2416) -> ()
              n1925 = local write "S5 2"(w2415) -> ()
              n1926 = local write "S6 2"(w2414) -> ()
              n1927 = local write "Player1 2"(w2413) -> ()
              n1928 = local write "Player2 2"(w2412) -> ()
              n1929 = local write "Button 6"(w2411) -> ()
              n1930 = local write "Button 7"(w2410) -> ()
              n1931 = local write "Button 8"(w2409) -> ()
              n1932 = local write "Button 9"(w2408) -> ()
              n1933 = local write "Button 10"(w2407) -> ()
            }
          }
          n1934 = local read "Btn 10"() -> (w2252:string)
          n1935 = local read "Btn 7"() -> (w2255:string)
          n1936 = local read "Btn 8"() -> (w2256:string)
          n1937 = local read "Btn 9"() -> (w2253:string)
          n1938 = local read "Btn 6"() -> (w2254:string)
          n1939 = Concatenate Strings(w2254, w2249, w2255, w2249, w2256, w2249, w2253, w2249, w2252, w2249, "Error" ("String")) -> (w2262:string)
          n1940 = for {
            tunnel: string[] ["frame number", "Lead", "Lag", "position 1", "position 2", "position 3", "position 4", "position 5", "position 6", "position 7", "position 8", "position 9", "position 10", "position 11", "position 12", "position 13", "position 14", "position 15", "position 16", "position 17", "position 18", "position 19", "position 20", "position 21", "position 22", "position 23", "position 24", "Drive A", "Drive D", "SW Drive A", "SW Drive D", "drop", "chop", "lob", "boast 2", "boast 3", "smash", "Forehand", "Backhand", "Straight", "Cross", "Bounce", "Half Volley", "Volley", "Expected winner 1", "Expected winner 2", "Unexpected winner 1", "Unexpected winner 2", "Stroke 1", "Stroke 2", "Forced error 1", "Forced error 2", "Unforced error 1", "Unforced error 2", "No let 1", "No let 2", "Let", "point1", "point2", "score1", "score2", "service1", "service2", "s1", "s2", "s3", "s4", "s5", "s6", "player1", "player2"] ("all rows") -> [w2281] mode=indexing
            tunnel: [w2279] -> w2260 mode=indexing
            n1941 = Concatenate Strings(w2281, "\t") -> (w2279:string)
          }
          n1942 = Concatenate Strings(w2260, w2262, "\r") -> (w2257:string)
          n1943 = Array To Spreadsheet String(delimiter (Tab)="\t" ("delimiter (\\t)"), array=w2259, 3:"%.3f" ("format (%.3f)")) -> (spreadsheet string=w2258:string)
          n1944 = local read "Video file"() -> (w2270:path)
          n1945 = local read "Data file"() -> (w2266:path)
          n1946 = call <vilib>:"Get File Extension.vi"("file"=w2270) -> ("filename without extension"=w2272:string)  [unwired: 7 in, 3 out]
          n1947 = Open/Create/Replace File(file path (use dialog)=w2266, operation (0:open)=T3."replace") -> (refnum out=w2268:refnum<file>, error out=w2267:errorcluster)  [unwired: 4 in, 1 out]
          n1948 = Concatenate Strings("avi file" ("string"), w2273, w2272, w2273, w2273, w2257, w2258) -> (w2274:string)
          n1949 = local write "Update"(FALSE ("Update")) -> ()
          n1950 = Write to Text File(file (use dialog)=w2268, text=w2274, error in=w2267) -> (refnum out=w2265:refnum<file>)  [unwired: 1 in, 2 out]
        }
      }
      "refnum of data save file" <- w374
      n1951 = Equal?(x="Main tab", y=enum32{"Coding", "Display"}."Coding" ("Tab Control 3")) -> (x = y?=w384:bool)
      n1952 = Not Equal?(x=w373, y=w379) -> (x != y?=w383:bool)
      n1953 = Select(t=w379, s=w384, f=w381) -> (s? t:f=w372:T1)
      n1954 = And(x=w383, y=w384) -> (x .and. y?=w382:bool)
      n1955 = Equal?(x=w373, y=w379) -> (x = y?=w378:bool)
      n1956 = Equal?(x=w372, y=w381) -> (x = y?=w380:bool)
      n1957 = And(x=w380, y=w378) -> (x .and. y?=w377:bool)
      n1958 = case shown="True" w382 {
        tunnel: w376 -> [_ w393]
        frame False {
        }
        frame True {
          # "Moving back to coding tab"
          n1959 = flat-sequence {
            tunnel: w393 -> [w397]
            frame #0 {
              n1960 = local read "ful video frames"() -> (w398:i64[])
              n1961 = Index Array(array=w397, index (col)=0 ("disabled index (col)")) -> (element=w395:i64[])  [unwired: 1 in]
              n1962 = Array Max & Min(array=w395) -> (max value=w394:i64)  [unwired: 3 out]
              n1963 = local write "frames 2 play"(w398) -> ()
              n1964 = local write "Progress..."(w394) -> ()
            }
            frame #1 {
              w399 = FALSE ("Next")
              w400 = TRUE ("Play")
              n1965 = local write "stop"(w400) -> ()
              n1966 = local write "Load video"(w400) -> ()
              n1967 = local write "Pause"(w399) -> ()
              n1968 = local write "Update"(w399) -> ()
              n1969 = local write "Next"(w399) -> ()
              n1970 = local write "Previous"(w399) -> ()
              n1971 = local write "Reset"(w399) -> ()
              n1972 = local write "Extract data"(w399) -> ()
              n1973 = local write "Upload edited video"(w399) -> ()
              n1974 = local write "Examine code"(w399) -> ()
            }
          }
        }
      }
      n1975 = case shown="True" w377 {
        frame False {
        }
        frame True {
          n1976 = local write "Progress..."(u32 0 ("Progress...")) -> ()
          n1977 = local write "Pause"(FALSE ("Pause")) -> ()
          n1978 = local write "stop"(TRUE ("stop")) -> ()
        }
      }
      n1979 = local read "START"() -> (w375:bool)
      n1980 = Wait (ms)(milliseconds to wait=u32 200) -> ()  [unwired: 1 out]
      "Main tab 2" <- w373
    }
    n1981 = while {
      tunnel: w10 -> [w223]
      tunnel: w1 -> [_]
      tunnel: [w218] -> w5
      stop <- w218 continue-if-true
      # "This loop is for writing\nvideo to disk"
      n1982 = local read "Video files to write"() -> (w222:string[])
      n1983 = local read "frames to write"() -> (w220:i64[][])
      n1984 = case shown="True" "Write file" {
        tunnel: [FALSE FALSE] -> w225
        tunnel: w223 -> [_ w243]
        tunnel: w222 -> [_ w242]
        tunnel: "Video to write" -> [_ w241]
        tunnel: w220 -> [_ w240]
        tunnel: [u32 0 ("milliseconds to wait") u32 0 ("milliseconds to wait")] -> w219
        frame False {
          w227 = T4."Enabled" ("Disabled")
          n1985 = local read "Video files to write"() -> (w231:string[])
          n1986 = property on="Add to lib" class="Bool (strict)"("DisabledEnum"=w227) -> ()  [unwired: 2 in, 2 out]
          n1987 = property on="File name" class="Str"("DisabledEnum"=w227) -> ()  [unwired: 2 in, 2 out]
          n1988 = property on="Video to write" class="Path"("DisabledEnum"=w227) -> ()  [unwired: 2 in, 2 out]
          n1989 = property on="START" class="Bool (strict)"("DisabledEnum"=w227) -> ()  [unwired: 2 in, 2 out]
          n1990 = Empty Array?(array=w231) -> (empty?=w230:bool)
          n1991 = Select(t=T4."Disabled and Grayed Out" ("Disabled"), s=w230, f=w227) -> (s? t:f=w228:T4)
          n1992 = property on="Write file" class="Bool (strict)"("DisabledEnum"=w228) -> ()  [unwired: 2 in, 2 out]
          n1993 = local write "Abort"(FALSE ("Abort")) -> ()
        }
        frame True {
          w235 = T4."Disabled and Grayed Out" ("Disabled")
          n1994 = for {
            tunnel: w240 -> [w282] mode=indexing
            tunnel: w242 -> [w273] mode=indexing
            tunnel: w241 -> [w272]
            tunnel: w243 -> [w260]
            tunnel: [w254] -> w238
            tunnel: [w253] -> w237
            tunnel: [w251] -> w236
            i -> [w255]
            stop <- w252 stop-if-true
            w269 = T5 4 items=["Grayscale (U8)", "Grayscale (I16)", "Grayscale (SGL)", "Complex (CSG)", "RGB (U32)", "HSL (U32)", "RGB (U64)"] ("Image Type")
            n1995 = Path To String(path=w272) -> (string=w274:string)
            n1996 = for {
              tunnel: w282 -> [w320] mode=indexing
              tunnel: [w320] -> w259 mode=indexing if=w319
              n1997 = Not Equal To 0?(x=w320) -> (x != 0?=w319:bool)
            }
            n1998 = Concatenate Strings(w274, "\\" ("string"), w273) -> (w277:string)
            n1999 = Array Size(array=w259) -> (size(s)=w258:i32)
            n2000 = Decrement(x=w255) -> (x-1=w256:i32)
            n2001 = Not Equal To 0?(x=w255) -> (x != 0?=w257:bool)
            n2002 = call <vilib>:"Search and Replace Pattern.vi"("string"=w277, "regular expression (\"\")"=".avi" ("regular expression (\"\")")) -> ("result string"=w281:string)  [unwired: 3 in, 1 out]
            n2003 = case shown="True" w257 {
              tunnel: w256 -> [_ w292]
              frame False {
              }
              frame True {
                n2004 = local read "Video files to write"() -> (w296:string[])
                n2005 = local read "frames to write"() -> (w293:i64[][])
                n2006 = Delete From Array(array=w296, index=w292) -> (array with subset deleted=w295:string[])  [unwired: 1 in, 1 out]
                n2007 = Delete From Array(array=w293, index (row)=w292) -> (array with subset deleted=w294:i64[][])  [unwired: 2 in, 1 out]
                n2008 = local write "frames to write"(w294) -> ()
                n2009 = local write "Video files to write"(w295) -> ()
              }
            }
            n2010 = property on="Writing" class="Slide (strict)"("Scale.Maximum"=w258) -> ()  [unwired: 2 in, 2 out]
            n2011 = Concatenate Strings(w281, ".avi" ("string")) -> (w279:string)
            n2012 = String To Path(string=w279) -> (path=w280:path)
            n2013 = while {
              shift-right: [w300] -> _
              shift-left: w280 -> [w299]
              tunnel: w281 -> [w304]
              tunnel: [w299] -> w250
              i -> [w298]
              stop <- w306 continue-if-true
              n2014 = Increment(x=w298) -> (x+1=w297:i32)
              n2015 = call <vilib>:"Check if File or Folder Exists.vi"("path"=w299) -> ("file or folder exists?"=w306:bool)  [unwired: 8 in, 2 out]
              n2016 = Number To Decimal String(number=w297) -> (decimal integer string=w303:string)  [unwired: 1 in]
              n2017 = Concatenate Strings(w304, " (file path clash) - " ("string"), w303, ".avi" ("string")) -> (w301:string)
              n2018 = String To Path(string=w301) -> (path=w300:path)
            }
            n2019 = Select(t="Microsoft Video 1" ("Codec Name"), s="Video compress", f="" ("Codec Name")) -> (s? t:f=w247:string)
            n2020 = local read "framesPerSecond"() -> (w263:u32)
            n2021 = call "IMAQ AVI Create"("Compression Filter"=w247, "Frames Per Second"=w263, "AVI Path"=w250) -> ("error out"=w270:errorcluster, "Avi Refnum"=w264:T6)  [unwired: 7 in]
            n2022 = call "IMAQ Create"("Image Name"="write", "Image Type"=w269, "error in (no error)"=w270) -> ("New Image"=w268:T2, "error out"=w267:errorcluster)  [unwired: 2 in]
            n2023 = for {
              tunnel: w259 -> [w317] mode=indexing
              tunnel: w268 -> [w311]
              tunnel: w267 -> [w316]
              tunnel: [w314] -> w266
              tunnel: [w313] -> w265
              tunnel: w264 -> [w312]
              tunnel: [w311] -> w261
              tunnel: w260 -> [w310]
              tunnel: ["Abort"] -> w252
              i -> [w309]
              stop <- "Abort" stop-if-true
              n2024 = Increment(x=w309) -> (x+1=→"Writing":i32)
              n2025 = call "IMAQ AVI Read Frame"("error in (no error)"=w316, "Frame Number"=w317, "Image"=w311, "Avi Refnum"=w310) -> ("error out"=w318:errorcluster, "Image Out"=w315:T2)  [unwired: 4 in, 2 out]
              n2026 = call "IMAQ AVI Write Frame"("error in (no error)"=w318, "Image"=w315, "Avi Refnum"=w312) -> ("error out"=w313:errorcluster, "Avi Refnum (duplicate)"=w314:T6)  [unwired: 7 in]
            }
            n2027 = call "IMAQ AVI Close"("error in (no error)"=w265, "Avi Refnum"=w266) -> ("error out"=w262:errorcluster)  [unwired: 9 in]
            n2028 = call "IMAQ Dispose"("Image"=w261, "error in (no error)"=w262) -> ("error out"=w249:errorcluster)  [unwired: 4 in]
            n2029 = case shown="False" w252 {
              tunnel: [string[] [] ("Video files to write") w290] -> w254
              tunnel: [i64[][] [] ("to write") w289] -> w253
              tunnel: ["Writing Complete" ("message") "Writing aborted" ("message")] -> w251
              tunnel: w250 -> [_ w287]
              tunnel: w249 -> [_ w286]
              frame False {
              }
              frame True {
                n2030 = local read "Video files to write"() -> (w290:string[])
                n2031 = Delete(path (use dialog)=w287, error in=w286) -> ()  [unwired: 3 in, 3 out]
                n2032 = local read "frames to write"() -> (w289:i64[][])
                n2033 = local write "Abort"(FALSE ("Abort")) -> ()
              }
            }
          }
          n2034 = One Button Dialog(message=w236) -> ()  [unwired: 1 in, 1 out]
          n2035 = local write "Video files to write"(w238) -> ()
          n2036 = local write "frames to write"(w237) -> ()
          n2037 = property on="Add to lib" class="Bool (strict)"("DisabledEnum"=w235) -> ()  [unwired: 2 in, 2 out]
          n2038 = property on="File name" class="Str"("DisabledEnum"=w235) -> ()  [unwired: 2 in, 2 out]
          n2039 = property on="Video to write" class="Path"("DisabledEnum"=w235) -> ()  [unwired: 2 in, 2 out]
          n2040 = property on="START" class="Bool (strict)"("DisabledEnum"=w235) -> ()  [unwired: 2 in, 2 out]
        }
      }
      n2041 = local read "START"() -> (w218:bool)
      n2042 = local write "Write file"(w225) -> ()
      n2043 = local write "Writing"(w219) -> ()
      n2044 = Wait (ms)(milliseconds to wait=u32 200) -> ()  [unwired: 1 out]
    }
    n2045 = while {
      tunnel: [w184] -> w6
      tunnel: w1 -> [_]
      stop <- w184 continue-if-true
      n2046 = case shown="True" "REPORT" {
        frame False {
        }
        frame True {
          w208 = TRUE ("open new instance (false)")
          n2047 = local read "Data file"() -> (w194:path)
          n2048 = local read "Video file"() -> (w193:path)
          n2049 = local write "REPORT"(FALSE ("REPORT")) -> ()
          n2050 = Strip Path(path=w194) -> (stripped path=w192:path)  [unwired: 1 out]
          n2051 = call <vilib>:"Get File Extension.vi"("file"=w193) -> ("filename without extension"=w189:string)  [unwired: 7 in, 3 out]
          n2052 = Path To String(path=w192) -> (string=w191:string)
          n2053 = Concatenate Strings(w191, "\\" ("string"), w189, " (BStAT Report).doc" ("string")) -> (w195:string)
          n2054 = String To Path(string=w195) -> (path=w197:path)
          n2055 = call <vilib>:"Check if File or Folder Exists.vi"("path"=w197) -> ("file or folder exists?"=w196:bool)  [unwired: 8 in, 2 out]
          n2056 = Automation Open(Automation Refnum=refnum<k7> refnum ("Word._Application"), 9:w208) -> (Automation Refnum=w201:refnum<k7>, error out=w202:errorcluster)  [unwired: 2 in]
          n2057 = property class="_Application"(reference=w201, error in=w202, "Visible"=w208) -> (reference out=w203:refnum<k7>, error out=w204:errorcluster)
          n2058 = case shown="True" w196 {
            tunnel: w197 -> [w211 w217]
            tunnel: [w210 w217] -> w187
            frame False {
              n2059 = Current VI's Path() -> (path=w214:path)
              n2060 = Strip Path(path=w214) -> (stripped path=w213:path)  [unwired: 1 out]
              n2061 = Build Path(base path=w213, name or relative path="BStAT report.doc") -> (appended path=w212:path)
              n2062 = One Button Dialog(message="***New report generated***\n\nRight-click on the white strip on the LEFT of the data area to copy the data ") -> ()  [unwired: 1 in, 1 out]
              n2063 = Copy(10:w211, 11:w212) -> (3:w210:path)  [unwired: 3 in, 2 out]
            }
            frame True {
              n2064 = One Button Dialog(message="***Report found***\n\nRight-click on the white strip on the LEFT of the data area to copy the data ") -> ()  [unwired: 1 in, 1 out]
            }
          }
          n2065 = property class="_Application"(reference=w203, error in=w204) -> (error out=w206:errorcluster, "Documents"=w205:refnum<k7>)  [unwired: 1 out]
          n2066 = invoke class="Documents" method="Open"(reference=w205, error in=w206, "FileName"=w187, "ReadOnly"=TRUE, "Visible"=TRUE) -> ()  [unwired: 14 in, 19 out]
        }
      }
      n2067 = local read "START"() -> (w184:bool)
      n2068 = Wait (ms)(milliseconds to wait=u32 200) -> ()  [unwired: 1 out]
    }
    n2069 = flat-sequence {
      tunnel: w7 -> [w33]
      tunnel: w6 -> [_]
      tunnel: w5 -> [_]
      tunnel: w4 -> [w34]
      frame #0 {
        w28 = T5 4 items=["Grayscale (U8)", "Grayscale (I16)", "Grayscale (SGL)", "Complex (CSG)", "RGB (U32)", "HSL (U32)", "RGB (U64)"] ("Image Type")
        w29 = T5 4 items=["Grayscale (U8)", "Grayscale (I16)", "Grayscale (SGL)", "Complex (CSG)", "RGB (U32)", "HSL (U32)", "RGB (U64)"] ("Image Type")
        w31 = T5 4 items=["Grayscale (U8)", "Grayscale (I16)", "Grayscale (SGL)", "Complex (CSG)", "RGB (U32)", "HSL (U32)", "RGB (U64)"] ("Image Type")
        n2070 = call "IMAQ AVI Close"("Avi Refnum"=w34) -> ("error out"=w32:errorcluster)  [unwired: 10 in]
        n2071 = Close File(refnum=w33, error in=w32) -> (error out=w26:errorcluster)  [unwired: 1 out]
        n2072 = call "IMAQ Create"("Image Name"="Video", "Image Type"=w28, "error in (no error)"=w26) -> ("New Image"=w22:T2, "error out"=w25:errorcluster)  [unwired: 2 in]
        n2073 = call "IMAQ Create"("Image Name"="pauselag", "Image Type"=w31, "error in (no error)"=w25) -> ("New Image"=w21:T2, "error out"=w23:errorcluster)  [unwired: 2 in]
        n2074 = call "IMAQ Create"("Image Name"="write", "Image Type"=w29, "error in (no error)"=w23) -> ("New Image"=w20:T2, "error out"=w19:errorcluster)  [unwired: 2 in]
        n2075 = call "IMAQ Dispose"("Image"=w22, "error in (no error)"=w19) -> ("error out"=w18:errorcluster)  [unwired: 4 in]
        n2076 = call "IMAQ Dispose"("Image"=w21, "error in (no error)"=w18) -> ("error out"=w17:errorcluster)  [unwired: 4 in]
        n2077 = call "IMAQ Dispose"("Image"=w20, "error in (no error)"=w17) -> ()  [unwired: 4 in, 1 out]
      }
    }
    n2078 = Wait (ms)(milliseconds to wait=u32 100) -> ()  [unwired: 1 out]
  }
  n2079 = while {
    stop <- FALSE stop-if-true
    n2080 = event shown="[23] \"Nolet1 disp\", \"Nolet2 disp\", \"Stroke1 disp\", \"Stroke2 disp\", \"Unforced Error1 disp\", \"Forced Error1 disp\", \"Forced Error2 disp\", \"Unforced Error2 disp\", \"Unexpected Winner1 disp\", \"Expected Winner1 disp\", \"Expected Winner2 disp\", \"Unexpected Winner2 disp\": Value Change" {
      selector: _ -> [_ _ _ _ _ _ _ _ _ _ _ _ _ _ _ _ _ _ _ _ _ _ _ _]
      dyn-events: _ -> [_ _ _ _ _ _ _ _ _ _ _ _ _ _ _ _ _ _ _ _ _ _ _ _]
      timeout: 100 -> [_ _ _ _ _ _ _ _ _ _ _ _ _ _ _ _ _ _ _ _ _ _ _ _]
      event Timeout {
        n2081 = event-data() -> ()  [unwired: 1 in, 3 out]
        n2082 = local write "fast forward"(FALSE ("fast forward")) -> ()
        n2083 = local write "fast rewind"(FALSE ("fast rewind")) -> ()
      }
      event Key Repeat {
        n2084 = event-data() -> ("VKey"=w2459:T8)  [unwired: 1 in, 9 out]
        n2085 = case shown="\"Right\"" w2459 {
          frame "ASCII", Default {
          }
          frame "Enter" {
          }
          frame "Return" {
          }
          frame "Shift" {
          }
          frame "Ctrl" {
          }
          frame "Alt" {
          }
          frame "Cmd" {
          }
          frame "Opt" {
          }
          frame "Caps" {
          }
          frame "NumLock" {
          }
          frame "Clear" {
          }
          frame "Break" {
          }
          frame "Up" {
          }
          frame "Down" {
          }
          frame "Left" {
            n2086 = local write "fast rewind"(TRUE ("fast rewind")) -> ()
          }
          frame "Right" {
            n2087 = local write "fast forward"(TRUE ("fast forward")) -> ()
          }
          frame "Insert" {
          }
          frame "Delete" {
          }
          frame "Home" {
          }
          frame "End" {
          }
          frame "PageUp" {
          }
          frame "PageDown" {
          }
          frame "Escape" {
          }
          frame "Help" {
          }
          frame "Pause" {
          }
          frame "ScrollLock" {
          }
          frame "F1" {
          }
          frame "F2" {
          }
          frame "F3" {
          }
          frame "F4" {
          }
          frame "F5" {
          }
          frame "F6" {
          }
          frame "F7" {
          }
          frame "F8" {
          }
          frame "F9" {
          }
          frame "F10" {
          }
          frame "F11" {
          }
          frame "F12" {
          }
          frame "F13" {
          }
          frame "F14" {
          }
          frame "F15" {
          }
          frame "F16" {
          }
          frame "F17" {
          }
          frame "F18" {
          }
          frame "F19" {
          }
          frame "F20" {
          }
          frame "F21" {
          }
          frame "F22" {
          }
          frame "F23" {
          }
          frame "F24" {
          }
          frame "Play" {
          }
          frame "VolumeUp" {
          }
          frame "VolumeDown" {
          }
          frame "Mute" {
          }
          frame "Two Byte Char" {
          }
        }
      }
      event Key Down {
        n2088 = event-data() -> ("Char"=w2473:i16, "VKey"=w2462:T8)  [unwired: 1 in, 8 out]
        n2089 = property on="Btn 2" class="Str"() -> ("Key Focus"=w2468:bool)  [unwired: 2 in, 2 out]
        n2090 = property on="Btn 3" class="Str"() -> ("Key Focus"=w2467:bool)  [unwired: 2 in, 2 out]
        n2091 = property on="Btn 4" class="Str"() -> ("Key Focus"=w2466:bool)  [unwired: 2 in, 2 out]
        n2092 = property on="Btn 5" class="Str"() -> ("Key Focus"=w2469:bool)  [unwired: 2 in, 2 out]
        n2093 = property on="Btn 1" class="Str"() -> ("Key Focus"=w2470:bool)  [unwired: 2 in, 2 out]
        n2094 = Equal?(x=i16 32, y=w2473) -> (x = y?=w2464:bool)
        n2095 = Compound Arithmetic op=OR(w2468, w2467, w2466, w2469, w2470) -> (w2471:bool)
        n2096 = Not(x=w2471) -> (.not. x?=w2465:bool)
        n2097 = And(x=w2464, y=w2465) -> (x .and. y?=w2463:bool)
        n2098 = case shown="\"Escape\"" w2462 {
          frame "ASCII", Default {
          }
          frame "Enter" {
          }
          frame "Return" {
          }
          frame "Shift" {
          }
          frame "Ctrl" {
          }
          frame "Alt" {
          }
          frame "Cmd" {
          }
          frame "Opt" {
          }
          frame "Caps" {
          }
          frame "NumLock" {
          }
          frame "Clear" {
          }
          frame "Break" {
          }
          frame "Up" {
          }
          frame "Down" {
          }
          frame "Left" {
          }
          frame "Right" {
          }
          frame "Insert" {
          }
          frame "Delete" {
          }
          frame "Home" {
          }
          frame "End" {
          }
          frame "PageUp" {
          }
          frame "PageDown" {
          }
          frame "Escape" {
            n2099 = local write "Undo"(TRUE ("Undo")) -> ()
          }
          frame "Help" {
          }
          frame "Pause" {
          }
          frame "ScrollLock" {
          }
          frame "F1" {
          }
          frame "F2" {
          }
          frame "F3" {
          }
          frame "F4" {
          }
          frame "F5" {
          }
          frame "F6" {
          }
          frame "F7" {
          }
          frame "F8" {
          }
          frame "F9" {
          }
          frame "F10" {
          }
          frame "F11" {
          }
          frame "F12" {
          }
          frame "F13" {
          }
          frame "F14" {
          }
          frame "F15" {
          }
          frame "F16" {
          }
          frame "F17" {
          }
          frame "F18" {
          }
          frame "F19" {
          }
          frame "F20" {
          }
          frame "F21" {
          }
          frame "F22" {
          }
          frame "F23" {
          }
          frame "F24" {
          }
          frame "Play" {
          }
          frame "VolumeUp" {
          }
          frame "VolumeDown" {
          }
          frame "Mute" {
          }
          frame "Two Byte Char" {
          }
        }
        n2100 = case shown="True" w2463 {
          frame False {
          }
          frame True {
            n2101 = local read "Pause"() -> (w2476:bool)
            n2102 = Not(x=w2476) -> (.not. x?=w2475:bool)
            n2103 = local write "Pause"(w2475) -> ()
          }
        }
      }
      event "Drive hide": Value Change {
        n2104 = event-data() -> ("NewVal"=w2477:bool)  [unwired: 1 in, 5 out]
        n2105 = case shown="False" w2477 {
          frame True {
            w2514 = TRUE ("Visible")
            w2515 = TRUE ("Visible")
            n2106 = control-ref of="ADrive"() -> (w2501:refnum<vi>)
            n2107 = control-ref of="ADrive 2"() -> (w2500:refnum<vi>)
            n2108 = control-ref of="ADrive 3"() -> (w2499:refnum<vi>)
            n2109 = control-ref of="ADrive 4"() -> (w2498:refnum<vi>)
            n2110 = control-ref of="ADrive 5"() -> (w2497:refnum<vi>)
            n2111 = control-ref of="ADrive 6"() -> (w2496:refnum<vi>)
            n2112 = control-ref of="ADrive 7"() -> (w2495:refnum<vi>)
            n2113 = control-ref of="ADrive 8"() -> (w2494:refnum<vi>)
            n2114 = control-ref of="ADrive 9"() -> (w2493:refnum<vi>)
            n2115 = control-ref of="ADrive 10"() -> (w2492:refnum<vi>)
            n2116 = control-ref of="ADrive 11"() -> (w2491:refnum<vi>)
            n2117 = control-ref of="ADrive 12"() -> (w2490:refnum<vi>)
            n2118 = property class="Bool (strict)"(reference=w2501, "Visible"=w2515) -> (error out=w2489:errorcluster)  [unwired: 1 in, 1 out]
            n2119 = property class="Bool (strict)"(reference=w2500, "Visible"=w2515) -> (error out=w2488:errorcluster)  [unwired: 1 in, 1 out]
            n2120 = property class="Bool (strict)"(reference=w2499, "Visible"=w2515) -> (error out=w2487:errorcluster)  [unwired: 1 in, 1 out]
            n2121 = property class="Bool (strict)"(reference=w2498, "Visible"=w2515) -> (error out=w2486:errorcluster)  [unwired: 1 in, 1 out]
            n2122 = property class="Bool (strict)"(reference=w2497, "Visible"=w2515) -> (error out=w2485:errorcluster)  [unwired: 1 in, 1 out]
            n2123 = property class="Bool (strict)"(reference=w2496, "Visible"=w2515) -> (error out=w2484:errorcluster)  [unwired: 1 in, 1 out]
            n2124 = property class="Bool (strict)"(reference=w2495, "Visible"=w2515) -> (error out=w2483:errorcluster)  [unwired: 1 in, 1 out]
            n2125 = property class="Bool (strict)"(reference=w2494, "Visible"=w2515) -> (error out=w2482:errorcluster)  [unwired: 1 in, 1 out]
            n2126 = property class="Bool (strict)"(reference=w2493, "Visible"=w2515) -> (error out=w2481:errorcluster)  [unwired: 1 in, 1 out]
            n2127 = property class="Bool (strict)"(reference=w2492, "Visible"=w2515) -> (error out=w2480:errorcluster)  [unwired: 1 in, 1 out]
            n2128 = property class="Bool (strict)"(reference=w2491, "Visible"=w2515) -> (error out=w2479:errorcluster)  [unwired: 1 in, 1 out]
            n2129 = property class="Bool (strict)"(reference=w2490, "Visible"=w2515) -> (error out=w2478:errorcluster)  [unwired: 1 in, 1 out]
            n2130 = control-ref of="DDrive"() -> (w2513:refnum<vi>)
            n2131 = control-ref of="DDrive 2"() -> (w2512:refnum<vi>)
            n2132 = control-ref of="DDrive 3"() -> (w2511:refnum<vi>)
            n2133 = control-ref of="DDrive 4"() -> (w2510:refnum<vi>)
            n2134 = control-ref of="DDrive 5"() -> (w2509:refnum<vi>)
            n2135 = control-ref of="DDrive 6"() -> (w2508:refnum<vi>)
            n2136 = control-ref of="DDrive 7"() -> (w2507:refnum<vi>)
            n2137 = control-ref of="DDrive 8"() -> (w2506:refnum<vi>)
            n2138 = control-ref of="DDrive 9"() -> (w2505:refnum<vi>)
            n2139 = control-ref of="DDrive 10"() -> (w2504:refnum<vi>)
            n2140 = control-ref of="DDrive 11"() -> (w2503:refnum<vi>)
            n2141 = control-ref of="DDrive 12"() -> (w2502:refnum<vi>)
            n2142 = property class="Bool (strict)"(reference=w2513, error in=w2489, "Visible"=w2514) -> ()  [unwired: 2 out]
            n2143 = property class="Bool (strict)"(reference=w2512, error in=w2488, "Visible"=w2514) -> ()  [unwired: 2 out]
            n2144 = property class="Bool (strict)"(reference=w2511, error in=w2487, "Visible"=w2514) -> ()  [unwired: 2 out]
            n2145 = property class="Bool (strict)"(reference=w2510, error in=w2486, "Visible"=w2514) -> ()  [unwired: 2 out]
            n2146 = property class="Bool (strict)"(reference=w2509, error in=w2485, "Visible"=w2514) -> ()  [unwired: 2 out]
            n2147 = property class="Bool (strict)"(reference=w2508, error in=w2484, "Visible"=w2514) -> ()  [unwired: 2 out]
            n2148 = property class="Bool (strict)"(reference=w2507, error in=w2483, "Visible"=w2514) -> ()  [unwired: 2 out]
            n2149 = property class="Bool (strict)"(reference=w2506, error in=w2482, "Visible"=w2514) -> ()  [unwired: 2 out]
            n2150 = property class="Bool (strict)"(reference=w2505, error in=w2481, "Visible"=w2514) -> ()  [unwired: 2 out]
            n2151 = property class="Bool (strict)"(reference=w2504, error in=w2480, "Visible"=w2514) -> ()  [unwired: 2 out]
            n2152 = property class="Bool (strict)"(reference=w2503, error in=w2479, "Visible"=w2514) -> ()  [unwired: 2 out]
            n2153 = property class="Bool (strict)"(reference=w2502, error in=w2478, "Visible"=w2514) -> ()  [unwired: 2 out]
          }
          frame False {
            w2552 = FALSE ("Visible")
            w2553 = FALSE ("Visible")
            n2154 = control-ref of="ADrive"() -> (w2539:refnum<vi>)
            n2155 = control-ref of="ADrive 2"() -> (w2538:refnum<vi>)
            n2156 = control-ref of="ADrive 3"() -> (w2537:refnum<vi>)
            n2157 = control-ref of="ADrive 4"() -> (w2536:refnum<vi>)
            n2158 = control-ref of="ADrive 5"() -> (w2535:refnum<vi>)
            n2159 = control-ref of="ADrive 6"() -> (w2534:refnum<vi>)
            n2160 = control-ref of="ADrive 7"() -> (w2533:refnum<vi>)
            n2161 = control-ref of="ADrive 8"() -> (w2532:refnum<vi>)
            n2162 = control-ref of="ADrive 9"() -> (w2531:refnum<vi>)
            n2163 = control-ref of="ADrive 10"() -> (w2530:refnum<vi>)
            n2164 = control-ref of="ADrive 11"() -> (w2529:refnum<vi>)
            n2165 = control-ref of="ADrive 12"() -> (w2528:refnum<vi>)
            n2166 = property class="Bool (strict)"(reference=w2539, "Visible"=w2553) -> (error out=w2527:errorcluster)  [unwired: 1 in, 1 out]
            n2167 = property class="Bool (strict)"(reference=w2538, "Visible"=w2553) -> (error out=w2526:errorcluster)  [unwired: 1 in, 1 out]
            n2168 = property class="Bool (strict)"(reference=w2537, "Visible"=w2553) -> (error out=w2525:errorcluster)  [unwired: 1 in, 1 out]
            n2169 = property class="Bool (strict)"(reference=w2536, "Visible"=w2553) -> (error out=w2524:errorcluster)  [unwired: 1 in, 1 out]
            n2170 = property class="Bool (strict)"(reference=w2535, "Visible"=w2553) -> (error out=w2523:errorcluster)  [unwired: 1 in, 1 out]
            n2171 = property class="Bool (strict)"(reference=w2534, "Visible"=w2553) -> (error out=w2522:errorcluster)  [unwired: 1 in, 1 out]
            n2172 = property class="Bool (strict)"(reference=w2533, "Visible"=w2553) -> (error out=w2521:errorcluster)  [unwired: 1 in, 1 out]
            n2173 = property class="Bool (strict)"(reference=w2532, "Visible"=w2553) -> (error out=w2520:errorcluster)  [unwired: 1 in, 1 out]
            n2174 = property class="Bool (strict)"(reference=w2531, "Visible"=w2553) -> (error out=w2519:errorcluster)  [unwired: 1 in, 1 out]
            n2175 = property class="Bool (strict)"(reference=w2530, "Visible"=w2553) -> (error out=w2518:errorcluster)  [unwired: 1 in, 1 out]
            n2176 = property class="Bool (strict)"(reference=w2529, "Visible"=w2553) -> (error out=w2517:errorcluster)  [unwired: 1 in, 1 out]
            n2177 = property class="Bool (strict)"(reference=w2528, "Visible"=w2553) -> (error out=w2516:errorcluster)  [unwired: 1 in, 1 out]
            n2178 = control-ref of="DDrive"() -> (w2551:refnum<vi>)
            n2179 = control-ref of="DDrive 2"() -> (w2550:refnum<vi>)
            n2180 = control-ref of="DDrive 3"() -> (w2549:refnum<vi>)
            n2181 = control-ref of="DDrive 4"() -> (w2548:refnum<vi>)
            n2182 = control-ref of="DDrive 5"() -> (w2547:refnum<vi>)
            n2183 = control-ref of="DDrive 6"() -> (w2546:refnum<vi>)
            n2184 = control-ref of="DDrive 7"() -> (w2545:refnum<vi>)
            n2185 = control-ref of="DDrive 8"() -> (w2544:refnum<vi>)
            n2186 = control-ref of="DDrive 9"() -> (w2543:refnum<vi>)
            n2187 = control-ref of="DDrive 10"() -> (w2542:refnum<vi>)
            n2188 = control-ref of="DDrive 11"() -> (w2541:refnum<vi>)
            n2189 = control-ref of="DDrive 12"() -> (w2540:refnum<vi>)
            n2190 = property class="Bool (strict)"(reference=w2551, error in=w2527, "Visible"=w2552) -> ()  [unwired: 2 out]
            n2191 = property class="Bool (strict)"(reference=w2550, error in=w2526, "Visible"=w2552) -> ()  [unwired: 2 out]
            n2192 = property class="Bool (strict)"(reference=w2549, error in=w2525, "Visible"=w2552) -> ()  [unwired: 2 out]
            n2193 = property class="Bool (strict)"(reference=w2548, error in=w2524, "Visible"=w2552) -> ()  [unwired: 2 out]
            n2194 = property class="Bool (strict)"(reference=w2547, error in=w2523, "Visible"=w2552) -> ()  [unwired: 2 out]
            n2195 = property class="Bool (strict)"(reference=w2546, error in=w2522, "Visible"=w2552) -> ()  [unwired: 2 out]
            n2196 = property class="Bool (strict)"(reference=w2545, error in=w2521, "Visible"=w2552) -> ()  [unwired: 2 out]
            n2197 = property class="Bool (strict)"(reference=w2544, error in=w2520, "Visible"=w2552) -> ()  [unwired: 2 out]
            n2198 = property class="Bool (strict)"(reference=w2543, error in=w2519, "Visible"=w2552) -> ()  [unwired: 2 out]
            n2199 = property class="Bool (strict)"(reference=w2542, error in=w2518, "Visible"=w2552) -> ()  [unwired: 2 out]
            n2200 = property class="Bool (strict)"(reference=w2541, error in=w2517, "Visible"=w2552) -> ()  [unwired: 2 out]
            n2201 = property class="Bool (strict)"(reference=w2540, error in=w2516, "Visible"=w2552) -> ()  [unwired: 2 out]
          }
        }
      }
      event "SWDrive hide": Value Change {
        n2202 = event-data() -> ("NewVal"=w2554:bool)  [unwired: 1 in, 5 out]
        n2203 = case shown="True" w2554 {
          frame True {
            w2592 = TRUE ("Visible")
            w2591 = TRUE ("Visible")
            n2204 = control-ref of="SWDDrive"() -> (w2590:refnum<vi>)
            n2205 = control-ref of="SWDDrive 2"() -> (w2589:refnum<vi>)
            n2206 = control-ref of="SWDDrive 3"() -> (w2588:refnum<vi>)
            n2207 = control-ref of="SWDDrive 4"() -> (w2587:refnum<vi>)
            n2208 = control-ref of="SWDDrive 5"() -> (w2586:refnum<vi>)
            n2209 = control-ref of="SWDDrive 6"() -> (w2585:refnum<vi>)
            n2210 = control-ref of="SWDDrive 7"() -> (w2584:refnum<vi>)
            n2211 = control-ref of="SWDDrive 8"() -> (w2583:refnum<vi>)
            n2212 = control-ref of="SWDDrive 9"() -> (w2582:refnum<vi>)
            n2213 = control-ref of="SWDDrive 10"() -> (w2581:refnum<vi>)
            n2214 = control-ref of="SWDDrive 11"() -> (w2580:refnum<vi>)
            n2215 = control-ref of="SWDDrive 12"() -> (w2579:refnum<vi>)
            n2216 = property class="Bool (strict)"(reference=w2590, "Visible"=w2592) -> (error out=w2566:errorcluster)  [unwired: 1 in, 1 out]
            n2217 = property class="Bool (strict)"(reference=w2589, "Visible"=w2592) -> (error out=w2565:errorcluster)  [unwired: 1 in, 1 out]
            n2218 = property class="Bool (strict)"(reference=w2588, "Visible"=w2592) -> (error out=w2564:errorcluster)  [unwired: 1 in, 1 out]
            n2219 = property class="Bool (strict)"(reference=w2587, "Visible"=w2592) -> (error out=w2563:errorcluster)  [unwired: 1 in, 1 out]
            n2220 = property class="Bool (strict)"(reference=w2586, "Visible"=w2592) -> (error out=w2562:errorcluster)  [unwired: 1 in, 1 out]
            n2221 = property class="Bool (strict)"(reference=w2585, "Visible"=w2592) -> (error out=w2561:errorcluster)  [unwired: 1 in, 1 out]
            n2222 = property class="Bool (strict)"(reference=w2584, "Visible"=w2592) -> (error out=w2560:errorcluster)  [unwired: 1 in, 1 out]
            n2223 = property class="Bool (strict)"(reference=w2583, "Visible"=w2592) -> (error out=w2559:errorcluster)  [unwired: 1 in, 1 out]
            n2224 = property class="Bool (strict)"(reference=w2582, "Visible"=w2592) -> (error out=w2558:errorcluster)  [unwired: 1 in, 1 out]
            n2225 = property class="Bool (strict)"(reference=w2581, "Visible"=w2592) -> (error out=w2557:errorcluster)  [unwired: 1 in, 1 out]
            n2226 = property class="Bool (strict)"(reference=w2580, "Visible"=w2592) -> (error out=w2556:errorcluster)  [unwired: 1 in, 1 out]
            n2227 = property class="Bool (strict)"(reference=w2579, "Visible"=w2592) -> (error out=w2555:errorcluster)  [unwired: 1 in, 1 out]
            n2228 = control-ref of="SWADrive"() -> (w2578:refnum<vi>)
            n2229 = control-ref of="SWADrive 2"() -> (w2577:refnum<vi>)
            n2230 = control-ref of="SWADrive 3"() -> (w2576:refnum<vi>)
            n2231 = control-ref of="SWADrive 4"() -> (w2575:refnum<vi>)
            n2232 = control-ref of="SWADrive 5"() -> (w2574:refnum<vi>)
            n2233 = control-ref of="SWADrive 6"() -> (w2573:refnum<vi>)
            n2234 = control-ref of="SWADrive 7"() -> (w2572:refnum<vi>)
            n2235 = control-ref of="SWADrive 8"() -> (w2571:refnum<vi>)
            n2236 = control-ref of="SWADrive 9"() -> (w2570:refnum<vi>)
            n2237 = control-ref of="SWADrive 10"() -> (w2569:refnum<vi>)
            n2238 = control-ref of="SWADrive 11"() -> (w2568:refnum<vi>)
            n2239 = control-ref of="SWADrive 12"() -> (w2567:refnum<vi>)
            n2240 = property class="Bool (strict)"(reference=w2578, error in=w2566, "Visible"=w2591) -> ()  [unwired: 2 out]
            n2241 = property class="Bool (strict)"(reference=w2577, error in=w2565, "Visible"=w2591) -> ()  [unwired: 2 out]
            n2242 = property class="Bool (strict)"(reference=w2576, error in=w2564, "Visible"=w2591) -> ()  [unwired: 2 out]
            n2243 = property class="Bool (strict)"(reference=w2575, error in=w2563, "Visible"=w2591) -> ()  [unwired: 2 out]
            n2244 = property class="Bool (strict)"(reference=w2574, error in=w2562, "Visible"=w2591) -> ()  [unwired: 2 out]
            n2245 = property class="Bool (strict)"(reference=w2573, error in=w2561, "Visible"=w2591) -> ()  [unwired: 2 out]
            n2246 = property class="Bool (strict)"(reference=w2572, error in=w2560, "Visible"=w2591) -> ()  [unwired: 2 out]
            n2247 = property class="Bool (strict)"(reference=w2571, error in=w2559, "Visible"=w2591) -> ()  [unwired: 2 out]
            n2248 = property class="Bool (strict)"(reference=w2570, error in=w2558, "Visible"=w2591) -> ()  [unwired: 2 out]
            n2249 = property class="Bool (strict)"(reference=w2569, error in=w2557, "Visible"=w2591) -> ()  [unwired: 2 out]
            n2250 = property class="Bool (strict)"(reference=w2568, error in=w2556, "Visible"=w2591) -> ()  [unwired: 2 out]
            n2251 = property class="Bool (strict)"(reference=w2567, error in=w2555, "Visible"=w2591) -> ()  [unwired: 2 out]
          }
          frame False {
            w2630 = FALSE ("Visible")
            w2629 = FALSE ("Visible")
            n2252 = control-ref of="SWDDrive"() -> (w2628:refnum<vi>)
            n2253 = control-ref of="SWDDrive 2"() -> (w2627:refnum<vi>)
            n2254 = control-ref of="SWDDrive 3"() -> (w2626:refnum<vi>)
            n2255 = control-ref of="SWDDrive 4"() -> (w2625:refnum<vi>)
            n2256 = control-ref of="SWDDrive 5"() -> (w2624:refnum<vi>)
            n2257 = control-ref of="SWDDrive 6"() -> (w2623:refnum<vi>)
            n2258 = control-ref of="SWDDrive 7"() -> (w2622:refnum<vi>)
            n2259 = control-ref of="SWDDrive 8"() -> (w2621:refnum<vi>)
            n2260 = control-ref of="SWDDrive 9"() -> (w2620:refnum<vi>)
            n2261 = control-ref of="SWDDrive 10"() -> (w2619:refnum<vi>)
            n2262 = control-ref of="SWDDrive 11"() -> (w2618:refnum<vi>)
            n2263 = control-ref of="SWDDrive 12"() -> (w2617:refnum<vi>)
            n2264 = property class="Bool (strict)"(reference=w2628, "Visible"=w2630) -> (error out=w2604:errorcluster)  [unwired: 1 in, 1 out]
            n2265 = property class="Bool (strict)"(reference=w2627, "Visible"=w2630) -> (error out=w2603:errorcluster)  [unwired: 1 in, 1 out]
            n2266 = property class="Bool (strict)"(reference=w2626, "Visible"=w2630) -> (error out=w2602:errorcluster)  [unwired: 1 in, 1 out]
            n2267 = property class="Bool (strict)"(reference=w2625, "Visible"=w2630) -> (error out=w2601:errorcluster)  [unwired: 1 in, 1 out]
            n2268 = property class="Bool (strict)"(reference=w2624, "Visible"=w2630) -> (error out=w2600:errorcluster)  [unwired: 1 in, 1 out]
            n2269 = property class="Bool (strict)"(reference=w2623, "Visible"=w2630) -> (error out=w2599:errorcluster)  [unwired: 1 in, 1 out]
            n2270 = property class="Bool (strict)"(reference=w2622, "Visible"=w2630) -> (error out=w2598:errorcluster)  [unwired: 1 in, 1 out]
            n2271 = property class="Bool (strict)"(reference=w2621, "Visible"=w2630) -> (error out=w2597:errorcluster)  [unwired: 1 in, 1 out]
            n2272 = property class="Bool (strict)"(reference=w2620, "Visible"=w2630) -> (error out=w2596:errorcluster)  [unwired: 1 in, 1 out]
            n2273 = property class="Bool (strict)"(reference=w2619, "Visible"=w2630) -> (error out=w2595:errorcluster)  [unwired: 1 in, 1 out]
            n2274 = property class="Bool (strict)"(reference=w2618, "Visible"=w2630) -> (error out=w2594:errorcluster)  [unwired: 1 in, 1 out]
            n2275 = property class="Bool (strict)"(reference=w2617, "Visible"=w2630) -> (error out=w2593:errorcluster)  [unwired: 1 in, 1 out]
            n2276 = control-ref of="SWADrive"() -> (w2616:refnum<vi>)
            n2277 = control-ref of="SWADrive 2"() -> (w2615:refnum<vi>)
            n2278 = control-ref of="SWADrive 3"() -> (w2614:refnum<vi>)
            n2279 = control-ref of="SWADrive 4"() -> (w2613:refnum<vi>)
            n2280 = control-ref of="SWADrive 5"() -> (w2612:refnum<vi>)
            n2281 = control-ref of="SWADrive 6"() -> (w2611:refnum<vi>)
            n2282 = control-ref of="SWADrive 7"() -> (w2610:refnum<vi>)
            n2283 = control-ref of="SWADrive 8"() -> (w2609:refnum<vi>)
            n2284 = control-ref of="SWADrive 9"() -> (w2608:refnum<vi>)
            n2285 = control-ref of="SWADrive 10"() -> (w2607:refnum<vi>)
            n2286 = control-ref of="SWADrive 11"() -> (w2606:refnum<vi>)
            n2287 = control-ref of="SWADrive 12"() -> (w2605:refnum<vi>)
            n2288 = property class="Bool (strict)"(reference=w2616, error in=w2604, "Visible"=w2629) -> ()  [unwired: 2 out]
            n2289 = property class="Bool (strict)"(reference=w2615, error in=w2603, "Visible"=w2629) -> ()  [unwired: 2 out]
            n2290 = property class="Bool (strict)"(reference=w2614, error in=w2602, "Visible"=w2629) -> ()  [unwired: 2 out]
            n2291 = property class="Bool (strict)"(reference=w2613, error in=w2601, "Visible"=w2629) -> ()  [unwired: 2 out]
            n2292 = property class="Bool (strict)"(reference=w2612, error in=w2600, "Visible"=w2629) -> ()  [unwired: 2 out]
            n2293 = property class="Bool (strict)"(reference=w2611, error in=w2599, "Visible"=w2629) -> ()  [unwired: 2 out]
            n2294 = property class="Bool (strict)"(reference=w2610, error in=w2598, "Visible"=w2629) -> ()  [unwired: 2 out]
            n2295 = property class="Bool (strict)"(reference=w2609, error in=w2597, "Visible"=w2629) -> ()  [unwired: 2 out]
            n2296 = property class="Bool (strict)"(reference=w2608, error in=w2596, "Visible"=w2629) -> ()  [unwired: 2 out]
            n2297 = property class="Bool (strict)"(reference=w2607, error in=w2595, "Visible"=w2629) -> ()  [unwired: 2 out]
            n2298 = property class="Bool (strict)"(reference=w2606, error in=w2594, "Visible"=w2629) -> ()  [unwired: 2 out]
            n2299 = property class="Bool (strict)"(reference=w2605, error in=w2593, "Visible"=w2629) -> ()  [unwired: 2 out]
          }
        }
      }
      event "Adrive disp", "Adrive disp 2": Value Change {
        n2300 = event-data() -> ("NewVal"=w2631:bool)  [unwired: 1 in, 5 out]
        n2301 = local write "Adrive disp 2"(w2631) -> ()
        n2302 = local write "Adrive"(w2631) -> ()
        n2303 = local write "Adrive disp"(w2631) -> ()
      }
      event "Ddrive disp", "Ddrive disp 2": Value Change {
        n2304 = event-data() -> ("NewVal"=w2632:bool)  [unwired: 1 in, 5 out]
        n2305 = local write "Ddrive"(w2632) -> ()
        n2306 = local write "Ddrive disp 2"(w2632) -> ()
        n2307 = local write "Ddrive disp"(w2632) -> ()
      }
      event "ASWdrive disp", "ASWdrive disp 2": Value Change {
        n2308 = event-data() -> ("NewVal"=w2633:bool)  [unwired: 1 in, 5 out]
        n2309 = local write "ASWdrive"(w2633) -> ()
        n2310 = local write "ASWdrive disp"(w2633) -> ()
        n2311 = local write "ASWdrive disp 2"(w2633) -> ()
      }
      event "DSWdrive disp", "DSWdrive disp 2": Value Change {
        n2312 = event-data() -> ("NewVal"=w2634:bool)  [unwired: 1 in, 5 out]
        n2313 = local write "DSWdrive disp 2"(w2634) -> ()
        n2314 = local write "DSWdrive disp"(w2634) -> ()
        n2315 = local write "DSWdrive"(w2634) -> ()
      }
      event "Drop disp", "Drop disp 2": Value Change {
        n2316 = event-data() -> ("NewVal"=w2635:bool)  [unwired: 1 in, 5 out]
        n2317 = local write "Drop disp 2"(w2635) -> ()
        n2318 = local write "Drop disp"(w2635) -> ()
        n2319 = local write "Drop 14"(w2635) -> ()
      }
      event "Chop disp", "Chop disp 2": Value Change {
        n2320 = event-data() -> ("NewVal"=w2636:bool)  [unwired: 1 in, 5 out]
        n2321 = local write "Chop disp 2"(w2636) -> ()
        n2322 = local write "Chop 13"(w2636) -> ()
        n2323 = local write "Chop disp"(w2636) -> ()
      }
      event "Lob disp", "Lob disp 2": Value Change {
        n2324 = event-data() -> ("NewVal"=w2637:bool)  [unwired: 1 in, 5 out]
        n2325 = local write "Lob disp 2"(w2637) -> ()
        n2326 = local write "Lob disp"(w2637) -> ()
        n2327 = local write "Lob"(w2637) -> ()
      }
      event "Boast2 disp", "Boast2 disp 2": Value Change {
        n2328 = event-data() -> ("NewVal"=w2638:bool)  [unwired: 1 in, 5 out]
        n2329 = local write "Boast2 disp 2"(w2638) -> ()
        n2330 = local write "Boast2"(w2638) -> ()
        n2331 = local write "Boast2 disp"(w2638) -> ()
      }
      event "Boast3 disp", "Boast3 disp 2": Value Change {
        n2332 = event-data() -> ("NewVal"=w2639:bool)  [unwired: 1 in, 5 out]
        n2333 = local write "Boast3 disp"(w2639) -> ()
        n2334 = local write "Boast3 disp 2"(w2639) -> ()
        n2335 = local write "Boast3"(w2639) -> ()
      }
      event "Smash disp", "Smash disp 2": Value Change {
        n2336 = event-data() -> ("NewVal"=w2640:bool)  [unwired: 1 in, 5 out]
        n2337 = local write "Smash disp 2"(w2640) -> ()
        n2338 = local write "Smash 13"(w2640) -> ()
        n2339 = local write "Smash disp"(w2640) -> ()
      }
      event "Let disp", "Let disp 2": Value Change {
        n2340 = event-data() -> ("NewVal"=w2641:bool)  [unwired: 1 in, 5 out]
        n2341 = local write "Let 2"(w2641) -> ()
        n2342 = local write "Let disp 2"(w2641) -> ()
        n2343 = local write "Let disp"(w2641) -> ()
      }
      event "Forehand disp 1", "Forehand disp 2": Value Change {
        n2344 = event-data() -> ("NewVal"=w2642:bool)  [unwired: 1 in, 5 out]
        n2345 = local write "Forehand disp 1"(w2642) -> ()
        n2346 = local write "Forehand disp 2"(w2642) -> ()
        n2347 = local write "FH"(w2642) -> ()
      }
      event "Backhand disp 1", "Backhand disp 2": Value Change {
        n2348 = event-data() -> ("NewVal"=w2643:bool)  [unwired: 1 in, 5 out]
        n2349 = local write "Backhand disp 1"(w2643) -> ()
        n2350 = local write "Backhand disp 2"(w2643) -> ()
        n2351 = local write "BH"(w2643) -> ()
      }
      event "Straight disp 1", "Straight disp 2": Value Change {
        n2352 = event-data() -> ("NewVal"=w2644:bool)  [unwired: 1 in, 5 out]
        n2353 = local write "Straight disp 1"(w2644) -> ()
        n2354 = local write "Straight disp 2"(w2644) -> ()
        n2355 = local write "ST"(w2644) -> ()
      }
      event "Cross disp 1", "Cross disp 2": Value Change {
        n2356 = event-data() -> ("NewVal"=w2645:bool)  [unwired: 1 in, 5 out]
        n2357 = local write "Cross disp 2"(w2645) -> ()
        n2358 = local write "Cross disp 1"(w2645) -> ()
        n2359 = local write "CR"(w2645) -> ()
      }
      event "Bounce disp 1", "Bounce disp 2": Value Change {
        n2360 = event-data() -> ("NewVal"=w2646:bool)  [unwired: 1 in, 5 out]
        n2361 = local write "Bounce disp 1"(w2646) -> ()
        n2362 = local write "Bounce disp 2"(w2646) -> ()
        n2363 = local write "Bounce"(w2646) -> ()
      }
      event "halfvolley disp 1", "halfvolley disp 2": Value Change {
        n2364 = event-data() -> ("NewVal"=w2647:bool)  [unwired: 1 in, 5 out]
        n2365 = local write "halfvolley disp 2"(w2647) -> ()
        n2366 = local write "halfvolley disp 1"(w2647) -> ()
        n2367 = local write "Half Volley"(w2647) -> ()
      }
      event "volley disp 1", "volley disp 2": Value Change {
        n2368 = event-data() -> ("NewVal"=w2648:bool)  [unwired: 1 in, 5 out]
        n2369 = local write "volley disp 1"(w2648) -> ()
        n2370 = local write "Volley"(w2648) -> ()
        n2371 = local write "volley disp 2"(w2648) -> ()
      }
      event "Nolet1 disp", "Nolet2 disp", "Stroke1 disp", "Stroke2 disp", "Unforced Error1 disp", "Forced Error1 disp", "Forced Error2 disp", "Unforced Error2 disp", "Unexpected Winner1 disp", "Expected Winner1 disp", "Expected Winner2 disp", "Unexpected Winner2 disp": Value Change {
        n2372 = event-data() -> ()  [unwired: 1 in, 6 out]
        n2373 = local write "Nolet2 2"("Nolet2 disp") -> ()
        n2374 = local write "Nolet1 2"("Nolet1 disp") -> ()
        n2375 = local write "Stroke2 2"("Stroke2 disp") -> ()
        n2376 = local write "Stroke1 2"("Stroke1 disp") -> ()
        n2377 = local write "Unforced Error2 2"("Unforced Error2 disp") -> ()
        n2378 = local write "Forced Error2 2"("Forced Error2 disp") -> ()
        n2379 = local write "Unforced Error1 2"("Unforced Error1 disp") -> ()
        n2380 = local write "Forced Error1 2"("Forced Error1 disp") -> ()
        n2381 = local write "Unexpected Winner2 2"("Unexpected Winner2 disp") -> ()
        n2382 = local write "Unexpected Winner1 2"("Unexpected Winner1 disp") -> ()
        n2383 = local write "Expected Winner2 2"("Expected Winner2 disp") -> ()
        n2384 = local write "Expected Winner1 2"("Expected Winner1 disp") -> ()
      }
    }
  }
  n2385 = disable-structure shown="Disabled" {
    frame Disabled {
      n2386 = local read "Lob disp 2"() -> ()  [unwired: 1 in]
      n2387 = local read "Adrive disp 2"() -> ()  [unwired: 1 in]
      n2388 = local read "Smash disp 2"() -> ()  [unwired: 1 in]
      n2389 = local read "Ddrive disp 2"() -> ()  [unwired: 1 in]
      n2390 = local read "Chop disp 2"() -> ()  [unwired: 1 in]
      n2391 = local read "Drop disp 2"() -> ()  [unwired: 1 in]
      n2392 = local read "Boast2 disp 2"() -> ()  [unwired: 1 in]
      n2393 = local read "Boast3 disp 2"() -> ()  [unwired: 1 in]
      n2394 = local read "Smash 13"() -> ()  [unwired: 1 in]
      n2395 = local read "Boast3"() -> ()  [unwired: 1 in]
      n2396 = local read "Lob"() -> ()  [unwired: 1 in]
      n2397 = local read "Chop 13"() -> ()  [unwired: 1 in]
      n2398 = local read "Boast2"() -> ()  [unwired: 1 in]
      n2399 = local read "Ddrive"() -> ()  [unwired: 1 in]
      n2400 = local read "Drop 14"() -> ()  [unwired: 1 in]
      n2401 = local read "Adrive"() -> ()  [unwired: 1 in]
      n2402 = local read "Lob disp"() -> ()  [unwired: 1 in]
      n2403 = local read "Adrive disp"() -> ()  [unwired: 1 in]
      n2404 = local read "Chop disp"() -> ()  [unwired: 1 in]
      n2405 = local read "ASWdrive disp"() -> ()  [unwired: 1 in]
      n2406 = local read "Boast3 disp"() -> ()  [unwired: 1 in]
      n2407 = local read "Boast2 disp"() -> ()  [unwired: 1 in]
      n2408 = local read "Ddrive disp"() -> ()  [unwired: 1 in]
      n2409 = local read "Smash disp"() -> ()  [unwired: 1 in]
    }
    frame Enabled {
    }
  }
